vi "Interface.vi"() -> ()   [LabVIEW 2013]
uses:
  MeasureModeControl.ctl
  <vilib>/Utility/miscctls.llb/LVBoundsTypeDef.ctl
  GlobalVariables/LanguagesSettings.vi
  GlobalVariables/PreconfiguredSleeveData.vi
  GlobalVariables/CaptParameters.vi
  GlobalVariables/ValveParameters.vi
  GlobalVariables/MachineInfos.vi
  GlobalVariables/StabilizationSettings.vi
  GlobalVariables/CalibrationVolumes.vi
  GlobalVariables/HardwarePresent.vi
  GlobalVariables/ValveValues.vi
  GlobalVariables/AppState.vi
  GlobalVariables/PressureAndTimeSamples.vi
  GlobalVariables/CurrentPressure.vi
  GlobalVariables/CommunicationActivity.vi
  GlobalVariables/CalibrationState.vi
  GlobalVariables/FittedCurvePolynom.vi
  <vilib>/Utility/file.llb/Write To Spreadsheet File (string).vi
  <vilib>/Utility/file.llb/Read From Spreadsheet File (string).vi
  GlobalVariables/MeasureExportStrings.vi
  <vilib>/Utility/config.llb/Read Key (String).vi
  GlobalVariables/UserInfos.vi
  <vilib>/Utility/config.llb/NI_LVConfig.lvlib
panel:
  in  "DeleteMeasureLine":bool
  in  "ExportData":bool
  in  "LoadData":bool
  in  "SaveData":bool
  in  "ReloadResultTableTexts":bool
  in  "MeasureMode":T1
  in  "ReloadDiskVolumes":bool
  in  "StabilityAchieved":bool
  in  "UpdateServiceGraph":bool
  in  "ComputeCalibrationResult":bool
  in  "SingleCalibrationMeasureButtonsVisible":bool
  out "FirstGraphSampleIndex":i32
  in  "ServiceButtonsVisible":bool
  in  "ExportMeasuresButtonsVisible":bool
  in  "ChangeMenuState":bool
  in  "MeasureIndicatorsVisible":bool
  in  "MeasureSetupButtonsVisible":bool
  in  "CalibrationButtonsVisible":bool
  in  "CalibrationResultsVisible":bool
  in  "UserFilledDataChanged":bool
  out "NotificationTexts":string[](array[string])
  out "rPressionM":dbl caption="Pression courante" format="%#.1f bars"
  out "error out":errorcluster caption="sortie d'erreur"
  out "indicateurPerteSignal":bool caption="Perte du signal de pression"
  out "indicateurDefautPuissance":bool caption="Défaut de puissance"
  out "indicateurSurpression":bool caption="Surpression"
  in  "btnExit":bool
  out "vTimeDate":timestamp format="%<%.1X\n%x>T"
  out "strInstallName":string="INSTALL NAME"
  in  "AppTab":T2(tab) caption="Onglets1"
  out "presentationPicture":picture caption="Prêt"
  in  "MeasuresTabs":enum32{"Grain measures", "Pore measures"}(tab) caption="Measures"
  in  "LoadGrainMeasuresBtn":bool
  in  "SaveGrainMeasuresBtn":bool caption="SaveDataFileButton"
  in  "ExportGrainMeasuresBtn":bool caption="Exporter"
  in  "ClearGrainMeasuresBtn":bool caption="Clear measures table"
  out "grainMeasuresTable":string[][](table)=[["Date", "Numéro", "ID de l'échantillon", "Profondeur (coudées)", "Poids à sec (g)", "Volume de grain (cm3)", "Densité de grain (g/cm3)", "Volume de pore (cm3)", "Porosité (%)", "Volume de l'enveloppe (cm3)", "Longueur (cm)", "Diamètre (cm)", "Epaisseur (cm)", "Température (°C)", "Commentaires"]] caption="Résultats Mesures de grains"
  in  "ClearGrainMeasureBtn":bool
  in  "LoadPoreMeasuresBtn":bool
  in  "SavePoreMeasuresBtn":bool caption="SaveDataFileButton"
  in  "ExportPoreMeasuresBtn":bool caption="Exporter"
  out "poreMeasuresTable":string[][](table)=[["Date", "Numéro", "ID de l'échantillon", "Profondeur (coudées)", "Poids à sec (g)", "Volume de grain (cm3)", "Densité de grain (g/cm3)", "Volume de pore (cm3)", "Porosité (%)", "Volume de l'enveloppe (cm3)", "Longueur (cm)", "Diamètre (cm)", "Epaisseur (cm)", "Température (°C)", "Commentaires"]] caption="Résultats"
  in  "ClearPoreMeasuresBtn":bool caption="Clear measures table"
  in  "ClearPoreMeasureBtn":bool
  in  "btnMesureGrain":bool
  out "MeasureTotalAddedVolume":dbl caption="Volume total"
  in  "MeasureDiskSet":i32(listbox) caption="Jeu de disques"
  in  "MeasureDiskVolumes":i32[](listbox) caption="Volumes disponibles"
  in  "Comments":string caption="Commentaires"
  in  "Temperature":dbl caption="Température (°C)"
  in  "BulkVolume":dbl caption="Volume de grain (cm3)"
  in  "DryWeight":dbl caption="Poids à sec (g)"
  in  "SampleDepth":dbl caption="Profondeur (cm)"
  in  "SampleID":string caption="ID de l'échantillon"
  in  "SampleNumber":string caption="Numéro"
  in  "DoMeasureMeasure":bool caption="LaunchMeasureMeasure"
  in  "ReferenceCellMeasure":u16=1 caption="Cellule de référence" min=1 max=2
  in  "DiskSet":i32(listbox) caption="Jeu de disques"
  in  "RestartCalibration":bool
  out "CalibrationStep":u32 caption="Nombre de mesures effectuées"
  in  "CalibrationFilePath":path caption="Fichier de calibration"
  in  "LoadCalibrationFileBtn":bool
  in  "AvalaibleVolumesList":i32[](listbox) caption="Volumes disponibles"
  in  "ChosenVolume":dbl caption="Volume total"
  in  "DoMeasureCalibration":bool caption="DoCalibrationMeasure"
  in  "EndCalibration":bool caption="Finir la calibration"
  out "measureStabilization":string
  in  "P1P2RatioMeasure":dbl caption="P1/P2 ratio"
  out "MeasureReportedString":string
  out "VolumeMeasureInd":dbl caption="Volume de grain mesuré"
  out "calibrationStabilization":string
  in  "KeepCalibrationPoint":bool caption="Garder le point"
  out "VolumeOfCalibrationMeasure":dbl caption="Volume total"
  out "P1P2RatioCalibration":dbl caption="Rapport P1/P2"
  in  "ContinueCalibration":bool
  out "Correlation":dbl
  out "AverageAbsoluteDeviation":dbl caption="Deviation moyenne"
  in  "SaveCalibrationFile":bool caption="Save calibration file"
  out "ResidueInd":dbl caption="Résidu"
  out "FittedPolynomCoeffs":dbl[](array[numeric]) caption="Coefficient du polynome d'interpolation"
  in  "ExportToPDF":bool caption="Export to PDF"
  in  "ExportToHTMLBtn":bool
  in  "Client":string
  in  "Country":string caption="Pays"
  in  "Formation":string
  in  "LatitudeLongitude":string caption="Latitude/Longitude"
  in  "Operator":string caption="Opérateur"
  in  "Well":string caption="Puits"
  in  "Lab":string caption="Laboratoire"
  in  "Company":string caption="Entreprise"
  in  "Field":string caption="Champs"
  in  "Location":string caption="Lieu"
  out "PurgeState":string
  out "ValvesBoutonVisible":bool=TRUE caption="Sample valve"
  in  "FlushPressureGraph":bool
  in  "Sample ValveBtn":bool=TRUE caption="Sample valve"
  in  "V2Btn":bool=TRUE caption="V2"
  in  "V1Btn":bool=TRUE caption="V1"
  in  "Inlet ValveBtn":bool=TRUE caption="Inlet valve"
  in  "Outlet ValveBtn":bool=TRUE caption="Outlet valve"
  out "PressureGraph":T3(graph)
  out "Helium Tank":string caption="Bonbonne d'Hélium"
  out "NotificationArea":string
  out "Ref2":string caption="Référence 2"
  out "Matrix Cup":string caption="Echantillon"
  out "Ref1":string caption="Référence 1"
  in  "manualModeBtn":bool
  out "Outlet ValveInd":bool=TRUE caption="Valve de sortie"
  out "Sample ValveInd":bool=TRUE caption="Valve de l'échantillon"
  out "V2Ind":bool=TRUE caption="V2"
  out "V1Ind":bool=TRUE caption="V1"
  out "Inlet ValveInd":bool=TRUE caption="Valve d'entrée"
  out "vPressionM":dbl format="%#.1f bars"
  in  "btnVidanger":bool
  in  "btnEtal":bool
  in  "btnMesurePore":bool
  in  "MaximalWaitTime":u32 caption="Temps maximal d'attente (ms)"
  in  "VarianceTrigger":dbl caption="Variance minimale"
  in  "MinimalWaitTime":u32 caption="Temps minimal d'attente (ms)"
  in  "PressureCaptorConfig":T4 caption="Configuration du capteur"
  in  "mdpControl":string caption="Mot de passe"
  in  "SamplesMasks":bool[](array[boolean]) caption="Prise en compte point n°"
  in  "CalibrationVolumesTable":string[][](table) caption="Tableau des volumes de calibrations"
  out "AverageAbsoluteDeviationServices":dbl caption="Deviation moyenne"
  out "CorrelationServices":dbl caption="Correlation"
  out "ResiduServices":dbl caption="Résidu"
  out "FittedPolynomCoeffsServices":dbl[](array[numeric]) caption="Coefficient du polynome d'interpolation"
  out "XYGraphService":cluster{dbl[], dbl[]}[](graph)=[{[1.0, 2.0, 4.0], [2.0, 1.0, 0.0]}, {[0.5, 1.5, 3.5], [3.0, 4.0, 2.0]}] caption="Mesure et courbe d'étalonnage"
  out "pumeActive":bool caption="PUM-E actif"
  out "pressureCaptorActive":bool caption="Capteur de pression actif"
  in  "MachineName":string caption="Nom de la machine"
  in  "Pressure Gain":dbl=1.0 caption="Gain de pression"
  in  "Pressure Offset":dbl caption="Offset de pression"
  in  "Valve mapping":T5 caption="Mappage des valves"
  in  "LanguagesList":i32(listbox) caption="Langues disponibles"
  in  "SaveConfigChanges":bool caption="Save changes"
  in  "SleeveConfiguration":T6 caption="Configuration de la chemise"
  in  "ValvesConfig":T7 caption="Configuration des valves" {"Mode" items=["RTU", "ASCII"]}
  # "Stabilisation"
  # "Services"
  # "Transmission"
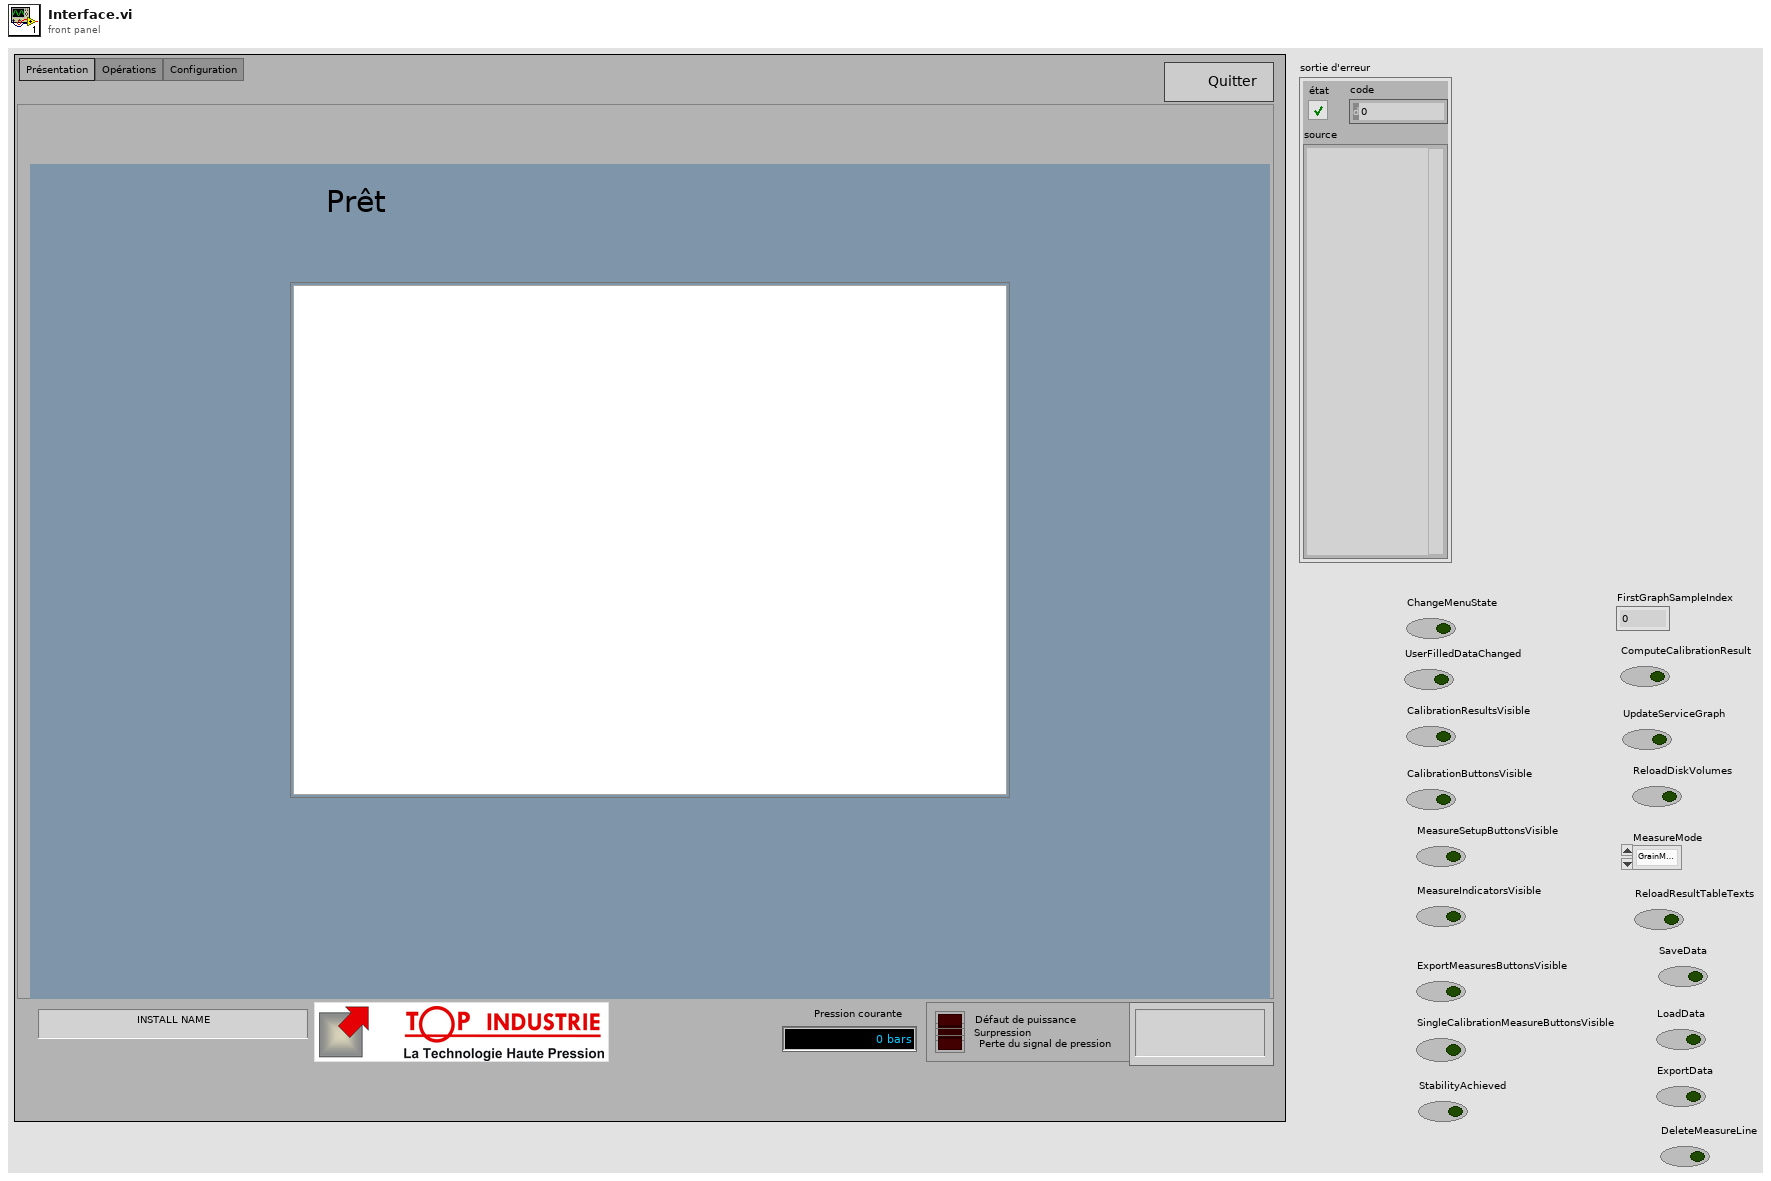
[diagram p1: front panel]
types:
  T1 = typedef "MeasureModeControl.ctl" = enum16{"GrainMeasure", "PoreMeasure"}
  T2 = enum32{"Présentation", "Opérations", "Configuration"}
  T3 = cluster{"TimeSamples":dbl[], "PressureSamples":dbl[]}
  T4 = cluster{"Baudrate":u32, "Port":string, "Databits":u16, "Parity":u16, "Stopbits":u16, "Flow Control":u16, "Slave Address":u16, "Register Address":u16, "Timeout (ms)":u16, "MaxCaptorPressure":dbl}
  T5 = cluster{"Inlet Valve":u8, "V1":u8, "V2":u8, "Sample Valve":u8, "Outlet Valve":u8}
  T6 = cluster{"Length (cm)":dbl, "Diameter (cm)":dbl, "Thickness (cm)":dbl}
  T7 = cluster{"Baudrate":u32, "Port":string, "Databits":u16, "Parity":u16, "Stopbits":u16, "Flow Control":u16, "Slave Address":u16, "Mode":u16, "Timeout (ms)":u16}
  T8 = enum8{"Enabled", "Disabled", "Disabled and Grayed Out"}
  T9 = cluster{bool, "CalibrationStep":u32, "Volumes":dbl[], "PressureRatios":dbl[], "Weights":bool[]}
  T10 = typedef "LVBoundsTypeDef.ctl" = cluster{"Width":u32, "Height":u32}
  T11 = cluster{"baudrate":u32, "databits":u16, "paritybit":u16, "stopbits":u16, "flux control":u16, "Port":string, "Serial Parameters":cluster{"Mode":enum16{"RTU", "ASCII"}, "Slave Address":u8}, "Timeout":u32, "Valve mapping":cluster{"Inlet Valve":u8, "V1":u8, "V2":u8, "Sample Valve":u8, "Outlet Valve":u8}}
  T12 = cluster{"baudrate":u32, "databits":u16, "paritybit":u16, "stopbits":u16, "flux control":u16, "Port":string, "Register Address":u16, "Serial Parameters":cluster{"Mode":enum16{"RTU", "ASCII"}, "Slave Address":u8}, "Timeout":u32, "PressureLimit":dbl}
  T13 = cluster{"SupportedLanguagesList":string[], "ActiveLanguage":string, "ActiveLanguageIndex":u16, "LocalisationFileContent[out]":cluster{"Indices":u32[], "LocalizedWords":string[][]}}
  T14 = cluster{"SerialNumber":string, "MachineName":string}
  T15 = cluster{"sleeveLength":dbl, "sleeveDiameter":dbl, "sleeveThickness":dbl}
  T16 = cluster{"baudrate":u32, "Port":string, "databits":u16, "paritybit":u16, "stopbits":u16, "flux control":u16, "Slave Address":u8, "Register Address":u16, "Timeout":u32, "PressureLimit":dbl}
  T17 = cluster{"baudrate":u32, "Port":string, "databits":u16, "paritybit":u16, "stopbits":u16, "flux control":u16, "Slave Address":u8, "Mode":enum16{"RTU", "ASCII"}, "Timeout":u32}
  T18 = cluster{"CalibrationVolumes":dbl[], "SetName":string, "DisplayedStrings":string[]}[]
  T19 = cluster{"MinimalWaitTime":u32, "VarianceTrigger":dbl, "MaxWaitTime":u32}
  T20 = typedef "imagedata.ctl" = cluster{"image type":i32, "image depth":i32, "image":u8[], "mask":u8[], "colors":u32[], "Rectangle":cluster{"left":i16, "top":i16, "right":i16, "bottom":i16}}
  T21 = cluster{"Indices":u32[], "LocalizedWords":string[][]}
  T22 = cluster{"SignalLoss":bool, "PumeActive":bool, "CaptorActive":bool}
  T23 = cluster{"CalibrationVolumes":dbl[], "SetName":string, "DisplayedStrings":string[]}
  T24 = cluster{"SampleNumber":string, "SampleID":string, "SampleDepth":dbl, "DryWeight":dbl, "BulkVolume":dbl, "Temperature":dbl, "Comments":string}
  T25 = cluster{"date":string, "sampleNumber":string, "sampleID":string, "sampleDepth":dbl, "dryWeight":dbl, "grainDensity":dbl, "bulk volume":dbl, "poreVolume":dbl, "porosity":dbl, "sleeveVolume":dbl, "sleeveLength":dbl, "sleeveDiameter":dbl, "sleeveThickness":dbl, "temperature":dbl, "comments":string}
  T26 = cluster{"NewVal":u32, "VarianceTrigger":dbl, "MaxWaitTime":u32}
  T27 = cluster{"MinimalWaitTime":u32, "NewVal":dbl, "MaxWaitTime":u32}
  T28 = cluster{"MinimalWaitTime":u32, "VarianceTrigger":dbl, "NewVal":u32}
  T29 = cluster{"Baudrate":u32, "Databits":u16, "Parity":u16, "Stopbits":u16, "Flow Control":u16, "Port":string, cluster{"Mode":u16, "Slave Address":u16}, "Timeout (ms)":u16, "Valve mapping":cluster{"Inlet Valve":u8, "V1":u8, "V2":u8, "Sample Valve":u8, "Outlet Valve":u8}}
  T30 = cluster{"Baudrate":u32, "Databits":u16, "Parity":u16, "Stopbits":u16, "Flow Control":u16, "Port":string, "Register Address":u16, cluster{u16, "Slave Address":u16}, "Timeout (ms)":u16, "MaxCaptorPressure":dbl}
  T31 = cluster{"SupportedLanguagesList":string[], "String":string, "LanguagesList":i32, "LocalisationFileContent[out]":cluster{"Indices":u32[], "LocalizedWords":string[][]}}
  T32 = typedef "NI_LVConfig.lvlib/Config Data RefNum.ctl" = refnum<k1>
  T33 = cluster{bool, u32, "Volumes":dbl[], "PressureRatios":dbl[], "Weights":bool[]}
  T34 = typedef "LVRowAndColumnTypeDef.ctl" = cluster{"Row":i32, "Column":i32}
  T35 = cluster{"location":string, "Field":string, "Company":string, "Lab":string, "Operator":string, "Well":string, "Lat/Long":string, "Formation":string, "Country":string, "Client":string}
  T36 = cluster{"NewVal":string, "Field":string, "Company":string, "Lab":string, "Operator":string, "Well":string, "Lat/Long":string, "Formation":string, "Country":string, "Client":string}
  T37 = cluster{"location":string, "NewVal":string, "Company":string, "Lab":string, "Operator":string, "Well":string, "Lat/Long":string, "Formation":string, "Country":string, "Client":string}
  T38 = cluster{"location":string, "Field":string, "NewVal":string, "Lab":string, "Operator":string, "Well":string, "Lat/Long":string, "Formation":string, "Country":string, "Client":string}
  T39 = cluster{"location":string, "Field":string, "Company":string, "NewVal":string, "Operator":string, "Well":string, "Lat/Long":string, "Formation":string, "Country":string, "Client":string}
  T40 = cluster{"location":string, "Field":string, "Company":string, "Lab":string, "NewVal":string, "Well":string, "Lat/Long":string, "Formation":string, "Country":string, "Client":string}
  T41 = cluster{"location":string, "Field":string, "Company":string, "Lab":string, "Operator":string, "NewVal":string, "Lat/Long":string, "Formation":string, "Country":string, "Client":string}
  T42 = cluster{"location":string, "Field":string, "Company":string, "Lab":string, "Operator":string, "Well":string, "NewVal":string, "Formation":string, "Country":string, "Client":string}
  T43 = cluster{"location":string, "Field":string, "Company":string, "Lab":string, "Operator":string, "Well":string, "Lat/Long":string, "NewVal":string, "Country":string, "Client":string}
  T44 = cluster{"location":string, "Field":string, "Company":string, "Lab":string, "Operator":string, "Well":string, "Lat/Long":string, "Formation":string, "NewVal":string, "Client":string}
  T45 = cluster{"location":string, "Field":string, "Company":string, "Lab":string, "Operator":string, "Well":string, "Lat/Long":string, "Formation":string, "Country":string, "NewVal":string}
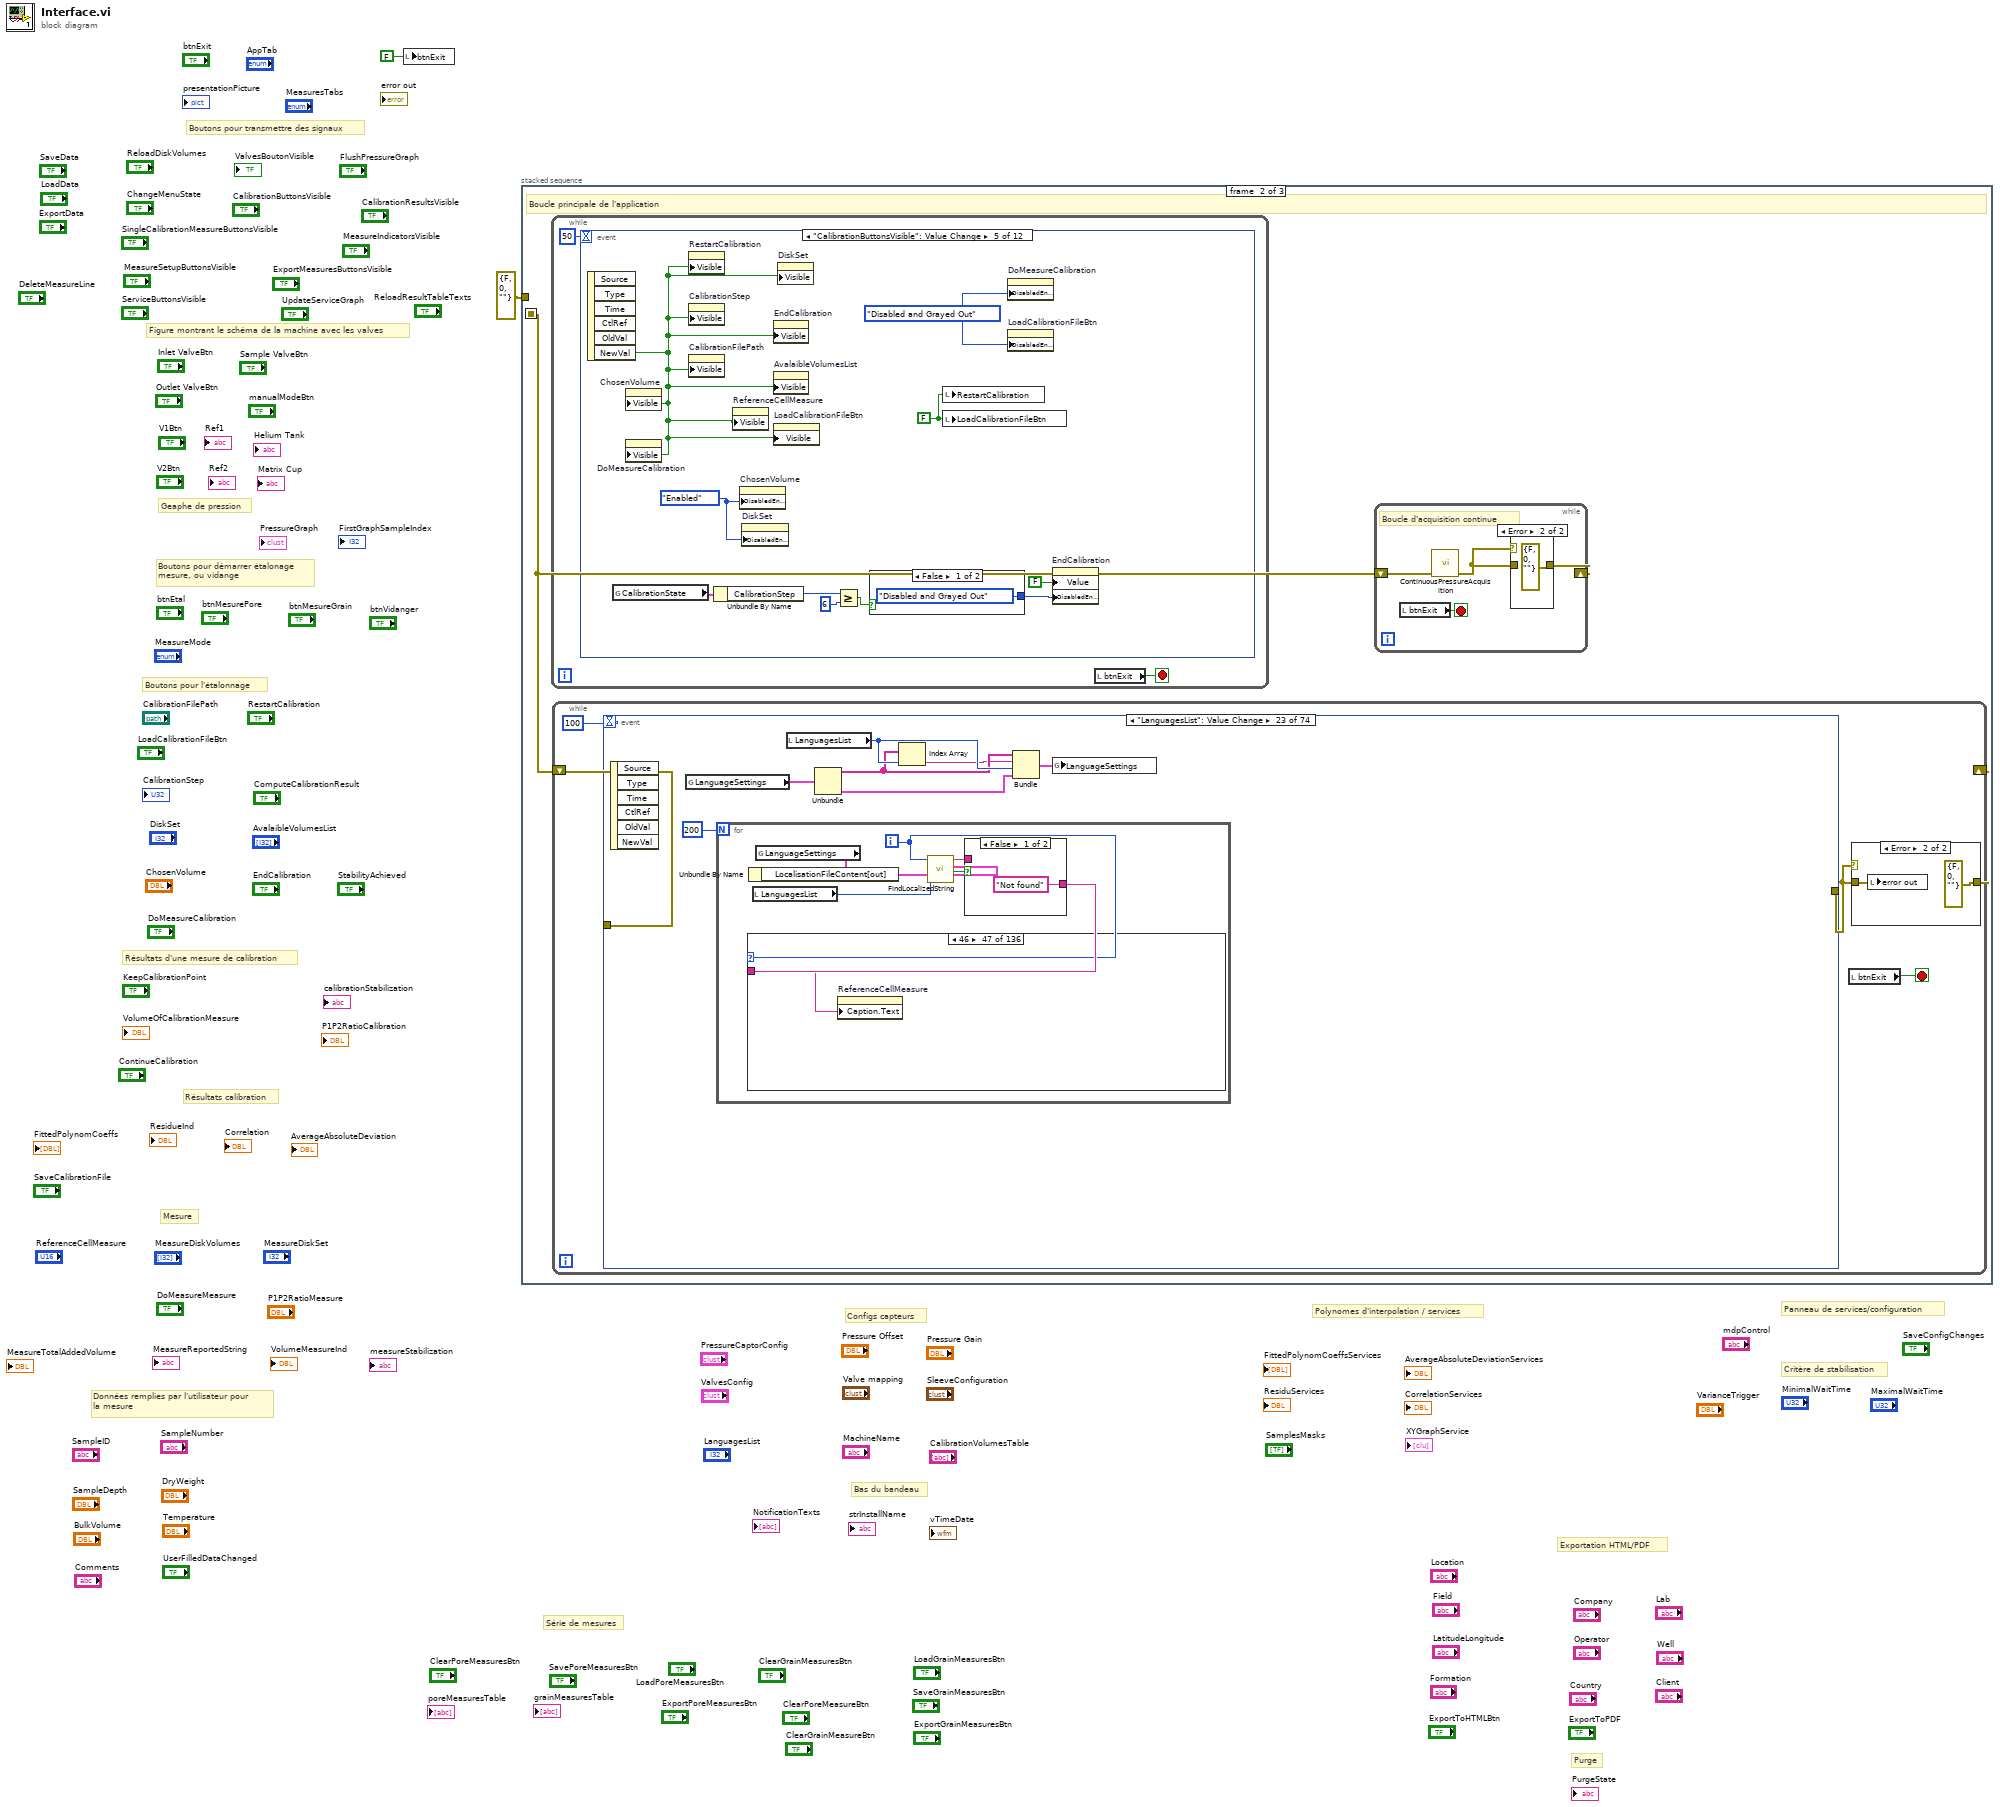
[diagram p0: block diagram]
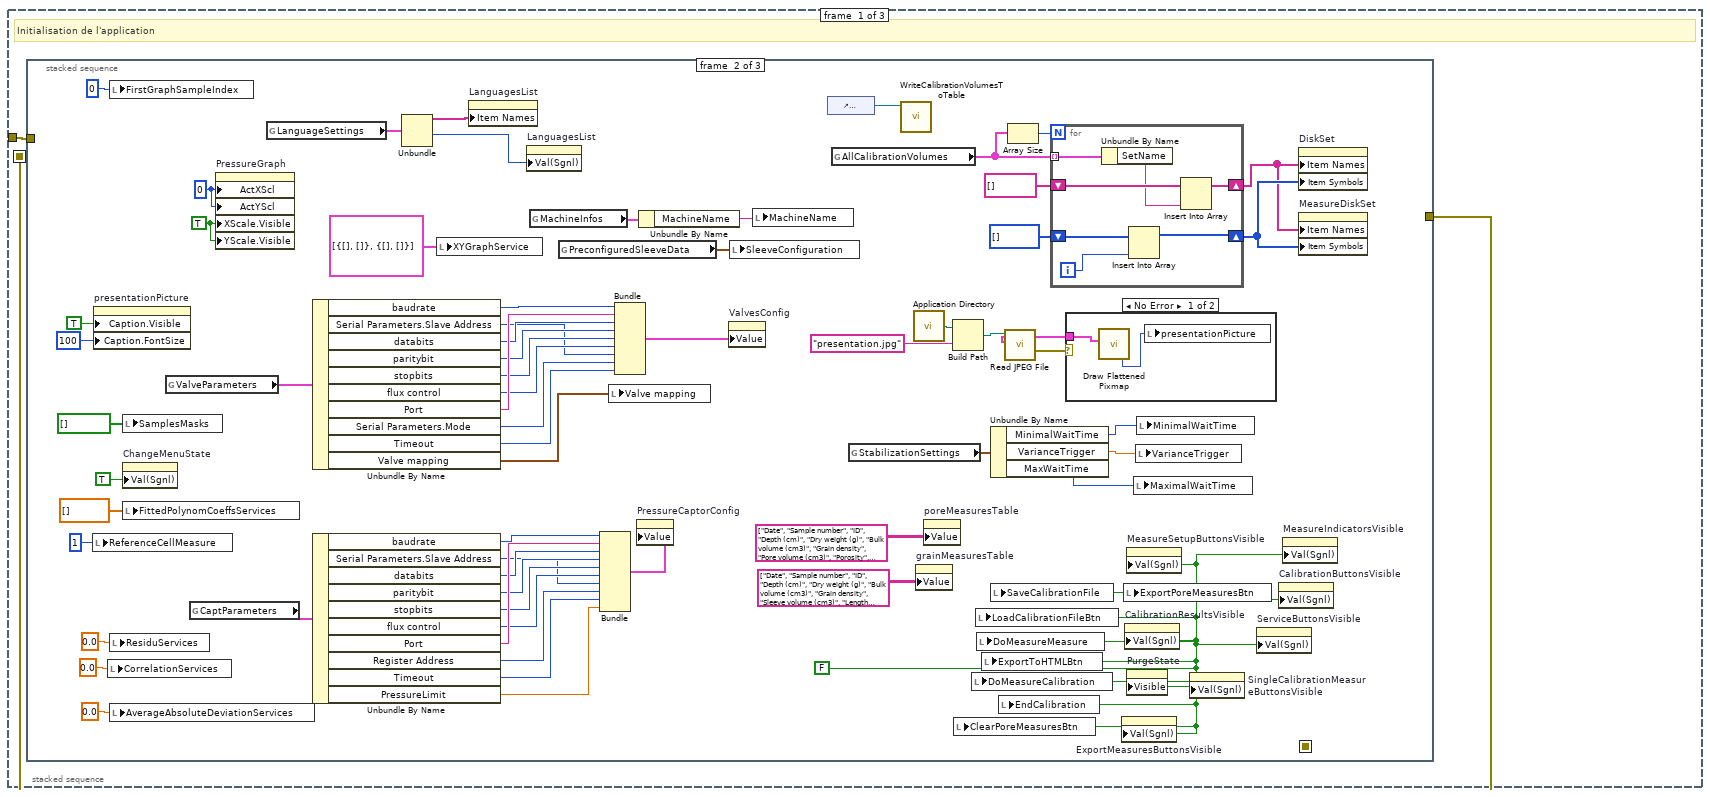
[diagram p2: hidden frame]
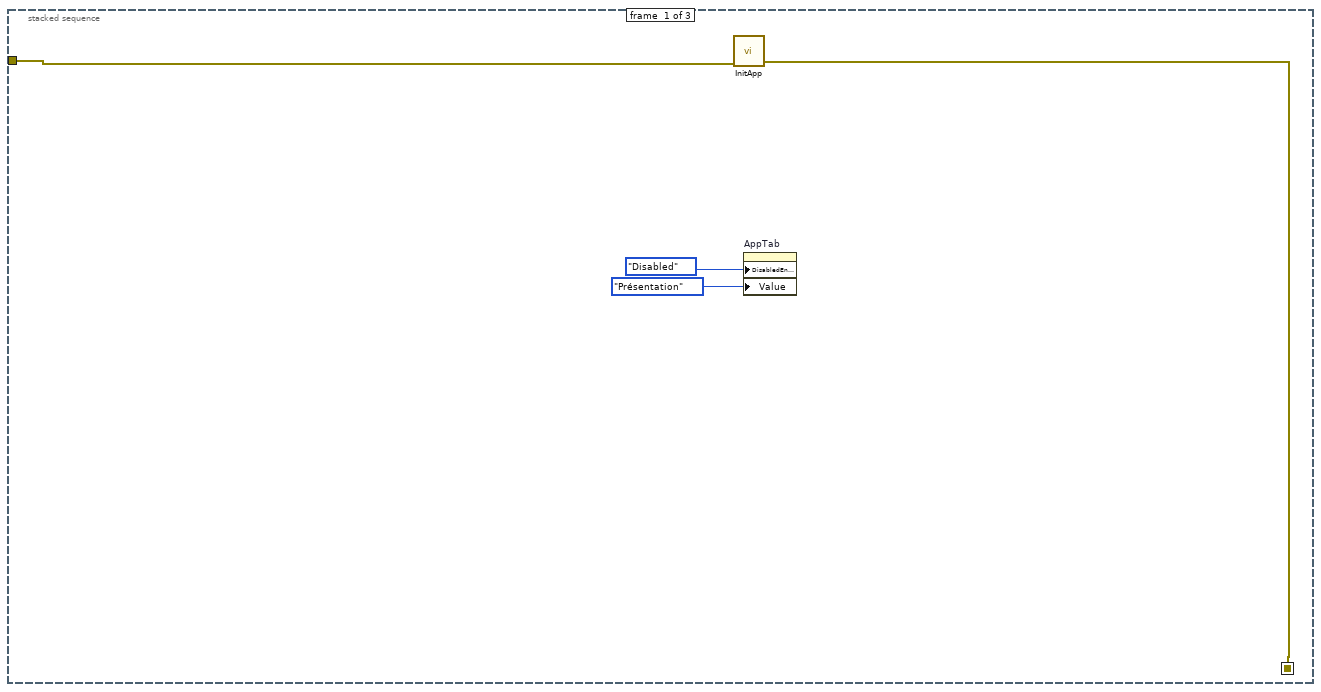
[diagram p3: hidden frame]
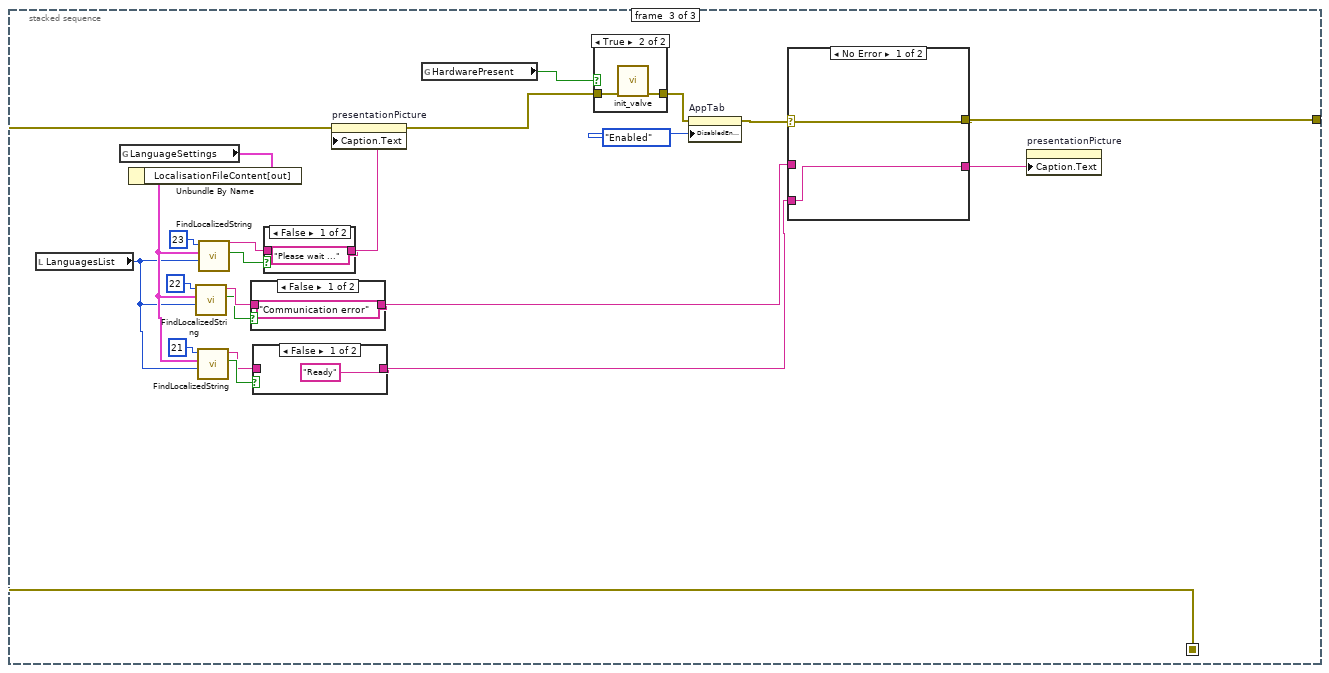
[diagram p5: hidden frame]
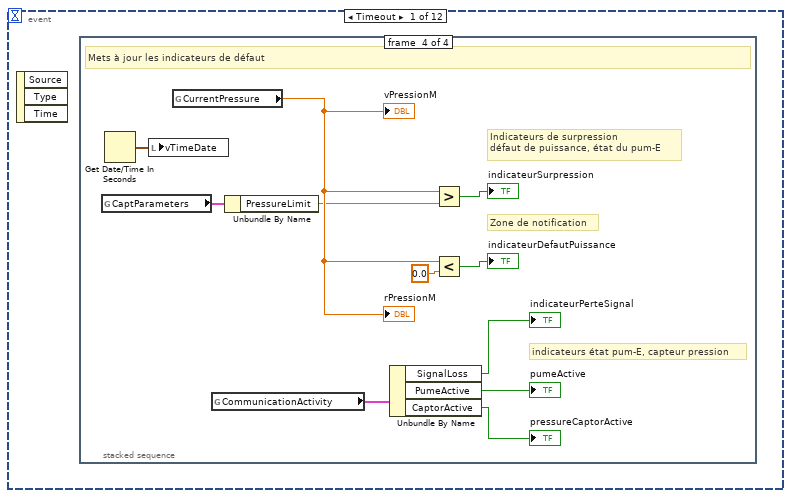
[diagram p12: hidden frame]
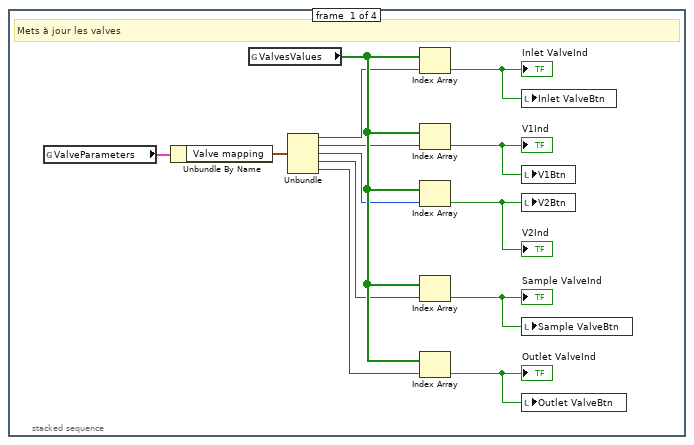
[diagram p13: hidden frame]
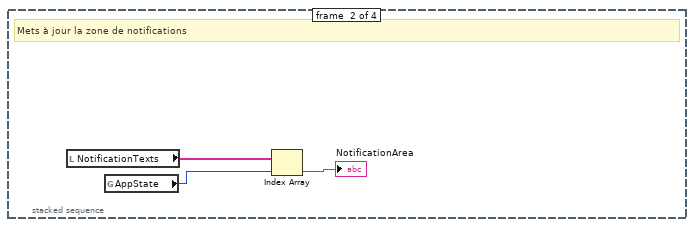
[diagram p14: hidden frame]
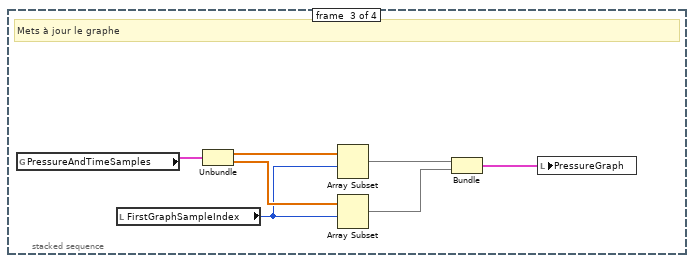
[diagram p15: hidden frame]
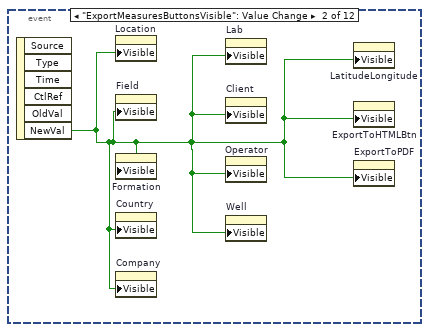
[diagram p16: hidden frame]
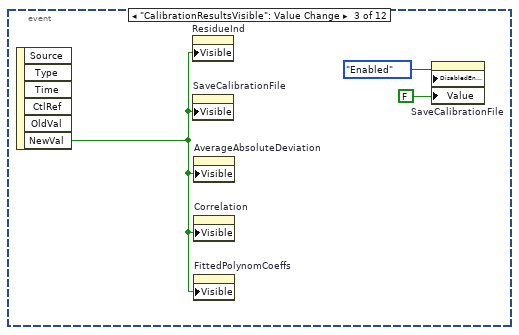
[diagram p17: hidden frame]
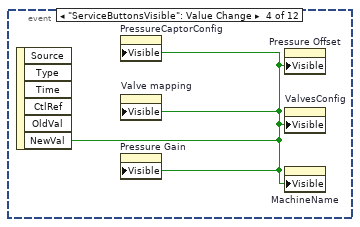
[diagram p18: hidden frame]
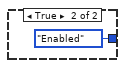
[diagram p19: hidden frame]
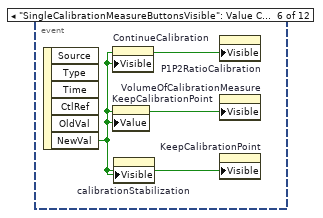
[diagram p20: hidden frame]
diagram:
  # "Boutons pour transmettre des signaux"
  # "Configs capteurs"
  # "Polynomes d'interpolation / services"
  # "Critère de stabilisation"
  # "Résultats d'une mesure de calibration"
  # "Geaphe de pression"
  # "Figure montrant le schéma de la machine avec les valves"
  # "Exportation HTML/PDF"
  # "Série de mesures"
  # "Données remplies par l'utilisateur pour \nla mesure"
  # "Panneau de services/configuration"
  # "Mesure"
  # "Résultats calibration"
  # "Purge"
  # "Boutons pour démarrer étalonage\nmesure, ou vidange"
  # "Bas du bandeau"
  # "Boutons pour l'étalonnage"
  n1 = local write "btnExit"(FALSE ("btnExit")) -> ()
  n2 = stacked-sequence {
    seq-local: [w3 _ _] -> [_ w116 _]
    tunnel: errorcluster {"status"=FALSE, "code"=0, "source"=""} ("error in") -> [w4 _ _]
    frame #0 {
      # "Initialisation de l'application"
      n3 = stacked-sequence {
        seq-local: [w5 _ _] -> [_ _ w80]
        tunnel: w4 -> [w8 _ _]
        tunnel: [_ _ w81] -> w3
        frame #0 {
          n4 = call "InitApp.vi"("error in"=w8) -> ("error out"=w5:errorcluster)  [unwired: 10 in]
          n5 = property on="AppTab" class="TabCtl (strict)"("DisabledEnum"=T8."Disabled" ("Disabled"), "Value"=T2."Présentation" ("Onglets1")) -> ()  [unwired: 2 in, 2 out]
        }
        frame #1 {
          w9 = TRUE ("X Scale.Visible")
          w10 = 0 ("Active X Scale")
          w32 = FALSE ("Visible")
          n6 = local write "ReferenceCellMeasure"(u16 1 ("ReferenceCellMeasure")) -> ()
          n7 = property on="presentationPicture" class="Pict"("Caption.Visible"=TRUE, "Caption.FontSize"=100) -> ()  [unwired: 2 in, 2 out]
          n8 = local write "CorrelationServices"(0.0 ("CorrelationServices")) -> ()
          n9 = local write "FirstGraphSampleIndex"(u32 0 ("FirstGraphSampleIndex")) -> ()
          n10 = local write "ResiduServices"(0.0 ("ResiduServices")) -> ()
          n11 = local write "AverageAbsoluteDeviationServices"(0.0 ("AverageAbsoluteDeviationServices")) -> ()
          n12 = local write "SamplesMasks"(bool[] [] ("SamplesMasks")) -> ()
          n13 = property on="ChangeMenuState" class="Bool (strict)"("Val(Sgnl)"=TRUE ("Value (Signaling)")) -> ()  [unwired: 2 in, 2 out]
          n14 = local write "FittedPolynomCoeffsServices"(dbl[] [] ("FittedPolynomCoeffsServices")) -> ()
          n15 = global read "ValveParameters.vi" "ValveParameters"() -> (w46:T11)
          n16 = global read "CaptParameters.vi" "CaptParameters"() -> (w65:T12)
          n17 = property on="PressureGraph" class="XYGraph (strict)"("ActXScl"=w10, "ActYScl"=w10, "XScale.Visible"=w9, "YScale.Visible"=w9) -> ()  [unwired: 2 in, 2 out]
          n18 = global read "LanguagesSettings.vi" "LanguageSettings"() -> (w69:T13)
          n19 = Unbundle By Name(w46) -> ("baudrate"=w55:u32, "Serial Parameters.Slave Address"=w49:u8, "databits"=w53:u16, "paritybit"=w52:u16, "stopbits"=w51:u16, "flux control"=w50:u16, "Port"=w54:string, "Serial Parameters.Mode"=w48:enum16{"RTU", "ASCII"}, "Timeout"=w47:u32, "Valve mapping"=w43:T5)
          n20 = Unbundle By Name(w65) -> ("baudrate"=w64:u32, "Serial Parameters.Slave Address"=w58:u8, "databits"=w62:u16, "paritybit"=w61:u16, "stopbits"=w60:u16, "flux control"=w59:u16, "Port"=w63:string, "Register Address"=w57:u16, "Timeout"=w56:u32, "PressureLimit"=w25:dbl)
          n21 = Unbundle(w69) -> ("SupportedLanguagesList"=w67:string[], "ActiveLanguageIndex"=w66:u16)  [unwired: 2 out]
          n22 = local write "XYGraphService"(cluster{dbl[], dbl[]}[] [{[], []}, {[], []}] ("XYGraphService")) -> ()
          n23 = property on="LanguagesList" class="LstBox (strict)"("Item Names"=w67) -> ()  [unwired: 2 in, 2 out]
          n24 = property on="LanguagesList" class="LstBox (strict)"("Val(Sgnl)"=w66) -> ()  [unwired: 2 in, 2 out]
          n25 = global read "MachineInfos.vi" "MachineInfos"() -> (w24:T14)
          n26 = global read "PreconfiguredSleeveData.vi" "PreconfiguredSleeveData"() -> (w68:T15)
          n27 = Bundle("baudrate"=w64, "Port"=w63, "databits"=w62, "paritybit"=w61, "stopbits"=w60, "flux control"=w59, "Slave Address"=w58, "Register Address"=w57, "Timeout"=w56, "PressureLimit"=w25) -> (w45:T16)  [unwired: 1 in]
          n28 = local write "Valve mapping"(w43) -> ()
          n29 = Bundle("baudrate"=w55, "Port"=w54, "databits"=w53, "paritybit"=w52, "stopbits"=w51, "flux control"=w50, "Slave Address"=w49, "Mode"=w48, "Timeout"=w47) -> (w44:T17)  [unwired: 1 in]
          n30 = property on="PressureCaptorConfig" class="Clust (strict)"("Value"=w45) -> ()  [unwired: 2 in, 2 out]
          n31 = Unbundle By Name(w24) -> ("MachineName"=w23:string)
          n32 = property on="ValvesConfig" class="Clust (strict)"("Value"=w44) -> ()  [unwired: 2 in, 2 out]
          n33 = local write "SleeveConfiguration"(w68) -> ()
          n34 = local write "MachineName"(w23) -> ()
          n35 = control-ref of="CalibrationVolumesTable"() -> (w38:refnum<vi>)
          n36 = global read "CalibrationVolumes.vi" "AllCalibrationVolumes"() -> (w16:T18)
          n37 = global read "StabilizationSettings.vi" "StabilizationSettings"() -> (w22:T19)
          n38 = call "WriteCalibrationVolumesToTable.vi"("Table in"=w38) -> ()  [unwired: 11 in]
          n39 = call <vilib>:"Application Directory.vi"() -> ("Application Directory"=w42:path)
          n40 = property on="grainMeasuresTable" class="Tbl (strict)"("Value"=string[][] [["Date", "Sample number", "ID", "Depth (cm)", "Dry weight (g)", "Bulk volume (cm3)", "Grain density", "Sleeve volume (cm3)", "Length (cm)", "Diameter (cm)", "Thickness (cm)", "Temperature (°C)", "Comments"]] ("measuresTable")) -> ()  [unwired: 2 in, 2 out]
          n41 = property on="poreMeasuresTable" class="Tbl (strict)"("Value"=string[][] [["Date", "Sample number", "ID", "Depth (cm)", "Dry weight (g)", "Bulk volume (cm3)", "Grain density", "Pore volume (cm3)", "Porosity", "Sleeve volume (cm3)", "Length (cm)", "Diameter (cm)", "Thickness (cm)", "Temperature (°C)", "Comments"]] ("measuresTable")) -> ()  [unwired: 2 in, 2 out]
          n42 = Build Path(base path=w42, name or relative path="presentation.jpg") -> (appended path=w41:path)
          n43 = local write "ClearPoreMeasuresBtn"(w32) -> ()
          n44 = local write "DoMeasureCalibration"(w32) -> ()
          n45 = local write "LoadCalibrationFileBtn"(w32) -> ()
          n46 = local write "DoMeasureMeasure"(w32) -> ()
          n47 = local write "ExportToHTMLBtn"(w32) -> ()
          n48 = Unbundle By Name(w22) -> ("MinimalWaitTime"=w21:u32, "VarianceTrigger"=w20:dbl, "MaxWaitTime"=w19:u32)
          n49 = local write "SaveCalibrationFile"(w32) -> ()
          n50 = local write "EndCalibration"(w32) -> ()
          n51 = call <vilib>:"Read JPEG File.vi"("path to JPEG file"=w41) -> ("error out"=w39:errorcluster, "image data"=w40:T20)  [unwired: 8 in, 1 out]
          n52 = Array Size(array=w16) -> (size(s)=w17:i32)
          n53 = for {
            N: w17 -> [_]
            shift-right: [w76] -> w13
            shift-left: string[] [] -> [w77]
            tunnel: w16 -> [w75] mode=indexing
            shift-right: [w71] -> w14
            shift-left: i32[] [] -> [w73]
            i -> [w72]
            n54 = Unbundle By Name(w75) -> ("SetName"=w74:string)
            n55 = Insert Into Array(array=w73, new element=w72) -> (w71:i32[])  [unwired: 1 in]
            n56 = Insert Into Array(array=w77, new element=w74) -> (w76:string[])  [unwired: 1 in]
          }
          n57 = case shown="No Error" w39 {
            tunnel: w40 -> [w79 _]
            frame No Error {
              n58 = call <vilib>:"Draw Flattened Pixmap.vi"("image data"=w79) -> ("new picture"=w78:picture)  [unwired: 8 in]
              n59 = local write "presentationPicture"(w78) -> ()
            }
            frame Error {
            }
          }
          n60 = property on="ExportMeasuresButtonsVisible" class="Bool (strict)"("Val(Sgnl)"=w32) -> ()  [unwired: 2 in, 2 out]
          n61 = local write "ExportPoreMeasuresBtn"(w32) -> ()
          n62 = property on="CalibrationResultsVisible" class="Bool (strict)"("Val(Sgnl)"=w32) -> ()  [unwired: 2 in, 2 out]
          n63 = property on="MeasureSetupButtonsVisible" class="Bool (strict)"("Val(Sgnl)"=w32) -> ()  [unwired: 2 in, 2 out]
          n64 = property on="PurgeState" class="Str"("Visible"=w32) -> ()  [unwired: 2 in, 2 out]
          n65 = local write "MaximalWaitTime"(w19) -> ()
          n66 = local write "VarianceTrigger"(w20) -> ()
          n67 = local write "MinimalWaitTime"(w21) -> ()
          n68 = property on="SingleCalibrationMeasureButtonsVisible" class="Bool (strict)"("Val(Sgnl)"=w32) -> ()  [unwired: 2 in, 2 out]
          n69 = property on="ServiceButtonsVisible" class="Bool (strict)"("Val(Sgnl)"=w32) -> ()  [unwired: 2 in, 2 out]
          n70 = property on="CalibrationButtonsVisible" class="Bool (strict)"("Val(Sgnl)"=w32) -> ()  [unwired: 2 in, 2 out]
          n71 = property on="MeasureIndicatorsVisible" class="Bool (strict)"("Val(Sgnl)"=w32) -> ()  [unwired: 2 in, 2 out]
          n72 = property on="DiskSet" class="LstBox (strict)"("Item Names"=w13, "Item Symbols"=w14) -> ()  [unwired: 2 in, 2 out]
          n73 = property on="MeasureDiskSet" class="LstBox (strict)"("Item Names"=w13, "Item Symbols"=w14) -> ()  [unwired: 2 in, 2 out]
        }
        frame #2 {
          n74 = local read "LanguagesList"() -> (w99:i32)
          n75 = global read "LanguagesSettings.vi" "LanguageSettings"() -> (w85:T13)
          n76 = Unbundle By Name(w85) -> ("LocalisationFileContent[out]"=w100:T21)
          n77 = call "FindLocalizedString.vi"("LangIndex"=w99, "LocalizationFileContent"=w100, "WordIndex"=22) -> ("Found"=w89:bool, "LocalizedString"=w90:string)  [unwired: 7 in]
          n78 = call "FindLocalizedString.vi"("LangIndex"=w99, "LocalizationFileContent"=w100, "WordIndex"=21) -> ("Found"=w97:bool, "LocalizedString"=w96:string)  [unwired: 7 in]
          n79 = call "FindLocalizedString.vi"("LangIndex"=w99, "LocalizationFileContent"=w100, "WordIndex"=23) -> ("Found"=w92:bool, "LocalizedString"=w93:string)  [unwired: 7 in]
          n80 = case shown="False" w89 {
            tunnel: w90 -> [_ w111]
            tunnel: ["Communication error" w111] -> w91
            frame False {
            }
            frame True {
            }
          }
          n81 = case shown="False" w97 {
            tunnel: w96 -> [_ w104]
            tunnel: ["Ready" w104] -> w101
            frame False {
            }
            frame True {
            }
          }
          n82 = case shown="False" w92 {
            tunnel: w93 -> [_ w109]
            tunnel: ["Please wait ..." w109] -> w94
            frame False {
            }
            frame True {
            }
          }
          n83 = property on="presentationPicture" class="Pict"(error in=w80, "Caption.Text"=w94) -> (error out=w88:errorcluster)  [unwired: 1 in, 1 out]
          n84 = global read "HardwarePresent.vi" "HardwarePresent"() -> (w102:bool)
          n85 = case shown="True" w102 {
            tunnel: [w105 w107] -> w84
            tunnel: w88 -> [w105 w106]
            frame False {
            }
            frame True {
              n86 = call "init_valve.vi"("error in"=w106) -> ("error out"=w107:errorcluster)  [unwired: 10 in]
            }
          }
          n87 = property on="AppTab" class="TabCtl (strict)"(error in=w84, "DisabledEnum"=T8."Enabled" ("Disabled")) -> (error out=w83:errorcluster)  [unwired: 1 in, 1 out]
          n88 = case shown="No Error" w83 {
            selector: w83 -> [w113 w115]
            tunnel: [w113 w115] -> w81
            tunnel: w91 -> [_ w114]
            tunnel: [w112 w114] -> w95
            tunnel: w101 -> [w112 _]
            frame No Error {
            }
            frame Error {
            }
          }
          n89 = property on="presentationPicture" class="Pict"("Caption.Text"=w95) -> ()  [unwired: 2 in, 2 out]
        }
      }
    }
    frame #1 {
      # "Boucle principale de l'application"
      n90 = while {
        stop <- w123 stop-if-true
        n91 = event shown="[4] \"CalibrationButtonsVisible\": Value Change" {
          selector: _ -> [_ _ _ _ _ _ _ _ _ _ _ _]
          dyn-events: _ -> [_ _ _ _ _ _ _ _ _ _ _ _]
          timeout: 50 -> [_ _ _ _ _ _ _ _ _ _ _ _]
          event Timeout {
            n92 = event-data() -> ()  [unwired: 1 in, 3 out]
            n93 = stacked-sequence {
              frame #0 {
                # "Mets à jour les valves"
                n94 = global read "ValveParameters.vi" "ValveParameters"() -> (w131:T11)
                n95 = Unbundle By Name(w131) -> ("Valve mapping"=w130:T5)
                n96 = global read "ValveValues.vi" "ValvesValues"() -> (w137:bool[])
                n97 = Unbundle(w130) -> ("Inlet Valve"=w125:u8, "V1"=w129:u8, "V2"=w128:u8, "Sample Valve"=w127:u8, "Outlet Valve"=w126:u8)
                n98 = Index Array(array=w137, index=w125) -> (element=w135:bool)
                "Inlet ValveInd" <- w135
                n99 = Index Array(array=w137, index=w129) -> (element=w133:bool)
                "V1Ind" <- w133
                n100 = Index Array(array=w137, index=w128) -> (element=w136:bool)
                "V2Ind" <- w136
                n101 = Index Array(array=w137, index=w127) -> (element=w134:bool)
                "Sample ValveInd" <- w134
                n102 = Index Array(array=w137, index=w126) -> (element=w132:bool)
                "Outlet ValveInd" <- w132
                n103 = local write "Inlet ValveBtn"(w135) -> ()
                n104 = local write "V1Btn"(w133) -> ()
                n105 = local write "V2Btn"(w136) -> ()
                n106 = local write "Sample ValveBtn"(w134) -> ()
                n107 = local write "Outlet ValveBtn"(w132) -> ()
              }
              frame #1 {
                # "Mets à jour la zone de notifications"
                n108 = local read "NotificationTexts"() -> (w138:string[])
                n109 = global read "AppState.vi" "AppState"() -> (w140:u16)
                n110 = Index Array(array=w138, index=w140) -> (element=→"NotificationArea":string)
              }
              frame #2 {
                # "Mets à jour le graphe"
                n111 = global read "PressureAndTimeSamples.vi" "PressureAndTimeSamples"() -> (w147:T3)
                n112 = local read "FirstGraphSampleIndex"() -> (w143:i32)
                n113 = Unbundle(w147) -> ("TimeSamples"=w145:dbl[], "PressureSamples"=w144:dbl[])
                n114 = Array Subset(array=w145, index=w143) -> (w142:dbl[])  [unwired: 1 in]
                n115 = Array Subset(array=w144, index=w143) -> (w141:dbl[])  [unwired: 1 in]
                n116 = Bundle(w142, w141) -> (w146:cluster{dbl[], dbl[]})  [unwired: 1 in]
                n117 = local write "PressureGraph"(w146) -> ()
              }
              frame #3 {
                # "indicateurs état pum-E, capteur pression"
                # "Indicateurs de surpression\ndéfaut de puissance, état du pum-E"
                # "Zone de notification"
                # "Mets à jour les indicateurs de défaut"
                n118 = global read "CaptParameters.vi" "CaptParameters"() -> (w150:T12)
                n119 = Get Date/Time In Seconds() -> (seconds since 1Jan1904=w148:timestamp)
                n120 = local write "vTimeDate"(w148) -> ()
                n121 = global read "CurrentPressure.vi" "CurrentPressure"() -> (w151:dbl)
                "vPressionM" <- w151
                "rPressionM" <- w151
                n122 = global read "CommunicationActivity.vi" "CommunicationActivity"() -> (w158:T22)
                n123 = Unbundle By Name(w150) -> ("PressureLimit"=w149:dbl)
                n124 = Unbundle By Name(w158) -> ("SignalLoss"=→"indicateurPerteSignal":bool, "PumeActive"=→"pumeActive":bool, "CaptorActive"=→"pressureCaptorActive":bool)
                n125 = Greater?(x=w151, y=w149) -> (0:→"indicateurSurpression":bool)
                n126 = Less?(x=w151, y=0.0) -> (x < y?=→"indicateurDefautPuissance":bool)
              }
            }
          }
          event "ExportMeasuresButtonsVisible": Value Change {
            n127 = event-data() -> ("NewVal"=w159:bool)  [unwired: 1 in, 5 out]
            n128 = property on="Location" class="Str"("Visible"=w159) -> ()  [unwired: 2 in, 2 out]
            n129 = property on="Field" class="Str"("Visible"=w159) -> ()  [unwired: 2 in, 2 out]
            n130 = property on="Formation" class="Str"("Visible"=w159) -> ()  [unwired: 2 in, 2 out]
            n131 = property on="Country" class="Str"("Visible"=w159) -> ()  [unwired: 2 in, 2 out]
            n132 = property on="Company" class="Str"("Visible"=w159) -> ()  [unwired: 2 in, 2 out]
            n133 = property on="Lab" class="Str"("Visible"=w159) -> ()  [unwired: 2 in, 2 out]
            n134 = property on="Client" class="Str"("Visible"=w159) -> ()  [unwired: 2 in, 2 out]
            n135 = property on="Operator" class="Str"("Visible"=w159) -> ()  [unwired: 2 in, 2 out]
            n136 = property on="Well" class="Str"("Visible"=w159) -> ()  [unwired: 2 in, 2 out]
            n137 = property on="LatitudeLongitude" class="Str"("Visible"=w159) -> ()  [unwired: 2 in, 2 out]
            n138 = property on="ExportToHTMLBtn" class="Bool (strict)"("Visible"=w159) -> ()  [unwired: 2 in, 2 out]
            n139 = property on="ExportToPDF" class="Bool (strict)"("Visible"=w159) -> ()  [unwired: 2 in, 2 out]
          }
          event "CalibrationResultsVisible": Value Change {
            n140 = event-data() -> ("NewVal"=w161:bool)  [unwired: 1 in, 5 out]
            n141 = property on="ResidueInd" class="DigNum (strict)"("Visible"=w161) -> ()  [unwired: 2 in, 2 out]
            n142 = property on="SaveCalibrationFile" class="Bool (strict)"("Visible"=w161) -> ()  [unwired: 2 in, 2 out]
            n143 = property on="AverageAbsoluteDeviation" class="DigNum (strict)"("Visible"=w161) -> ()  [unwired: 2 in, 2 out]
            n144 = property on="Correlation" class="DigNum (strict)"("Visible"=w161) -> ()  [unwired: 2 in, 2 out]
            n145 = property on="FittedPolynomCoeffs" class="Arr (strict)"("Visible"=w161) -> ()  [unwired: 2 in, 2 out]
            n146 = property on="SaveCalibrationFile" class="Bool (strict)"("DisabledEnum"=T8."Enabled" ("Disabled"), "Value"=FALSE ("SaveCalibrationFile")) -> ()  [unwired: 2 in, 2 out]
          }
          event "ServiceButtonsVisible": Value Change {
            n147 = event-data() -> ("NewVal"=w163:bool)  [unwired: 1 in, 5 out]
            n148 = property on="PressureCaptorConfig" class="Clust (strict)"("Visible"=w163) -> ()  [unwired: 2 in, 2 out]
            n149 = property on="Valve mapping" class="Clust (strict)"("Visible"=w163) -> ()  [unwired: 2 in, 2 out]
            n150 = property on="Pressure Gain" class="DigNum (strict)"("Visible"=w163) -> ()  [unwired: 2 in, 2 out]
            n151 = property on="Pressure Offset" class="DigNum (strict)"("Visible"=w163) -> ()  [unwired: 2 in, 2 out]
            n152 = property on="ValvesConfig" class="Clust (strict)"("Visible"=w163) -> ()  [unwired: 2 in, 2 out]
            n153 = property on="MachineName" class="Str"("Visible"=w163) -> ()  [unwired: 2 in, 2 out]
          }
          event "CalibrationButtonsVisible": Value Change {
            w166 = FALSE ("RestartCalibration")
            w165 = T8."Enabled" ("Disabled")
            w173 = T8."Disabled and Grayed Out" ("Disabled")
            n154 = event-data() -> ("NewVal"=w164:bool)  [unwired: 1 in, 5 out]
            n155 = global read "CalibrationState.vi" "CalibrationState"() -> (w167:T9)
            n156 = property on="ChosenVolume" class="DigNum (strict)"("Visible"=w164) -> ()  [unwired: 2 in, 2 out]
            n157 = property on="DoMeasureCalibration" class="Bool (strict)"("Visible"=w164) -> ()  [unwired: 2 in, 2 out]
            n158 = property on="RestartCalibration" class="Bool (strict)"("Visible"=w164) -> ()  [unwired: 2 in, 2 out]
            n159 = property on="CalibrationStep" class="DigNum (strict)"("Visible"=w164) -> ()  [unwired: 2 in, 2 out]
            n160 = property on="CalibrationFilePath" class="Path"("Visible"=w164) -> ()  [unwired: 2 in, 2 out]
            n161 = Unbundle By Name(w167) -> ("CalibrationStep"=w168:u32)
            n162 = property on="ReferenceCellMeasure" class="DigNum (strict)"("Visible"=w164) -> ()  [unwired: 2 in, 2 out]
            n163 = property on="ChosenVolume" class="DigNum (strict)"("DisabledEnum"=w165) -> ()  [unwired: 2 in, 2 out]
            n164 = property on="DiskSet" class="LstBox (strict)"("DisabledEnum"=w165) -> ()  [unwired: 2 in, 2 out]
            n165 = property on="EndCalibration" class="Bool (strict)"("Visible"=w164) -> ()  [unwired: 2 in, 2 out]
            n166 = property on="AvalaibleVolumesList" class="LstBox (strict)"("Visible"=w164) -> ()  [unwired: 2 in, 2 out]
            n167 = property on="LoadCalibrationFileBtn" class="Bool (strict)"("Visible"=w164) -> ()  [unwired: 2 in, 2 out]
            n168 = property on="DiskSet" class="LstBox (strict)"("Visible"=w164) -> ()  [unwired: 2 in, 2 out]
            n169 = Greater Or Equal?(x=w168, y=u32 6) -> (x >= y?=w170:bool)
            n170 = case shown="False" w170 {
              tunnel: [T8."Disabled and Grayed Out" ("Disabled") T8."Enabled" ("Disabled")] -> w171
              frame False {
              }
              frame True {
              }
            }
            n171 = local write "RestartCalibration"(w166) -> ()
            n172 = local write "LoadCalibrationFileBtn"(w166) -> ()
            n173 = property on="DoMeasureCalibration" class="Bool (strict)"("DisabledEnum"=w173) -> ()  [unwired: 2 in, 2 out]
            n174 = property on="LoadCalibrationFileBtn" class="Bool (strict)"("DisabledEnum"=w173) -> ()  [unwired: 2 in, 2 out]
            n175 = property on="EndCalibration" class="Bool (strict)"("Value"=FALSE ("EndCalibration"), "DisabledEnum"=w171) -> ()  [unwired: 2 in, 2 out]
          }
          event "SingleCalibrationMeasureButtonsVisible": Value Change {
            n176 = event-data() -> ("NewVal"=w176:bool)  [unwired: 1 in, 5 out]
            n177 = property on="ContinueCalibration" class="Bool (strict)"("Visible"=w176) -> ()  [unwired: 2 in, 2 out]
            n178 = property on="KeepCalibrationPoint" class="Bool (strict)"("Value"=w176) -> ()  [unwired: 2 in, 2 out]
            n179 = property on="calibrationStabilization" class="Str"("Visible"=w176) -> ()  [unwired: 2 in, 2 out]
            n180 = property on="P1P2RatioCalibration" class="DigNum (strict)"("Visible"=w176) -> ()  [unwired: 2 in, 2 out]
            n181 = property on="VolumeOfCalibrationMeasure" class="DigNum (strict)"("Visible"=w176) -> ()  [unwired: 2 in, 2 out]
            n182 = property on="KeepCalibrationPoint" class="Bool (strict)"("Visible"=w176) -> ()  [unwired: 2 in, 2 out]
          }
          event "ChangeMenuState": Value Change {
            n183 = event-data() -> ()  [unwired: 1 in, 6 out]
            n184 = global read "AppState.vi" "AppState"() -> (w183:u16)
            n185 = global read "CalibrationState.vi" "CalibrationState"() -> (w179:T9)
            n186 = global read "AppState.vi" "AppState"() -> (w201:u16)
            n187 = global read "CalibrationState.vi" "CalibrationState"() -> (w207:T9)
            n188 = global read "AppState.vi" "AppState"() -> (w196:u16)
            n189 = global read "AppState.vi" "AppState"() -> (w191:u16)
            n190 = Not Equal?(x=w183, y=u16 1) -> (x != y?=w185:bool)
            n191 = Not Equal?(x=w183, y=u16 3) -> (x != y?=w186:bool)
            n192 = Unbundle(w179) -> (w181:bool)  [unwired: 4 out]
            n193 = And(x=w185, y=w186) -> (x .and. y?=w177:bool)
            n194 = Not Equal?(x=w201, y=u16 3) -> (x != y?=w202:bool)
            n195 = And(x=w181, y=w177) -> (x .and. y?=w180:bool)
            n196 = Unbundle(w207) -> (w198:bool)  [unwired: 4 out]
            n197 = Not Equal?(x=w191, y=u16 1) -> (x != y?=w189:bool)
            n198 = Not Equal?(x=w191, y=u16 3) -> (x != y?=w188:bool)
            n199 = Not Equal?(x=w196, y=u16 1) -> (x != y?=w193:bool)
            n200 = Not Equal?(x=w196, y=u16 3) -> (x != y?=w194:bool)
            n201 = case shown="False" w180 {
              tunnel: [T8."Disabled and Grayed Out" ("Disabled") T8."Enabled" ("Disabled")] -> w178
              frame False {
              }
              frame True {
              }
            }
            n202 = case shown="False" w202 {
              tunnel: [T8."Disabled and Grayed Out" ("Disabled") T8."Enabled" ("Disabled")] -> w205
              frame False {
              }
              frame True {
              }
            }
            n203 = And(x=w189, y=w188) -> (x .and. y?=w187:bool)
            n204 = And(x=w193, y=w194) -> (x .and. y?=w192:bool)
            n205 = And(x=w198, y=w187) -> (x .and. y?=w199:bool)
            n206 = case shown="False" w192 {
              tunnel: [T8."Disabled and Grayed Out" ("Disabled") T8."Enabled" ("Disabled")] -> w204
              frame False {
              }
              frame True {
              }
            }
            n207 = case shown="False" w199 {
              tunnel: [T8."Disabled and Grayed Out" ("Disabled") T8."Enabled" ("Disabled")] -> w206
              frame False {
              }
              frame True {
              }
            }
            n208 = property on="btnMesureGrain" class="Bool (strict)"("DisabledEnum"=w178) -> ()  [unwired: 2 in, 2 out]
            n209 = property on="btnVidanger" class="Bool (strict)"("DisabledEnum"=w205) -> ()  [unwired: 2 in, 2 out]
            n210 = property on="btnEtal" class="Bool (strict)"("DisabledEnum"=w204) -> ()  [unwired: 2 in, 2 out]
            n211 = property on="btnMesurePore" class="Bool (strict)"("DisabledEnum"=w206) -> ()  [unwired: 2 in, 2 out]
          }
          event "MeasureSetupButtonsVisible": Value Change {
            n212 = event-data() -> ("NewVal"=w217:bool)  [unwired: 1 in, 5 out]
            n213 = local read "MeasureMode"() -> (w219:T1)
            n214 = property on="ReferenceCellMeasure" class="DigNum (strict)"("Visible"=w217) -> ()  [unwired: 2 in, 2 out]
            n215 = property on="SampleNumber" class="Str"("Visible"=w217) -> ()  [unwired: 2 in, 2 out]
            n216 = property on="Temperature" class="DigNum (strict)"("Visible"=w217) -> ()  [unwired: 2 in, 2 out]
            n217 = property on="Comments" class="Str"("Visible"=w217) -> ()  [unwired: 2 in, 2 out]
            n218 = property on="SampleDepth" class="DigNum (strict)"("Visible"=w217) -> ()  [unwired: 2 in, 2 out]
            n219 = property on="DryWeight" class="DigNum (strict)"("Visible"=w217) -> ()  [unwired: 2 in, 2 out]
            n220 = property on="SampleID" class="Str"("Visible"=w217) -> ()  [unwired: 2 in, 2 out]
            n221 = Equal?(x=w219, y=MeasureModeControl."PoreMeasure") -> (x = y?=w220:bool)
            n222 = And(x=w217, y=w220) -> (x .and. y?=w216:bool)
            n223 = property on="BulkVolume" class="DigNum (strict)"("Visible"=w216) -> ()  [unwired: 2 in, 2 out]
            n224 = property on="MeasureTotalAddedVolume" class="DigNum (strict)"("Visible"=w217) -> ()  [unwired: 2 in, 2 out]
            n225 = property on="MeasureDiskSet" class="LstBox (strict)"("Visible"=w217) -> ()  [unwired: 2 in, 2 out]
            n226 = property on="MeasureDiskVolumes" class="LstBox (strict)"("Visible"=w217) -> ()  [unwired: 2 in, 2 out]
            n227 = property on="DoMeasureMeasure" class="Bool (strict)"("Visible"=w217, "DisabledEnum"=T8."Disabled and Grayed Out" ("Disabled")) -> ()  [unwired: 2 in, 2 out]
          }
          event "ReloadDiskVolumes": Value Change {
            # "On re-remplit la liste des volumes des disques"
            # "On re-remplit la liste des volumes des disques"
            n228 = event-data() -> ()  [unwired: 1 in, 6 out]
            n229 = global read "CalibrationVolumes.vi" "AllCalibrationVolumes"() -> (w226:T18)
            n230 = global read "CalibrationVolumes.vi" "AllCalibrationVolumes"() -> (w230:T18)
            n231 = local read "MeasureDiskSet"() -> (w227:i32)
            n232 = global read "CalibrationVolumes.vi" "AllCalibrationVolumes"() -> (w239:T18)
            n233 = local read "DiskSet"() -> (w235:i32)
            n234 = To Long Integer(number=w227) -> (32bit integer=w225:i32)
            n235 = To Long Integer(number=w235) -> (32bit integer=w231:i32)
            n236 = Index Array(array=w226, index=w225) -> (element=w224:T23)
            n237 = Array Size(array=w239) -> (size(s)=w240:i32)
            n238 = Index Array(array=w230, index=w231) -> (element=w232:T23)
            n239 = Unbundle(w224) -> ("DisplayedStrings"=w222:string[])  [unwired: 2 out]
            n240 = for {
              N: w240 -> [_]
              shift-right: [w247] -> w236
              shift-left: string[] [] -> [w248]
              tunnel: w239 -> [w246] mode=indexing
              shift-right: [w242] -> w237
              shift-left: i32[] [] -> [w244]
              i -> [w243]
              n241 = Insert Into Array(array=w244, new element=w243) -> (w242:i32[])  [unwired: 1 in]
              n242 = Unbundle By Name(w246) -> ("SetName"=w245:string)
              n243 = Insert Into Array(array=w248, new element=w245) -> (w247:string[])  [unwired: 1 in]
            }
            n244 = Unbundle(w232) -> ("DisplayedStrings"=w223:string[])  [unwired: 2 out]
            n245 = property on="MeasureDiskVolumes" class="LstBox (strict)"("Item Names"=w222, "DisabledEnum"=T8."Enabled" ("Disabled"), "Val(Sgnl)"=i32[] [] ("Value (Signaling)")) -> ()  [unwired: 2 in, 2 out]
            n246 = property on="AvalaibleVolumesList" class="LstBox (strict)"("Item Names"=w223, "DisabledEnum"=T8."Enabled" ("Disabled"), "Val(Sgnl)"=i32[] [] ("Value (Signaling)")) -> ()  [unwired: 2 in, 2 out]
            n247 = property on="DiskSet" class="LstBox (strict)"("Item Names"=w236, "Item Symbols"=w237) -> ()  [unwired: 2 in, 2 out]
            n248 = property on="MeasureDiskSet" class="LstBox (strict)"("Item Names"=w236, "Item Symbols"=w237) -> ()  [unwired: 2 in, 2 out]
          }
          event "ValvesBoutonVisible": Value Change {
            n249 = event-data() -> ("NewVal"=w249:bool)  [unwired: 1 in, 5 out]
            n250 = property on="V2Btn" class="Bool (strict)"("Visible"=w249) -> ()  [unwired: 2 in, 2 out]
            n251 = property on="V1Btn" class="Bool (strict)"("Visible"=w249) -> ()  [unwired: 2 in, 2 out]
            n252 = property on="Inlet ValveBtn" class="Bool (strict)"("Visible"=w249) -> ()  [unwired: 2 in, 2 out]
            n253 = property on="Sample ValveBtn" class="Bool (strict)"("Visible"=w249) -> ()  [unwired: 2 in, 2 out]
            n254 = property on="Outlet ValveBtn" class="Bool (strict)"("Visible"=w249) -> ()  [unwired: 2 in, 2 out]
          }
          event "MeasureIndicatorsVisible": Value Change {
            n255 = event-data() -> ("NewVal"=w250:bool)  [unwired: 1 in, 5 out]
            n256 = property on="MeasureReportedString" class="Str"("Visible"=w250) -> ()  [unwired: 2 in, 2 out]
            n257 = property on="VolumeMeasureInd" class="DigNum (strict)"("Visible"=w250) -> ()  [unwired: 2 in, 2 out]
            n258 = property on="P1P2RatioMeasure" class="DigNum (strict)"("Visible"=w250) -> ()  [unwired: 2 in, 2 out]
            n259 = property on="measureStabilization" class="Str"("Visible"=w250) -> ()  [unwired: 2 in, 2 out]
          }
          event "ReloadResultTableTexts": Value Change {
            n260 = event-data() -> ()  [unwired: 1 in, 6 out]
            n261 = for {
              N: 15 -> [_]
              i -> [w256]
              n262 = local read "LanguagesList"() -> (w255:i32)
              n263 = global read "LanguagesSettings.vi" "LanguageSettings"() -> (w254:T13)
              n264 = Unbundle By Name(w254) -> ("LocalisationFileContent[out]"=w253:T21)
              n265 = call "FindLocalizedString.vi"("LangIndex"=w255, "LocalizationFileContent"=w253, "WordIndex"=w256) -> ("Found"=w257:bool, "LocalizedString"=w258:string)  [unwired: 7 in]
              n266 = case shown="False" w257 {
                tunnel: w258 -> [_ w378]
                tunnel: ["Not found" w378] -> w252
                frame False {
                }
                frame True {
                }
              }
              n267 = case shown="Default" w256 {
                tunnel: w252 -> [_ w259 w268 w277 w286 w295 w304 w313 w318 w323 w332 w341 w350 w359 w368]
                frame Default {
                }
                frame 1 {
                  n268 = local read "poreMeasuresTable"() -> (w267:string[][])
                  n269 = property on="SampleNumber" class="Str"("Caption.Text"=w259) -> ()  [unwired: 2 in, 2 out]
                  n270 = local read "grainMeasuresTable"() -> (w260:string[][])
                  n271 = Replace Array Subset(array=w267, new element=w259, index (row)=0, index (col)=1) -> (w266:string[][])
                  n272 = local write "poreMeasuresTable"(w266) -> ()
                  n273 = Replace Array Subset(array=w260, new element=w259, index (row)=0, index (col)=1) -> (w261:string[][])
                  n274 = local write "grainMeasuresTable"(w261) -> ()
                }
                frame 2 {
                  n275 = local read "poreMeasuresTable"() -> (w276:string[][])
                  n276 = local read "grainMeasuresTable"() -> (w269:string[][])
                  n277 = property on="SampleID" class="Str"("Caption.Text"=w268) -> ()  [unwired: 2 in, 2 out]
                  n278 = Replace Array Subset(array=w276, new element=w268, index (row)=0, index (col)=2) -> (w275:string[][])
                  n279 = local write "poreMeasuresTable"(w275) -> ()
                  n280 = Replace Array Subset(array=w269, new element=w268, index (row)=0, index (col)=2) -> (w270:string[][])
                  n281 = local write "grainMeasuresTable"(w270) -> ()
                }
                frame 3 {
                  n282 = local read "poreMeasuresTable"() -> (w285:string[][])
                  n283 = local read "grainMeasuresTable"() -> (w278:string[][])
                  n284 = property on="SampleDepth" class="DigNum (strict)"("Caption.Text"=w277) -> ()  [unwired: 2 in, 2 out]
                  n285 = Replace Array Subset(array=w285, new element=w277, index (row)=0, index (col)=3) -> (w284:string[][])
                  n286 = local write "poreMeasuresTable"(w284) -> ()
                  n287 = Replace Array Subset(array=w278, new element=w277, index (row)=0, index (col)=3) -> (w279:string[][])
                  n288 = local write "grainMeasuresTable"(w279) -> ()
                }
                frame 4 {
                  n289 = local read "poreMeasuresTable"() -> (w294:string[][])
                  n290 = local read "grainMeasuresTable"() -> (w287:string[][])
                  n291 = property on="DryWeight" class="DigNum (strict)"("Caption.Text"=w286) -> ()  [unwired: 2 in, 2 out]
                  n292 = Replace Array Subset(array=w294, new element=w286, index (row)=0, index (col)=4) -> (w293:string[][])
                  n293 = local write "poreMeasuresTable"(w293) -> ()
                  n294 = Replace Array Subset(array=w287, new element=w286, index (row)=0, index (col)=4) -> (w288:string[][])
                  n295 = local write "grainMeasuresTable"(w288) -> ()
                }
                frame 5 {
                  n296 = local read "poreMeasuresTable"() -> (w303:string[][])
                  n297 = local read "grainMeasuresTable"() -> (w296:string[][])
                  n298 = property on="BulkVolume" class="DigNum (strict)"("Caption.Text"=w295) -> ()  [unwired: 2 in, 2 out]
                  n299 = Replace Array Subset(array=w303, new element=w295, index (row)=0, index (col)=5) -> (w302:string[][])
                  n300 = local write "poreMeasuresTable"(w302) -> ()
                  n301 = Replace Array Subset(array=w296, new element=w295, index (row)=0, index (col)=5) -> (w297:string[][])
                  n302 = local write "grainMeasuresTable"(w297) -> ()
                }
                frame 6 {
                  n303 = local read "poreMeasuresTable"() -> (w312:string[][])
                  n304 = local read "grainMeasuresTable"() -> (w305:string[][])
                  n305 = Replace Array Subset(array=w312, new element=w304, index (row)=0, index (col)=6) -> (w311:string[][])
                  n306 = local write "poreMeasuresTable"(w311) -> ()
                  n307 = Replace Array Subset(array=w305, new element=w304, index (row)=0, index (col)=6) -> (w306:string[][])
                  n308 = local write "grainMeasuresTable"(w306) -> ()
                }
                frame 7 {
                  n309 = local read "poreMeasuresTable"() -> (w317:string[][])
                  n310 = Replace Array Subset(array=w317, new element=w313, index (row)=0, index (col)=7) -> (w316:string[][])
                  n311 = local write "poreMeasuresTable"(w316) -> ()
                }
                frame 8 {
                  n312 = local read "poreMeasuresTable"() -> (w322:string[][])
                  n313 = Replace Array Subset(array=w322, new element=w318, index (row)=0, index (col)=8) -> (w321:string[][])
                  n314 = local write "poreMeasuresTable"(w321) -> ()
                }
                frame 9 {
                  n315 = local read "poreMeasuresTable"() -> (w331:string[][])
                  n316 = local read "grainMeasuresTable"() -> (w324:string[][])
                  n317 = Replace Array Subset(array=w331, new element=w323, index (row)=0, index (col)=9) -> (w330:string[][])
                  n318 = local write "poreMeasuresTable"(w330) -> ()
                  n319 = Replace Array Subset(array=w324, new element=w323, index (row)=0, index (col)=7) -> (w325:string[][])
                  n320 = local write "grainMeasuresTable"(w325) -> ()
                }
                frame 10 {
                  n321 = local read "poreMeasuresTable"() -> (w340:string[][])
                  n322 = local read "grainMeasuresTable"() -> (w333:string[][])
                  n323 = Replace Array Subset(array=w340, new element=w332, index (row)=0, index (col)=10) -> (w339:string[][])
                  n324 = local write "poreMeasuresTable"(w339) -> ()
                  n325 = Replace Array Subset(array=w333, new element=w332, index (row)=0, index (col)=8) -> (w334:string[][])
                  n326 = local write "grainMeasuresTable"(w334) -> ()
                }
                frame 11 {
                  n327 = local read "poreMeasuresTable"() -> (w349:string[][])
                  n328 = local read "grainMeasuresTable"() -> (w342:string[][])
                  n329 = Replace Array Subset(array=w349, new element=w341, index (row)=0, index (col)=11) -> (w348:string[][])
                  n330 = local write "poreMeasuresTable"(w348) -> ()
                  n331 = Replace Array Subset(array=w342, new element=w341, index (row)=0, index (col)=9) -> (w343:string[][])
                  n332 = local write "grainMeasuresTable"(w343) -> ()
                }
                frame 12 {
                  n333 = local read "poreMeasuresTable"() -> (w358:string[][])
                  n334 = local read "grainMeasuresTable"() -> (w351:string[][])
                  n335 = Replace Array Subset(array=w358, new element=w350, index (row)=0, index (col)=12) -> (w357:string[][])
                  n336 = local write "poreMeasuresTable"(w357) -> ()
                  n337 = Replace Array Subset(array=w351, new element=w350, index (row)=0, index (col)=10) -> (w352:string[][])
                  n338 = local write "grainMeasuresTable"(w352) -> ()
                }
                frame 13 {
                  n339 = local read "poreMeasuresTable"() -> (w367:string[][])
                  n340 = property on="Temperature" class="DigNum (strict)"("Caption.Text"=w359) -> ()  [unwired: 2 in, 2 out]
                  n341 = local read "grainMeasuresTable"() -> (w360:string[][])
                  n342 = Replace Array Subset(array=w367, new element=w359, index (row)=0, index (col)=13) -> (w366:string[][])
                  n343 = local write "poreMeasuresTable"(w366) -> ()
                  n344 = Replace Array Subset(array=w360, new element=w359, index (row)=0, index (col)=11) -> (w361:string[][])
                  n345 = local write "grainMeasuresTable"(w361) -> ()
                }
                frame 14 {
                  n346 = local read "poreMeasuresTable"() -> (w376:string[][])
                  n347 = property on="Comments" class="Str"("Caption.Text"=w368) -> ()  [unwired: 2 in, 2 out]
                  n348 = local read "grainMeasuresTable"() -> (w369:string[][])
                  n349 = Replace Array Subset(array=w376, new element=w368, index (row)=0, index (col)=14) -> (w375:string[][])
                  n350 = local write "poreMeasuresTable"(w375) -> ()
                  n351 = Replace Array Subset(array=w369, new element=w368, index (row)=0, index (col)=12) -> (w370:string[][])
                  n352 = local write "grainMeasuresTable"(w370) -> ()
                }
              }
            }
          }
        }
        n353 = local read "btnExit"() -> (w123:bool)
      }
      n354 = while {
        shift-right: [w380] -> _
        shift-left: w116 -> [w382]
        stop <- w383 stop-if-true
        n355 = event shown="[22] \"LanguagesList\": Value Change" {
          selector: _ -> [_ _ _ _ _ _ _ _ _ _ _ _ _ _ _ _ _ _ _ _ _ _ _ _ _ _ _ _ _ _ _ _ _ _ _ _ _ _ _ _ _ _ _ _ _ _ _ _ _ _ _ _ _ _ _ _ _ _ _ _ _ _ _ _ _ _ _ _ _ _ _ _ _ _]
          dyn-events: _ -> [_ _ _ _ _ _ _ _ _ _ _ _ _ _ _ _ _ _ _ _ _ _ _ _ _ _ _ _ _ _ _ _ _ _ _ _ _ _ _ _ _ _ _ _ _ _ _ _ _ _ _ _ _ _ _ _ _ _ _ _ _ _ _ _ _ _ _ _ _ _ _ _ _ _]
          timeout: 100 -> [_ _ _ _ _ _ _ _ _ _ _ _ _ _ _ _ _ _ _ _ _ _ _ _ _ _ _ _ _ _ _ _ _ _ _ _ _ _ _ _ _ _ _ _ _ _ _ _ _ _ _ _ _ _ _ _ _ _ _ _ _ _ _ _ _ _ _ _ _ _ _ _ _ _]
          tunnel: w382 -> [_ _ w407 w481 w501 _ _ _ _ _ _ _ _ _ _ _ _ w542 _ _ _ _ _ w899 w903 _ w930 _ _ w947 w960 w972 w983 w994 _ _ _ _ _ _ _ w1069 _ _ w1121 _ _ _ w1173 _ _ _ _ _ _ _ _ _ _ _ _ _ _ _ _ _ _ _ _ w1405 _ w1417 w1439 w1475]
          tunnel: [_ _ w409 w480 w500 _ _ _ _ _ _ _ _ _ _ _ _ w543 _ _ _ _ _ w899 w903 _ w925 _ _ w949 w959 w971 w981 w992 _ _ _ _ _ _ _ w1068 _ _ w1120 _ _ _ w1172 _ _ _ _ _ _ _ _ _ _ _ _ _ _ _ _ _ _ _ _ w1404 _ w1416 w1438 w1474] -> w379
          event "btnMesurePore": Value Change {
            # "Si la calibration est faîte, que l'on est\nen mode idle: on lance la mesure"
            n356 = event-data() -> ("NewVal"=w390:bool)  [unwired: 1 in, 5 out]
            n357 = global read "CalibrationState.vi" "CalibrationState"() -> (w389:T9)
            n358 = Unbundle(w389) -> (w388:bool)  [unwired: 4 out]
            n359 = And(x=w388, y=w390) -> (x .and. y?=w387:bool)
            n360 = case shown="True" w387 {
              frame False {
              }
              frame True {
                n361 = stacked-sequence {
                  frame #0 {
                    # "On désactive le mode automatique"
                    n362 = property on="manualModeBtn" class="Bool (strict)"("Val(Sgnl)"=FALSE ("Value (Signaling)")) -> ()  [unwired: 2 in, 2 out]
                  }
                  frame #1 {
                    # "On passe en mode mesure: et on indique que c'est une mesure de pores"
                    n363 = global write "AppState.vi" "AppState"(u16 2 ("AppState")) -> ()
                    n364 = local write "MeasureMode"(MeasureModeControl."PoreMeasure" ("MeasureMode")) -> ()
                  }
                  frame #2 {
                    w394 = TRUE ("Value (Signaling)")
                    w395 = FALSE ("Value (Signaling)")
                    # "On efface/affiche les contrôles qu'il faut. On change l'état de l'app"
                    n365 = property on="MeasureSetupButtonsVisible" class="Bool (strict)"("Val(Sgnl)"=w394) -> ()  [unwired: 2 in, 2 out]
                    n366 = property on="ChangeMenuState" class="Bool (strict)"("Val(Sgnl)"=w394) -> ()  [unwired: 2 in, 2 out]
                    n367 = property on="ReloadDiskVolumes" class="Bool (strict)"("Val(Sgnl)"=w394) -> ()  [unwired: 2 in, 2 out]
                    n368 = property on="CalibrationResultsVisible" class="Bool (strict)"("Val(Sgnl)"=w395) -> ()  [unwired: 2 in, 2 out]
                    n369 = property on="CalibrationButtonsVisible" class="Bool (strict)"("Val(Sgnl)"=w395) -> ()  [unwired: 2 in, 2 out]
                    n370 = property on="MeasureIndicatorsVisible" class="Bool (strict)"("Val(Sgnl)"=w395) -> ()  [unwired: 2 in, 2 out]
                    n371 = property on="PurgeState" class="Str"("Visible"=w395) -> ()  [unwired: 2 in, 2 out]
                    n372 = property on="ExportMeasuresButtonsVisible" class="Bool (strict)"("Val(Sgnl)"=w395) -> ()  [unwired: 2 in, 2 out]
                  }
                  frame #3 {
                    # "On change l'onglet des résultats de mesure affiché"
                    n373 = property on="MeasuresTabs" class="TabCtl (strict)"("Value"=enum32{"Grain measures", "Pore measures"}."Pore measures" ("MeasuresTabs")) -> ()  [unwired: 2 in, 2 out]
                  }
                }
              }
            }
          }
          event "btnMesureGrain": Value Change {
            # "Si la calibration est faîte, que l'on est\nen mode idle: on lance la mesure"
            n374 = event-data() -> ("NewVal"=w397:bool)  [unwired: 1 in, 5 out]
            n375 = global read "CalibrationState.vi" "CalibrationState"() -> (w400:T9)
            n376 = Unbundle(w400) -> (w399:bool)  [unwired: 4 out]
            n377 = And(x=w399, y=w397) -> (x .and. y?=w398:bool)
            n378 = case shown="True" w398 {
              frame False {
              }
              frame True {
                n379 = stacked-sequence {
                  frame #0 {
                    # "On désactive le mode automatique"
                    n380 = property on="manualModeBtn" class="Bool (strict)"("Val(Sgnl)"=FALSE ("Value (Signaling)")) -> ()  [unwired: 2 in, 2 out]
                  }
                  frame #1 {
                    # "On passe en mode mesure: et on indique que c'est une mesure de pores"
                    n381 = global write "AppState.vi" "AppState"(u16 2 ("AppState")) -> ()
                    n382 = local write "MeasureMode"(MeasureModeControl."GrainMeasure" ("MeasureMode")) -> ()
                  }
                  frame #2 {
                    w404 = TRUE ("Value (Signaling)")
                    w405 = FALSE ("Value (Signaling)")
                    # "On efface/affiche les contrôles qu'il faut. On change l'état de l'app"
                    n383 = property on="MeasureSetupButtonsVisible" class="Bool (strict)"("Val(Sgnl)"=w404) -> ()  [unwired: 2 in, 2 out]
                    n384 = property on="ChangeMenuState" class="Bool (strict)"("Val(Sgnl)"=w404) -> ()  [unwired: 2 in, 2 out]
                    n385 = property on="ReloadDiskVolumes" class="Bool (strict)"("Val(Sgnl)"=w404) -> ()  [unwired: 2 in, 2 out]
                    n386 = property on="CalibrationResultsVisible" class="Bool (strict)"("Val(Sgnl)"=w405) -> ()  [unwired: 2 in, 2 out]
                    n387 = property on="CalibrationButtonsVisible" class="Bool (strict)"("Val(Sgnl)"=w405) -> ()  [unwired: 2 in, 2 out]
                    n388 = property on="MeasureIndicatorsVisible" class="Bool (strict)"("Val(Sgnl)"=w405) -> ()  [unwired: 2 in, 2 out]
                    n389 = property on="PurgeState" class="Str"("Visible"=w405) -> ()  [unwired: 2 in, 2 out]
                    n390 = property on="ExportMeasuresButtonsVisible" class="Bool (strict)"("Val(Sgnl)"=w405) -> ()  [unwired: 2 in, 2 out]
                  }
                  frame #3 {
                    # "On change l'onglet de résultats de mesures affiché"
                    n391 = property on="MeasuresTabs" class="TabCtl (strict)"("Value"=enum32{"Grain measures", "Pore measures"}."Grain measures" ("MeasuresTabs")) -> ()  [unwired: 2 in, 2 out]
                  }
                }
              }
            }
          }
          event "DoMeasureMeasure": Value Change {
            # "Si on est bien dans l'état de mesure"
            n392 = event-data() -> ("NewVal"=w413:bool)  [unwired: 1 in, 5 out]
            n393 = global read "AppState.vi" "AppState"() -> (w411:u16)
            n394 = Equal?(x=w411, y=u16 2) -> (x = y?=w412:bool)
            n395 = And(x=w412, y=w413) -> (x .and. y?=w408:bool)
            n396 = case shown="True" w408 {
              tunnel: w407 -> [w414 w416]
              tunnel: [w414 w415] -> w409
              frame False {
              }
              frame True {
                n397 = stacked-sequence {
                  tunnel: w416 -> [_ w435 _ _]
                  tunnel: [_ w430 _ _] -> w415
                  frame #0 {
                    n398 = property on="manualModeBtn" class="Bool (strict)"("DisabledEnum"=T8."Disabled and Grayed Out" ("Disabled"), "Val(Sgnl)"=FALSE ("Value (Signaling)")) -> ()  [unwired: 2 in, 2 out]
                  }
                  frame #1 {
                    # "Effectue la mesure et reporte la valeur"
                    n399 = local read "MeasureTotalAddedVolume"() -> (w428:dbl)
                    n400 = local read "ReferenceCellMeasure"() -> (w447:u16)
                    n401 = global read "PressureAndTimeSamples.vi" "PressureAndTimeSamples"() -> (w449:T3)
                    n402 = global read "FittedCurvePolynom.vi" "FittedCurvePolynom"() -> (w448:dbl[])
                    n403 = To Long Integer(number=w447) -> (32bit integer=w450:i32)
                    n404 = call "Measure.vi"("Graph in"=w449, "error in"=w435, "Reference Cell"=w450) -> ("error out"=w430:errorcluster, "Values"=w425:cluster{dbl[], dbl[]}, "P1/P2"=w432:dbl, "StabilityAchieved"=w431:bool)  [unwired: 5 in]
                    n405 = local write "StabilityAchieved"(w431) -> ()
                    n406 = global write "PressureAndTimeSamples.vi" "PressureAndTimeSamples"(w425) -> ()
                    n407 = Build Array(w432) -> (w427:dbl[])
                    n408 = local write "P1P2RatioMeasure"(w432) -> ()
                    n409 = call "Horner.vi"("Meilleure poly"=w448, "X"=w427) -> ("Y"=w426:dbl[])  [unwired: 9 in]
                    n410 = call "ElementWiseMinus.vi"("a"=w428, "Array [in]"=w426) -> ("Array[out]"=w429:dbl[])  [unwired: 9 in]
                    n411 = local read "SampleNumber"() -> (w444:string)
                    n412 = local read "SampleDepth"() -> (w442:dbl)
                    n413 = local read "Temperature"() -> (w441:dbl)
                    n414 = local read "BulkVolume"() -> (w437:dbl)
                    n415 = local read "Comments"() -> (w440:string)
                    n416 = local read "DryWeight"() -> (w436:dbl)
                    n417 = local read "SampleID"() -> (w443:string)
                    n418 = Bundle("SampleNumber"=w444, "SampleID"=w443, "SampleDepth"=w442, "DryWeight"=w436, "BulkVolume"=w437, "Temperature"=w441, "Comments"=w440) -> (w445:T24)  [unwired: 1 in]
                    n419 = local read "MeasureMode"() -> (w419:T1)
                    n420 = Index Array(array=w429, index=0) -> (element=w433:dbl)
                    n421 = local read "MeasureMode"() -> (w424:T1)
                    n422 = local write "VolumeMeasureInd"(w433) -> ()
                    n423 = call "ComputeSampleData.vi"("MeasureMode"=w419, "MeasuredVolume"=w433, "UserFilledData"=w445) -> ("MeasureData"=w446:T25)  [unwired: 8 in]
                    n424 = local read "MeasureMode"() -> (w422:T1)
                    n425 = call "DataToStringArray.vi"("MeasureMode"=w424, "MeasureData"=w446) -> ("Array"=w438:string[])  [unwired: 9 in]
                    n426 = Equal?(x=w422, y=MeasureModeControl."PoreMeasure") -> (x = y?=w420:bool)
                    n427 = case shown="True" w420 {
                      tunnel: [w453 w454] -> w439
                      frame False {
                        n428 = property on="grainMeasuresTable" class="Tbl (strict)"() -> ("Value"=w453:string[][])  [unwired: 2 in, 2 out]
                      }
                      frame True {
                        n429 = property on="poreMeasuresTable" class="Tbl (strict)"() -> ("Value"=w454:string[][])  [unwired: 2 in, 2 out]
                      }
                    }
                    n430 = Insert Into Array(array=w439, new element=w438) -> (w423:string[][])  [unwired: 2 in]
                    n431 = case shown="True" w420 {
                      tunnel: w423 -> [w451 w452]
                      frame False {
                        n432 = property on="grainMeasuresTable" class="Tbl (strict)"("Value"=w451) -> ()  [unwired: 2 in, 2 out]
                      }
                      frame True {
                        n433 = property on="poreMeasuresTable" class="Tbl (strict)"("Value"=w452) -> ()  [unwired: 2 in, 2 out]
                      }
                    }
                  }
                  frame #2 {
                    # "Affiche/cache les boutons qu'il faut"
                    n434 = property on="MeasureIndicatorsVisible" class="Bool (strict)"("Val(Sgnl)"=TRUE) -> ()  [unwired: 2 in, 2 out]
                    n435 = global write "AppState.vi" "AppState"(u16 0 ("AppState")) -> ()
                    n436 = property on="manualModeBtn" class="Bool (strict)"("DisabledEnum"=T8."Enabled" ("Disabled")) -> ()  [unwired: 2 in, 2 out]
                    n437 = global read "LanguagesSettings.vi" "LanguageSettings"() -> (w465:T13)
                    n438 = Unbundle By Name(w465) -> ("LocalisationFileContent[out]"=w466:T21)
                    n439 = local read "StabilityAchieved"() -> (w461:bool)
                    n440 = local read "MeasureMode"() -> (w456:T1)
                    n441 = local read "LanguagesList"() -> (w462:i32)
                    n442 = case shown="False" w461 {
                      tunnel: [u32 131 ("WordIndex") u32 130 ("WordIndex")] -> w460
                      frame False {
                      }
                      frame True {
                      }
                    }
                    n443 = call "FindLocalizedString.vi"("LangIndex"=w462, "LocalizationFileContent"=w466, "WordIndex"=w460) -> ("Found"=w463:bool, "LocalizedString"=w464:string)  [unwired: 7 in]
                    n444 = Equal?(x=w456, y=MeasureModeControl."GrainMeasure") -> (x = y?=w457:bool)
                    n445 = case shown="False" w463 {
                      tunnel: w464 -> [_ w477]
                      tunnel: ["Not found" w477] -> w459
                      frame False {
                      }
                      frame True {
                      }
                    }
                    n446 = case shown="False" w457 {
                      tunnel: [enum32{"Grain measures", "Pore measures"}."Pore measures" ("MeasuresTabs") enum32{"Grain measures", "Pore measures"}."Grain measures" ("MeasuresTabs")] -> w458
                      frame False {
                      }
                      frame True {
                      }
                    }
                    n447 = local write "measureStabilization"(w459) -> ()
                    n448 = property on="MeasuresTabs" class="TabCtl (strict)"("Value"=w458) -> ()  [unwired: 2 in, 2 out]
                    n449 = property on="DoMeasureMeasure" class="Bool (strict)"("Value"=FALSE ("DoMeasureMeasure")) -> ()  [unwired: 2 in, 2 out]
                    n450 = property on="MeasureSetupButtonsVisible" class="Bool (strict)"("Val(Sgnl)"=FALSE ("Value (Signaling)")) -> ()  [unwired: 2 in, 2 out]
                  }
                  frame #3 {
                    n451 = property on="ChangeMenuState" class="Bool (strict)"("Val(Sgnl)"=TRUE ("Value (Signaling)")) -> ()  [unwired: 2 in, 2 out]
                  }
                }
              }
            }
          }
          event "SaveData": Value Change {
            n452 = event-data() -> ("NewVal"=w479:bool)  [unwired: 1 in, 5 out]
            n453 = case shown="True" w479 {
              tunnel: w481 -> [w482 w490]
              tunnel: [w482 w489] -> w480
              frame False {
              }
              frame True {
                n454 = call "File Dialog4"("default name"="data.csv", "error in"=w490, "pattern (all files)"="*.csv", "pattern label"="Data file") -> ("selected path"=w483:path, "cancelled"=w484:bool, "error out"=w489:errorcluster)  [unwired: 8 in, 1 out]
                n455 = Not(x=w484) -> (.not. x?=w485:bool)
                n456 = case shown="True" w485 {
                  tunnel: w483 -> [_ w496]
                  frame False {
                  }
                  frame True {
                    n457 = local read "MeasureMode"() -> (w492:T1)
                    n458 = Equal?(x=w492, y=MeasureModeControl."PoreMeasure" ("MeasureMode")) -> (x = y?=w493:bool)
                    n459 = case shown="True" w493 {
                      tunnel: [w497 w498] -> w494
                      frame False {
                        n460 = property on="grainMeasuresTable" class="Tbl (strict)"() -> ("Value"=w497:string[][])  [unwired: 2 in, 2 out]
                      }
                      frame True {
                        n461 = property on="poreMeasuresTable" class="Tbl (strict)"() -> ("Value"=w498:string[][])  [unwired: 2 in, 2 out]
                      }
                    }
                    n462 = call-poly <vilib>:"Write To Spreadsheet File.vi"("delimiter (\\t)"=";" ("delimiter (\\t)"), "2D data"=w494, "file path (dialog if empty)"=w496) -> ()  [unwired: 5 in, 1 out]
                  }
                }
              }
            }
          }
          event "LoadData": Value Change {
            n463 = event-data() -> ("NewVal"=w499:bool)  [unwired: 1 in, 5 out]
            n464 = case shown="True" w499 {
              tunnel: w501 -> [w502 w504]
              tunnel: [w502 w503] -> w500
              frame False {
              }
              frame True {
                n465 = call "File Dialog"("default name"="data.csv", "error in"=w504, "pattern (all files)"="*.csv", "pattern label"="Data file") -> ("selected path"=w510:path, "cancelled"=w509:bool, "error out"=w503:errorcluster)  [unwired: 8 in, 1 out]
                n466 = Not(x=w509) -> (.not. x?=w508:bool)
                n467 = case shown="True" w508 {
                  tunnel: w510 -> [_ w516]
                  frame False {
                  }
                  frame True {
                    n468 = call-poly <vilib>:"Read From Spreadsheet File.vi"("delimiter (\\t)"=";" ("delimiter (\\t)"), "file path (dialog if empty)"=w516) -> ("all rows"=w511:string[][])  [unwired: 5 in, 4 out]
                    n469 = local read "MeasureMode"() -> (w513:T1)
                    n470 = Equal?(x=w513, y=MeasureModeControl."PoreMeasure" ("MeasureMode")) -> (x = y?=w514:bool)
                    n471 = case shown="True" w514 {
                      tunnel: w511 -> [w517 w518]
                      frame False {
                        n472 = property on="grainMeasuresTable" class="Tbl (strict)"("Value"=w517) -> ()  [unwired: 2 in, 2 out]
                      }
                      frame True {
                        n473 = property on="poreMeasuresTable" class="Tbl (strict)"("Value"=w518) -> ()  [unwired: 2 in, 2 out]
                      }
                    }
                  }
                }
              }
            }
          }
          event "ExportData": Value Change {
            n474 = event-data() -> ("NewVal"=w519:bool)  [unwired: 1 in, 5 out]
            n475 = case shown="True" w519 {
              selector: w519 -> [_ w524]
              frame False {
              }
              frame True {
                w523 = FALSE ("Value (Signaling)")
                n476 = property on="ExportMeasuresButtonsVisible" class="Bool (strict)"("Val(Sgnl)"=w524) -> ()  [unwired: 2 in, 2 out]
                n477 = property on="CalibrationButtonsVisible" class="Bool (strict)"("Val(Sgnl)"=w523) -> ()  [unwired: 2 in, 2 out]
                n478 = property on="CalibrationResultsVisible" class="Bool (strict)"("Val(Sgnl)"=w523) -> ()  [unwired: 2 in, 2 out]
                n479 = property on="MeasureIndicatorsVisible" class="Bool (strict)"("Val(Sgnl)"=w523) -> ()  [unwired: 2 in, 2 out]
                n480 = property on="MeasureSetupButtonsVisible" class="Bool (strict)"("Val(Sgnl)"=w523) -> ()  [unwired: 2 in, 2 out]
                n481 = property on="PurgeState" class="Str"("Visible"=FALSE) -> ()  [unwired: 2 in, 2 out]
                n482 = property on="ChangeMenuState" class="Bool (strict)"("Val(Sgnl)"=TRUE ("Value (Signaling)")) -> ()  [unwired: 2 in, 2 out]
                n483 = global write "AppState.vi" "AppState"(u16 5 ("AppState")) -> ()
              }
            }
          }
          event "SampleNumber": Value Change {
            n484 = event-data() -> ()  [unwired: 1 in, 6 out]
            n485 = property on="UserFilledDataChanged" class="Bool (strict)"("Val(Sgnl)"=TRUE ("Value (Signaling)")) -> ()  [unwired: 2 in, 2 out]
          }
          event "SleeveConfiguration": Value Change {
            n486 = event-data() -> ()  [unwired: 1 in, 6 out]
            n487 = local read "SleeveConfiguration"() -> (w526:T6)
            n488 = global write "PreconfiguredSleeveData.vi" "PreconfiguredSleeveData"(w526) -> ()
          }
          event "btnExit": Value Change {
            w527 = TRUE ("Visible")
            w528 = T8."Enabled" ("Disabled")
            n489 = event-data() -> ()  [unwired: 1 in, 6 out]
            n490 = property on="PurgeState" class="Str"("Visible"=w527) -> ()  [unwired: 2 in, 2 out]
            n491 = property on="CalibrationButtonsVisible" class="Bool (strict)"("Val(Sgnl)"=w527) -> ()  [unwired: 2 in, 2 out]
            n492 = property on="CalibrationResultsVisible" class="Bool (strict)"("Val(Sgnl)"=w527) -> ()  [unwired: 2 in, 2 out]
            n493 = property on="MeasureIndicatorsVisible" class="Bool (strict)"("Val(Sgnl)"=w527) -> ()  [unwired: 2 in, 2 out]
            n494 = property on="MeasureSetupButtonsVisible" class="Bool (strict)"("Val(Sgnl)"=w527) -> ()  [unwired: 2 in, 2 out]
            n495 = property on="ExportMeasuresButtonsVisible" class="Bool (strict)"("Val(Sgnl)"=w527) -> ()  [unwired: 2 in, 2 out]
            n496 = property on="btnMesurePore" class="Bool (strict)"("DisabledEnum"=w528) -> ()  [unwired: 2 in, 2 out]
            n497 = property on="btnVidanger" class="Bool (strict)"("DisabledEnum"=w528) -> ()  [unwired: 2 in, 2 out]
            n498 = property on="btnEtal" class="Bool (strict)"("DisabledEnum"=w528) -> ()  [unwired: 2 in, 2 out]
          }
          event "MachineName": Value Change {
            n499 = event-data() -> ("NewVal"=w529:string)  [unwired: 1 in, 5 out]
            n500 = global read "MachineInfos.vi" "MachineInfos"() -> (w532:T14)
            n501 = Unbundle By Name(w532) -> ("SerialNumber"=w530:string)
            n502 = Bundle("SerialNumber"=w530, "NewVal"=w529) -> (w531:cluster{"SerialNumber":string, "NewVal":string})  [unwired: 1 in]
            n503 = global write "MachineInfos.vi" "MachineInfos"(w531) -> ()
          }
          event "SampleID": Value Change {
            n504 = event-data() -> ()  [unwired: 1 in, 6 out]
            n505 = property on="UserFilledDataChanged" class="Bool (strict)"("Val(Sgnl)"=TRUE ("Value (Signaling)")) -> ()  [unwired: 2 in, 2 out]
          }
          event "SampleDepth": Value Change {
            n506 = event-data() -> ()  [unwired: 1 in, 6 out]
            n507 = property on="UserFilledDataChanged" class="Bool (strict)"("Val(Sgnl)"=TRUE ("Value (Signaling)")) -> ()  [unwired: 2 in, 2 out]
          }
          event "DryWeight": Value Change {
            n508 = event-data() -> ()  [unwired: 1 in, 6 out]
            n509 = property on="UserFilledDataChanged" class="Bool (strict)"("Val(Sgnl)"=TRUE ("Value (Signaling)")) -> ()  [unwired: 2 in, 2 out]
          }
          event "BulkVolume": Value Change {
            n510 = event-data() -> ()  [unwired: 1 in, 6 out]
            n511 = property on="UserFilledDataChanged" class="Bool (strict)"("Val(Sgnl)"=TRUE ("Value (Signaling)")) -> ()  [unwired: 2 in, 2 out]
          }
          event "Temperature": Value Change {
            n512 = event-data() -> ()  [unwired: 1 in, 6 out]
            n513 = property on="UserFilledDataChanged" class="Bool (strict)"("Val(Sgnl)"=TRUE ("Value (Signaling)")) -> ()  [unwired: 2 in, 2 out]
          }
          event "Comments": Value Change {
            n514 = event-data() -> ()  [unwired: 1 in, 6 out]
            n515 = property on="UserFilledDataChanged" class="Bool (strict)"("Val(Sgnl)"=TRUE ("Value (Signaling)")) -> ()  [unwired: 2 in, 2 out]
          }
          event "UserFilledDataChanged": Value Change {
            n516 = event-data() -> ("NewVal"=w539:bool)  [unwired: 1 in, 5 out]
            n517 = case shown="True" w539 {
              frame False {
              }
              frame True {
                n518 = local write "UserFilledDataChanged"(FALSE ("UserFilledDataChanged")) -> ()
                n519 = property on="DoMeasureMeasure" class="Bool (strict)"("DisabledEnum"=T8."Enabled" ("Disabled")) -> ()  [unwired: 2 in, 2 out]
              }
            }
          }
          event "SaveConfigChanges": Value Change {
            n520 = event-data() -> ("NewVal"=w544:bool)  [unwired: 1 in, 5 out]
            n521 = case shown="True" w544 {
              tunnel: w542 -> [w545 w548]
              tunnel: [w545 w547] -> w543
              frame False {
              }
              frame True {
                n522 = flat-sequence {
                  tunnel: w548 -> [w550]
                  tunnel: [w549] -> w546
                  tunnel: [w552] -> w547
                  tunnel: w546 -> [w552]
                  frame #0 {
                    n523 = call "WriteConfiguration.vi"("error in"=w550) -> ("error out"=w549:errorcluster)  [unwired: 10 in]
                  }
                  frame #1 {
                    n524 = local write "SaveConfigChanges"(FALSE ("SaveConfigChanges")) -> ()
                  }
                }
              }
            }
          }
          event "MinimalWaitTime": Value Change {
            n525 = event-data() -> ("NewVal"=w554:u32)  [unwired: 1 in, 5 out]
            n526 = global read "StabilizationSettings.vi" "StabilizationSettings"() -> (w556:T19)
            n527 = Unbundle(w556) -> ("VarianceTrigger"=w555:dbl, "MaxWaitTime"=w553:u32)  [unwired: 1 out]
            n528 = Bundle("NewVal"=w554, "VarianceTrigger"=w555, "MaxWaitTime"=w553) -> (w557:T26)  [unwired: 1 in]
            n529 = global write "StabilizationSettings.vi" "StabilizationSettings"(w557) -> ()
          }
          event "VarianceTrigger": Value Change {
            n530 = event-data() -> ("NewVal"=w559:dbl)  [unwired: 1 in, 5 out]
            n531 = global read "StabilizationSettings.vi" "StabilizationSettings"() -> (w562:T19)
            n532 = Unbundle(w562) -> ("MinimalWaitTime"=w560:u32, "MaxWaitTime"=w558:u32)  [unwired: 1 out]
            n533 = Bundle("MinimalWaitTime"=w560, "NewVal"=w559, "MaxWaitTime"=w558) -> (w561:T27)  [unwired: 1 in]
            n534 = global write "StabilizationSettings.vi" "StabilizationSettings"(w561) -> ()
          }
          event "MaximalWaitTime": Value Change {
            n535 = event-data() -> ("NewVal"=w563:u32)  [unwired: 1 in, 5 out]
            n536 = global read "StabilizationSettings.vi" "StabilizationSettings"() -> (w567:T19)
            n537 = Unbundle(w567) -> ("MinimalWaitTime"=w565:u32, "VarianceTrigger"=w564:dbl)  [unwired: 1 out]
            n538 = Bundle("MinimalWaitTime"=w565, "VarianceTrigger"=w564, "NewVal"=w563) -> (w566:T28)  [unwired: 1 in]
            n539 = global write "StabilizationSettings.vi" "StabilizationSettings"(w566) -> ()
          }
          event "PressureCaptorConfig", "ValvesConfig", "Valve mapping": Value Change {
            n540 = event-data() -> ()  [unwired: 1 in, 6 out]
            n541 = local read "ValvesConfig"() -> (w594:T7)
            n542 = local read "PressureCaptorConfig"() -> (w573:T4)
            n543 = Unbundle By Name(w594) -> ("Baudrate"=w592:u32, "Port"=w587:string, "Databits"=w591:u16, "Parity"=w590:u16, "Stopbits"=w589:u16, "Flow Control"=w588:u16, "Slave Address"=w585:u16, "Mode"=w584:u16, "Timeout (ms)"=w586:u16)
            n544 = Unbundle By Name(w573) -> ("Baudrate"=w582:u32, "Port"=w577:string, "Databits"=w581:u16, "Parity"=w580:u16, "Stopbits"=w579:u16, "Flow Control"=w578:u16, "Slave Address"=w575:u16, "Register Address"=w571:u16, "Timeout (ms)"=w576:u16, "MaxCaptorPressure"=w568:dbl)
            n545 = local read "Valve mapping"() -> (w569:T5)
            n546 = Bundle("Mode"=w584, "Slave Address"=w585) -> (w583:cluster{"Mode":u16, "Slave Address":u16})  [unwired: 1 in]
            n547 = Bundle("Baudrate"=w592, "Databits"=w591, "Parity"=w590, "Stopbits"=w589, "Flow Control"=w588, "Port"=w587, w583, "Timeout (ms)"=w586, "Valve mapping"=w569) -> (w593:T29)  [unwired: 1 in]
            n548 = Bundle(u16 0, "Slave Address"=w575) -> (w574:cluster{u16, "Slave Address":u16})  [unwired: 1 in]
            n549 = global write "ValveParameters.vi" "ValveParameters"(w593) -> ()
            n550 = Bundle("Baudrate"=w582, "Databits"=w581, "Parity"=w580, "Stopbits"=w579, "Flow Control"=w578, "Port"=w577, "Register Address"=w571, w574, "Timeout (ms)"=w576, "MaxCaptorPressure"=w568) -> (w572:T30)  [unwired: 1 in]
            n551 = global write "CaptParameters.vi" "CaptParameters"(w572) -> ()
          }
          event "LanguagesList": Value Change {
            n552 = event-data() -> ()  [unwired: 1 in, 6 out]
            n553 = global read "LanguagesSettings.vi" "LanguageSettings"() -> (w599:T13)
            n554 = for {
              N: 200 -> [_]
              i -> [w605]
              n555 = local read "LanguagesList"() -> (w604:i32)
              n556 = global read "LanguagesSettings.vi" "LanguageSettings"() -> (w603:T13)
              n557 = Unbundle By Name(w603) -> ("LocalisationFileContent[out]"=w602:T21)
              n558 = call "FindLocalizedString.vi"("LangIndex"=w604, "LocalizationFileContent"=w602, "WordIndex"=w605) -> ("Found"=w606:bool, "LocalizedString"=w608:string)  [unwired: 7 in]
              n559 = case shown="False" w606 {
                tunnel: w608 -> [_ w897]
                tunnel: ["Not found" w897] -> w607
                frame False {
                }
                frame True {
                }
              }
              n560 = case shown="46" w605 {
                tunnel: w607 -> [_ w609 w618 w627 w636 w645 w654 w663 w668 w673 w682 w691 w700 w709 w718 _ _ _ _ _ _ _ _ _ w727 w733 w738 _ w742 w743 w744 w745 w746 w748 w752 w756 w757 w758 _ w759 w760 w761 w762 w763 w764 _ w765 w766 w767 w768 w769 w770 w771 _ w772 _ _ _ _ _ _ _ _ _ _ _ w773 w774 w775 w776 w777 w778 w779 _ w780 w781 w782 w783 w786 w790 w794 w797 w802 w804 w807 _ w809 w810 w811 w812 w813 w814 w815 w816 w817 _ w818 w819 w820 _ w821 w822 w823 w824 _ w825 w832 w833 w834 w835 w836 w837 w838 w839 w840 w841 w842 w843 w844 w845 w847 w850 w854 w858 w862 w866 w870 _ _ _ _ w874 w881 w882 w886 w891]
                frame 0, Default {
                }
                frame 1 {
                  n561 = local read "poreMeasuresTable"() -> (w617:string[][])
                  n562 = property on="SampleNumber" class="Str"("Caption.Text"=w609) -> ()  [unwired: 2 in, 2 out]
                  n563 = local read "grainMeasuresTable"() -> (w610:string[][])
                  n564 = Replace Array Subset(array=w617, new element=w609, index (row)=0, index (col)=1) -> (w616:string[][])
                  n565 = Replace Array Subset(array=w610, new element=w609, index (row)=0, index (col)=1) -> (w611:string[][])
                  n566 = local write "grainMeasuresTable"(w611) -> ()
                  n567 = local write "poreMeasuresTable"(w616) -> ()
                }
                frame 2 {
                  n568 = local read "poreMeasuresTable"() -> (w623:string[][])
                  n569 = property on="SampleID" class="Str"("Caption.Text"=w618) -> ()  [unwired: 2 in, 2 out]
                  n570 = local read "grainMeasuresTable"() -> (w619:string[][])
                  n571 = Replace Array Subset(array=w623, new element=w618, index (row)=0, index (col)=2) -> (w626:string[][])
                  n572 = local write "poreMeasuresTable"(w626) -> ()
                  n573 = Replace Array Subset(array=w619, new element=w618, index (row)=0, index (col)=2) -> (w620:string[][])
                  n574 = local write "grainMeasuresTable"(w620) -> ()
                }
                frame 3 {
                  n575 = property on="SampleDepth" class="DigNum (strict)"("Caption.Text"=w627) -> ()  [unwired: 2 in, 2 out]
                  n576 = local read "poreMeasuresTable"() -> (w632:string[][])
                  n577 = local read "grainMeasuresTable"() -> (w628:string[][])
                  n578 = Replace Array Subset(array=w628, new element=w627, index (row)=0, index (col)=3) -> (w629:string[][])
                  n579 = Replace Array Subset(array=w632, new element=w627, index (row)=0, index (col)=3) -> (w635:string[][])
                  n580 = local write "grainMeasuresTable"(w629) -> ()
                  n581 = local write "poreMeasuresTable"(w635) -> ()
                }
                frame 4 {
                  n582 = local read "poreMeasuresTable"() -> (w644:string[][])
                  n583 = local read "grainMeasuresTable"() -> (w637:string[][])
                  n584 = property on="DryWeight" class="DigNum (strict)"("Caption.Text"=w636) -> ()  [unwired: 2 in, 2 out]
                  n585 = Replace Array Subset(array=w637, new element=w636, index (row)=0, index (col)=4) -> (w638:string[][])
                  n586 = Replace Array Subset(array=w644, new element=w636, index (row)=0, index (col)=4) -> (w643:string[][])
                  n587 = local write "grainMeasuresTable"(w638) -> ()
                  n588 = local write "poreMeasuresTable"(w643) -> ()
                }
                frame 5 {
                  n589 = property on="BulkVolume" class="DigNum (strict)"("Caption.Text"=w645) -> ()  [unwired: 2 in, 2 out]
                  n590 = local read "poreMeasuresTable"() -> (w653:string[][])
                  n591 = local read "grainMeasuresTable"() -> (w646:string[][])
                  n592 = Replace Array Subset(array=w646, new element=w645, index (row)=0, index (col)=5) -> (w647:string[][])
                  n593 = Replace Array Subset(array=w653, new element=w645, index (row)=0, index (col)=5) -> (w652:string[][])
                  n594 = local write "grainMeasuresTable"(w647) -> ()
                  n595 = local write "poreMeasuresTable"(w652) -> ()
                }
                frame 6 {
                  n596 = local read "poreMeasuresTable"() -> (w662:string[][])
                  n597 = local read "grainMeasuresTable"() -> (w655:string[][])
                  n598 = Replace Array Subset(array=w655, new element=w654, index (row)=0, index (col)=6) -> (w656:string[][])
                  n599 = Replace Array Subset(array=w662, new element=w654, index (row)=0, index (col)=6) -> (w661:string[][])
                  n600 = local write "grainMeasuresTable"(w656) -> ()
                  n601 = local write "poreMeasuresTable"(w661) -> ()
                }
                frame 7 {
                  n602 = local read "poreMeasuresTable"() -> (w667:string[][])
                  n603 = Replace Array Subset(array=w667, new element=w663, index (row)=0, index (col)=7) -> (w666:string[][])
                  n604 = local write "poreMeasuresTable"(w666) -> ()
                }
                frame 8 {
                  n605 = local read "poreMeasuresTable"() -> (w672:string[][])
                  n606 = Replace Array Subset(array=w672, new element=w668, index (row)=0, index (col)=8) -> (w671:string[][])
                  n607 = local write "poreMeasuresTable"(w671) -> ()
                }
                frame 9 {
                  n608 = local read "poreMeasuresTable"() -> (w681:string[][])
                  n609 = local read "grainMeasuresTable"() -> (w674:string[][])
                  n610 = Replace Array Subset(array=w681, new element=w673, index (row)=0, index (col)=9) -> (w680:string[][])
                  n611 = Replace Array Subset(array=w674, new element=w673, index (row)=0, index (col)=7) -> (w675:string[][])
                  n612 = local write "grainMeasuresTable"(w675) -> ()
                  n613 = local write "poreMeasuresTable"(w680) -> ()
                }
                frame 10 {
                  n614 = local read "poreMeasuresTable"() -> (w690:string[][])
                  n615 = local read "grainMeasuresTable"() -> (w683:string[][])
                  n616 = Replace Array Subset(array=w683, new element=w682, index (row)=0, index (col)=8) -> (w684:string[][])
                  n617 = Replace Array Subset(array=w690, new element=w682, index (row)=0, index (col)=10) -> (w689:string[][])
                  n618 = local write "poreMeasuresTable"(w689) -> ()
                  n619 = local write "grainMeasuresTable"(w684) -> ()
                }
                frame 11 {
                  n620 = local read "poreMeasuresTable"() -> (w699:string[][])
                  n621 = local read "grainMeasuresTable"() -> (w692:string[][])
                  n622 = Replace Array Subset(array=w692, new element=w691, index (row)=0, index (col)=9) -> (w693:string[][])
                  n623 = Replace Array Subset(array=w699, new element=w691, index (row)=0, index (col)=11) -> (w698:string[][])
                  n624 = local write "grainMeasuresTable"(w693) -> ()
                  n625 = local write "poreMeasuresTable"(w698) -> ()
                }
                frame 12 {
                  n626 = local read "poreMeasuresTable"() -> (w708:string[][])
                  n627 = local read "grainMeasuresTable"() -> (w701:string[][])
                  n628 = Replace Array Subset(array=w701, new element=w700, index (row)=0, index (col)=10) -> (w702:string[][])
                  n629 = Replace Array Subset(array=w708, new element=w700, index (row)=0, index (col)=12) -> (w707:string[][])
                  n630 = local write "poreMeasuresTable"(w707) -> ()
                  n631 = local write "grainMeasuresTable"(w702) -> ()
                }
                frame 13 {
                  n632 = property on="Temperature" class="DigNum (strict)"("Caption.Text"=w709) -> ()  [unwired: 2 in, 2 out]
                  n633 = local read "poreMeasuresTable"() -> (w717:string[][])
                  n634 = local read "grainMeasuresTable"() -> (w710:string[][])
                  n635 = Replace Array Subset(array=w717, new element=w709, index (row)=0, index (col)=13) -> (w716:string[][])
                  n636 = Replace Array Subset(array=w710, new element=w709, index (row)=0, index (col)=11) -> (w711:string[][])
                  n637 = local write "grainMeasuresTable"(w711) -> ()
                  n638 = local write "poreMeasuresTable"(w716) -> ()
                }
                frame 14 {
                  n639 = property on="Comments" class="Str"("Caption.Text"=w718) -> ()  [unwired: 2 in, 2 out]
                  n640 = local read "poreMeasuresTable"() -> (w726:string[][])
                  n641 = local read "grainMeasuresTable"() -> (w719:string[][])
                  n642 = Replace Array Subset(array=w719, new element=w718, index (row)=0, index (col)=12) -> (w720:string[][])
                  n643 = Replace Array Subset(array=w726, new element=w718, index (row)=0, index (col)=14) -> (w725:string[][])
                  n644 = local write "grainMeasuresTable"(w720) -> ()
                  n645 = local write "poreMeasuresTable"(w725) -> ()
                }
                frame 15 {
                }
                frame 16 {
                }
                frame 17 {
                }
                frame 18 {
                }
                frame 19 {
                }
                frame 20 {
                }
                frame 21 {
                }
                frame 22 {
                }
                frame 23 {
                }
                frame 24 {
                  n646 = property on="AppTab" class="TabCtl (strict)"() -> ("Pages"=w731:refnum<vi>[])  [unwired: 2 in, 2 out]
                  n647 = Index Array(array=w731, index=0) -> (element=w729:refnum<vi>)
                  n648 = property class="Page"(reference=w729, "IndependentLabel"=TRUE, "TabCaption"=w727) -> ()  [unwired: 1 in, 2 out]
                }
                frame 25 {
                  n649 = property on="AppTab" class="TabCtl (strict)"() -> ("Pages"=w734:refnum<vi>[])  [unwired: 2 in, 2 out]
                  n650 = Index Array(array=w734, index=1) -> (element=w735:refnum<vi>)
                  n651 = property class="Page"(reference=w735, "IndependentLabel"=TRUE, "TabCaption"=w733) -> ()  [unwired: 1 in, 2 out]
                }
                frame 26 {
                  n652 = property on="AppTab" class="TabCtl (strict)"() -> ("Pages"=w739:refnum<vi>[])  [unwired: 2 in, 2 out]
                  n653 = Index Array(array=w739, index=2) -> (element=w740:refnum<vi>)
                  n654 = property class="Page"(reference=w740, "IndependentLabel"=TRUE, "TabCaption"=w738) -> ()  [unwired: 1 in, 2 out]
                }
                frame 27 {
                }
                frame 28 {
                  n655 = property on="strInstallName" class="Str"("Value"=w742) -> ()  [unwired: 2 in, 2 out]
                }
                frame 29 {
                  n656 = property on="btnExit" class="Bool (strict)"("BoolText.Text"=w743) -> ()  [unwired: 2 in, 2 out]
                }
                frame 30 {
                  n657 = property on="btnEtal" class="Bool (strict)"("BoolText.Text"=w744) -> ()  [unwired: 2 in, 2 out]
                }
                frame 31 {
                  n658 = property on="btnMesurePore" class="Bool (strict)"("BoolText.Text"=w745) -> ()  [unwired: 2 in, 2 out]
                }
                frame 32 {
                  n659 = property on="btnVidanger" class="Bool (strict)"("BoolText.Text"=w746) -> ()  [unwired: 2 in, 2 out]
                  n660 = property on="manualModeBtn" class="Bool (strict)"("Value"=FALSE) -> ()  [unwired: 2 in, 2 out]
                }
                frame 33 {
                  n661 = property on="manualModeBtn" class="Bool (strict)"() -> ("Strings [4]"=w751:string[])  [unwired: 2 in, 2 out]
                  n662 = Replace Array Subset(array=w751, new element=w748, index=0) -> (w750:string[])
                  n663 = property on="manualModeBtn" class="Bool (strict)"("Strings [4]"=w750) -> ()  [unwired: 2 in, 2 out]
                }
                frame 34 {
                  n664 = property on="manualModeBtn" class="Bool (strict)"() -> ("Strings [4]"=w755:string[])  [unwired: 2 in, 2 out]
                  n665 = Replace Array Subset(array=w755, new element=w752, index=1) -> (w754:string[])
                  n666 = property on="manualModeBtn" class="Bool (strict)"("Strings [4]"=w754) -> ()  [unwired: 2 in, 2 out]
                }
                frame 35 {
                  n667 = property on="Helium Tank" class="Str"("Caption.Text"=w756) -> ()  [unwired: 2 in, 2 out]
                }
                frame 36 {
                  n668 = property on="Ref1" class="Str"("Caption.Text"=w757) -> ()  [unwired: 2 in, 2 out]
                }
                frame 37 {
                  n669 = property on="Ref2" class="Str"("Caption.Text"=w758) -> ()  [unwired: 2 in, 2 out]
                }
                frame 38 {
                }
                frame 39 {
                  n670 = property on="V1Ind" class="Bool (strict)"("Caption.Text"=w759) -> ()  [unwired: 2 in, 2 out]
                }
                frame 40 {
                  n671 = property on="V2Ind" class="Bool (strict)"("Caption.Text"=w760) -> ()  [unwired: 2 in, 2 out]
                }
                frame 41 {
                  n672 = property on="Sample ValveInd" class="Bool (strict)"("Caption.Text"=w761) -> ()  [unwired: 2 in, 2 out]
                }
                frame 42 {
                  n673 = property on="Inlet ValveInd" class="Bool (strict)"("Caption.Text"=w762) -> ()  [unwired: 2 in, 2 out]
                }
                frame 43 {
                  n674 = property on="Outlet ValveInd" class="Bool (strict)"("Caption.Text"=w763) -> ()  [unwired: 2 in, 2 out]
                }
                frame 44 {
                  n675 = property on="Matrix Cup" class="Str"("Caption.Text"=w764) -> ()  [unwired: 2 in, 2 out]
                }
                frame 45 {
                }
                frame 46 {
                  n676 = property on="ReferenceCellMeasure" class="DigNum (strict)"("Caption.Text"=w765) -> ()  [unwired: 2 in, 2 out]
                }
                frame 47 {
                  n677 = property on="KeepCalibrationPoint" class="Bool (strict)"("Caption.Text"=w766) -> ()  [unwired: 2 in, 2 out]
                }
                frame 48 {
                  n678 = property on="P1P2RatioCalibration" class="DigNum (strict)"("Caption.Text"=w767) -> ()  [unwired: 2 in, 2 out]
                }
                frame 49 {
                  n679 = property on="ContinueCalibration" class="Bool (strict)"("BoolText.Text"=w768) -> ()  [unwired: 2 in, 2 out]
                }
                frame 50 {
                  n680 = property on="CalibrationVolumesTable" class="Tbl (strict)"("Caption.Text"=w769) -> ()  [unwired: 2 in, 2 out]
                }
                frame 51 {
                  n681 = property on="MachineName" class="Str"("Caption.Text"=w770) -> ()  [unwired: 2 in, 2 out]
                }
                frame 52 {
                  n682 = property on="AverageAbsoluteDeviationServices" class="DigNum (strict)"("Caption.Text"=w771) -> ()  [unwired: 2 in, 2 out]
                  n683 = property on="AverageAbsoluteDeviation" class="DigNum (strict)"("Caption.Text"=w771) -> ()  [unwired: 2 in, 2 out]
                }
                frame 53 {
                }
                frame 54 {
                  n684 = property on="mdpControl" class="Str"("Caption.Text"=w772) -> ()  [unwired: 2 in, 2 out]
                }
                frame 55 {
                }
                frame 56 {
                }
                frame 57 {
                }
                frame 58 {
                }
                frame 59 {
                }
                frame 60 {
                }
                frame 61 {
                }
                frame 62 {
                }
                frame 63 {
                }
                frame 64 {
                }
                frame 65 {
                }
                frame 66 {
                  n685 = property on="pumeActive" class="Bool (strict)"("Caption.Text"=w773) -> ()  [unwired: 2 in, 2 out]
                }
                frame 67 {
                  n686 = property on="pressureCaptorActive" class="Bool (strict)"("Caption.Text"=w774) -> ()  [unwired: 2 in, 2 out]
                }
                frame 68 {
                  n687 = property on="indicateurDefautPuissance" class="Bool (strict)"("Caption.Text"=w775) -> ()  [unwired: 2 in, 2 out]
                }
                frame 69 {
                  n688 = property on="indicateurSurpression" class="Bool (strict)"("Caption.Text"=w776) -> ()  [unwired: 2 in, 2 out]
                }
                frame 70 {
                  n689 = property on="indicateurPerteSignal" class="Bool (strict)"("Caption.Text"=w777) -> ()  [unwired: 2 in, 2 out]
                }
                frame 71 {
                  n690 = property on="rPressionM" class="DigNum (strict)"("Caption.Text"=w778) -> ()  [unwired: 2 in, 2 out]
                }
                frame 72 {
                  n691 = property on="PressureGraph" class="XYGraph (strict)"("Plot.Plot Name"=w779) -> ()  [unwired: 2 in, 2 out]
                }
                frame 73 {
                }
                frame 74 {
                  n692 = property on="MeasureDiskSet" class="LstBox (strict)"("Caption.Text"=w780) -> ()  [unwired: 2 in, 2 out]
                  n693 = property on="DiskSet" class="LstBox (strict)"("Caption.Text"=w780) -> ()  [unwired: 2 in, 2 out]
                }
                frame 77 {
                  n694 = property on="CalibrationStep" class="DigNum (strict)"("Caption.Text"=w781) -> ()  [unwired: 2 in, 2 out]
                }
                frame 78 {
                  n695 = property on="SaveCalibrationFile" class="Bool (strict)"("BoolText.Text"=w782) -> ()  [unwired: 2 in, 2 out]
                }
                frame 79 {
                  n696 = property on="RestartCalibration" class="Bool (strict)"("BoolText.Text"=w783) -> ()  [unwired: 2 in, 2 out]
                }
                frame 80 {
                  # "Idle: 0\nCalibration: 1\nMesure: 2\nVidange: 3"
                  n697 = local read "NotificationTexts"() -> (w784:string[])
                  n698 = Insert Into Array(array=w784, index=0, new element=w786) -> (w785:string[])
                  n699 = local write "NotificationTexts"(w785) -> ()
                }
                frame 81 {
                  # "Idle: 0\nCalibration: 1\nMesure: 2\nVidange: 3"
                  n700 = local read "NotificationTexts"() -> (w789:string[])
                  n701 = Insert Into Array(array=w789, index=1, new element=w790) -> (w788:string[])
                  n702 = local write "NotificationTexts"(w788) -> ()
                }
                frame 82 {
                  # "Idle: 0\nCalibration: 1\nMesure: 2\nVidange: 3"
                  n703 = local read "NotificationTexts"() -> (w792:string[])
                  n704 = Insert Into Array(array=w792, index=2, new element=w794) -> (w793:string[])
                  n705 = local write "NotificationTexts"(w793) -> ()
                }
                frame 83 {
                  # "Idle: 0\nCalibration: 1\nMesure: 2\nVidange: 3"
                  n706 = local read "NotificationTexts"() -> (w796:string[])
                  n707 = Insert Into Array(array=w796, index=3, new element=w797) -> (w798:string[])
                  n708 = local write "NotificationTexts"(w798) -> ()
                }
                frame 84 {
                  # "Idle: 0\nCalibration: 1\nMesure: 2\nVidange: 3"
                  n709 = local read "NotificationTexts"() -> (w800:string[])
                  n710 = Insert Into Array(array=w800, index=4, new element=w802) -> (w801:string[])
                  n711 = local write "NotificationTexts"(w801) -> ()
                }
                frame 85 {
                  n712 = local write "MeasureReportedString"(w804) -> ()
                }
                frame 86 {
                  # "Idle: 0\nCalibration: 1\nMesure: 2\nVidange: 3"
                  n713 = local read "NotificationTexts"() -> (w806:string[])
                  n714 = Insert Into Array(array=w806, index=6, new element=w807) -> (w805:string[])
                  n715 = local write "NotificationTexts"(w805) -> ()
                }
                frame 87 {
                }
                frame 88 {
                  n716 = property on="PurgeState" class="Str"("Text.Text"=w809) -> ()  [unwired: 2 in, 2 out]
                }
                frame 89 {
                  n717 = property on="PressureCaptorConfig" class="Clust (strict)"("Caption.Text"=w810) -> ()  [unwired: 2 in, 2 out]
                }
                frame 90 {
                  n718 = property on="ValvesConfig" class="Clust (strict)"("Caption.Text"=w811) -> ()  [unwired: 2 in, 2 out]
                }
                frame 91 {
                  n719 = property on="Valve mapping" class="Clust (strict)"("Caption.Text"=w812) -> ()  [unwired: 2 in, 2 out]
                }
                frame 92 {
                  n720 = property on="SleeveConfiguration" class="Clust (strict)"("Caption.Text"=w813) -> ()  [unwired: 2 in, 2 out]
                }
                frame 93 {
                  n721 = property on="Pressure Offset" class="DigNum (strict)"("Caption.Text"=w814) -> ()  [unwired: 2 in, 2 out]
                }
                frame 94 {
                  n722 = property on="Pressure Gain" class="DigNum (strict)"("Caption.Text"=w815) -> ()  [unwired: 2 in, 2 out]
                }
                frame 95 {
                  n723 = property on="SaveConfigChanges" class="Bool (strict)"("BoolText.Text"=w816) -> ()  [unwired: 2 in, 2 out]
                }
                frame 96 {
                  n724 = property on="LanguagesList" class="LstBox (strict)"("Caption.Text"=w817) -> ()  [unwired: 2 in, 2 out]
                }
                frame 97 {
                }
                frame 98 {
                  n725 = property on="XYGraphService" class="XYGraph (strict)"("Caption.Text"=w818) -> ()  [unwired: 2 in, 2 out]
                }
                frame 99 {
                  n726 = property on="FittedPolynomCoeffs" class="Arr (strict)"("Caption.Text"=w819) -> ()  [unwired: 2 in, 2 out]
                  n727 = property on="FittedPolynomCoeffsServices" class="Arr (strict)"("Caption.Text"=w819) -> ()  [unwired: 2 in, 2 out]
                }
                frame 100 {
                  n728 = property on="ResidueInd" class="DigNum (strict)"("Caption.Text"=w820) -> ()  [unwired: 2 in, 2 out]
                  n729 = property on="ResiduServices" class="DigNum (strict)"("Caption.Text"=w820) -> ()  [unwired: 2 in, 2 out]
                }
                frame 101 {
                }
                frame 102 {
                  n730 = property on="CalibrationFilePath" class="Path"("Caption.Text"=w821) -> ()  [unwired: 2 in, 2 out]
                }
                frame 103 {
                  n731 = property on="LoadCalibrationFileBtn" class="Bool (strict)"("BoolText.Text"=w822) -> ()  [unwired: 2 in, 2 out]
                }
                frame 104 {
                  n732 = property on="MeasureDiskVolumes" class="LstBox (strict)"("Caption.Text"=w823) -> ()  [unwired: 2 in, 2 out]
                  n733 = property on="AvalaibleVolumesList" class="LstBox (strict)"("Caption.Text"=w823) -> ()  [unwired: 2 in, 2 out]
                }
                frame 105 {
                  n734 = property on="MeasureTotalAddedVolume" class="DigNum (strict)"("Caption.Text"=w824) -> ()  [unwired: 2 in, 2 out]
                  n735 = property on="VolumeOfCalibrationMeasure" class="DigNum (strict)"("Caption.Text"=w824) -> ()  [unwired: 2 in, 2 out]
                  n736 = property on="ChosenVolume" class="DigNum (strict)"("Caption.Text"=w824) -> ()  [unwired: 2 in, 2 out]
                }
                frame 106 {
                }
                frame 107 {
                  n737 = property on="DoMeasureCalibration" class="Bool (strict)"() -> ("Strings [4]"=w830:string[])  [unwired: 2 in, 2 out]
                  n738 = property on="DoMeasureMeasure" class="Bool (strict)"() -> ("Strings [4]"=w827:string[])  [unwired: 2 in, 2 out]
                  n739 = Replace Array Subset(array=w830, new element=w825, index=0) -> (w829:string[])
                  n740 = Replace Array Subset(array=w827, new element=w825, index=0) -> (w826:string[])
                  n741 = property on="DoMeasureCalibration" class="Bool (strict)"("Strings [4]"=w829) -> ()  [unwired: 2 in, 2 out]
                  n742 = property on="DoMeasureMeasure" class="Bool (strict)"("Strings [4]"=w826) -> ()  [unwired: 2 in, 2 out]
                }
                frame 108 {
                  n743 = property on="EndCalibration" class="Bool (strict)"("BoolText.Text"=w832) -> ()  [unwired: 2 in, 2 out]
                }
                frame 109 {
                  n744 = property on="poreMeasuresTable" class="Tbl (strict)"("Caption.Text"=w833) -> ()  [unwired: 2 in, 2 out]
                }
                frame 110 {
                  n745 = property on="ClearGrainMeasuresBtn" class="Bool (strict)"("BoolText.Text"=w834) -> ()  [unwired: 2 in, 2 out]
                  n746 = property on="ClearPoreMeasuresBtn" class="Bool (strict)"("BoolText.Text"=w834) -> ()  [unwired: 2 in, 2 out]
                }
                frame 111 {
                  n747 = property on="ExportToHTMLBtn" class="Bool (strict)"("BoolText.Text"=w835) -> ()  [unwired: 2 in, 2 out]
                }
                frame 112 {
                  n748 = property on="ExportGrainMeasuresBtn" class="Bool (strict)"("BoolText.Text"=w836) -> ()  [unwired: 2 in, 2 out]
                  n749 = property on="ExportPoreMeasuresBtn" class="Bool (strict)"("BoolText.Text"=w836) -> ()  [unwired: 2 in, 2 out]
                }
                frame 113 {
                  n750 = property on="SaveGrainMeasuresBtn" class="Bool (strict)"("BoolText.Text"=w837) -> ()  [unwired: 2 in, 2 out]
                  n751 = property on="SavePoreMeasuresBtn" class="Bool (strict)"("BoolText.Text"=w837) -> ()  [unwired: 2 in, 2 out]
                }
                frame 114 {
                  n752 = property on="LoadGrainMeasuresBtn" class="Bool (strict)"("BoolText.Text"=w838) -> ()  [unwired: 2 in, 2 out]
                  n753 = property on="LoadPoreMeasuresBtn" class="Bool (strict)"("BoolText.Text"=w838) -> ()  [unwired: 2 in, 2 out]
                }
                frame 115 {
                  n754 = property on="FlushPressureGraph" class="Bool (strict)"("BoolText.Text"=w839) -> ()  [unwired: 2 in, 2 out]
                }
                frame 116 {
                  n755 = property on="ExportToPDF" class="Bool (strict)"("BoolText.Text"=w840) -> ()  [unwired: 2 in, 2 out]
                }
                frame 117 {
                  n756 = property on="MaximalWaitTime" class="DigNum (strict)"("Caption.Text"=w841) -> ()  [unwired: 2 in, 2 out]
                }
                frame 118 {
                  n757 = property on="MinimalWaitTime" class="DigNum (strict)"("Caption.Text"=w842) -> ()  [unwired: 2 in, 2 out]
                }
                frame 119 {
                  n758 = property on="VarianceTrigger" class="DigNum (strict)"("Caption.Text"=w843) -> ()  [unwired: 2 in, 2 out]
                }
                frame 120 {
                  n759 = property on="SamplesMasks" class="Arr (strict)"("Caption.Text"=w844) -> ()  [unwired: 2 in, 2 out]
                }
                frame 121 {
                  n760 = property on="ClearGrainMeasureBtn" class="Bool (strict)"("BoolText.Text"=w845) -> ()  [unwired: 2 in, 2 out]
                  n761 = property on="ClearPoreMeasureBtn" class="Bool (strict)"("BoolText.Text"=w845) -> ()  [unwired: 2 in, 2 out]
                }
                frame 122 {
                  n762 = global read "MeasureExportStrings.vi" "MeasureExportStrings"() -> (w848:string[])
                  n763 = property on="Company" class="Str"("Caption.Text"=w847) -> ()  [unwired: 2 in, 2 out]
                  n764 = Replace Array Subset(array=w848, new element=w847, index=8) -> (w849:string[])
                  n765 = global write "MeasureExportStrings.vi" "MeasureExportStrings"(w849) -> ()
                }
                frame 123 {
                  n766 = global read "MeasureExportStrings.vi" "MeasureExportStrings"() -> (w852:string[])
                  n767 = property on="Location" class="Str"("Caption.Text"=w850) -> ()  [unwired: 2 in, 2 out]
                  n768 = Replace Array Subset(array=w852, new element=w850, index=4) -> (w853:string[])
                  n769 = global write "MeasureExportStrings.vi" "MeasureExportStrings"(w853) -> ()
                }
                frame 124 {
                  n770 = global read "MeasureExportStrings.vi" "MeasureExportStrings"() -> (w856:string[])
                  n771 = property on="Country" class="Str"("Caption.Text"=w854) -> ()  [unwired: 2 in, 2 out]
                  n772 = Replace Array Subset(array=w856, new element=w854, index=9) -> (w857:string[])
                  n773 = global write "MeasureExportStrings.vi" "MeasureExportStrings"(w857) -> ()
                }
                frame 125 {
                  n774 = global read "MeasureExportStrings.vi" "MeasureExportStrings"() -> (w860:string[])
                  n775 = Replace Array Subset(array=w860, new element=w858, index=10) -> (w861:string[])
                  n776 = property on="Lab" class="Str"("Caption.Text"=w858) -> ()  [unwired: 2 in, 2 out]
                  n777 = global write "MeasureExportStrings.vi" "MeasureExportStrings"(w861) -> ()
                }
                frame 126 {
                  n778 = global read "MeasureExportStrings.vi" "MeasureExportStrings"() -> (w864:string[])
                  n779 = property on="Operator" class="Str"("Caption.Text"=w862) -> ()  [unwired: 2 in, 2 out]
                  n780 = Replace Array Subset(array=w864, new element=w862, index=12) -> (w865:string[])
                  n781 = global write "MeasureExportStrings.vi" "MeasureExportStrings"(w865) -> ()
                }
                frame 127 {
                  n782 = global read "MeasureExportStrings.vi" "MeasureExportStrings"() -> (w868:string[])
                  n783 = Replace Array Subset(array=w868, new element=w866, index=6) -> (w869:string[])
                  n784 = property on="Field" class="Str"("Caption.Text"=w866) -> ()  [unwired: 2 in, 2 out]
                  n785 = global write "MeasureExportStrings.vi" "MeasureExportStrings"(w869) -> ()
                }
                frame 128 {
                  n786 = global read "MeasureExportStrings.vi" "MeasureExportStrings"() -> (w872:string[])
                  n787 = Replace Array Subset(array=w872, new element=w870, index=3) -> (w873:string[])
                  n788 = property on="Well" class="Str"("Caption.Text"=w870) -> ()  [unwired: 2 in, 2 out]
                  n789 = global write "MeasureExportStrings.vi" "MeasureExportStrings"(w873) -> ()
                }
                frame 129 {
                }
                frame 130 {
                }
                frame 131 {
                }
                frame 132 {
                }
                frame 133 {
                  n790 = property on="DoMeasureCalibration" class="Bool (strict)"() -> ("Strings [4]"=w879:string[])  [unwired: 2 in, 2 out]
                  n791 = property on="DoMeasureMeasure" class="Bool (strict)"() -> ("Strings [4]"=w876:string[])  [unwired: 2 in, 2 out]
                  n792 = Replace Array Subset(array=w879, new element=w874, index=1) -> (w878:string[])
                  n793 = Replace Array Subset(array=w876, new element=w874, index=1) -> (w875:string[])
                  n794 = property on="DoMeasureCalibration" class="Bool (strict)"("Strings [4]"=w878) -> ()  [unwired: 2 in, 2 out]
                  n795 = property on="DoMeasureMeasure" class="Bool (strict)"("Strings [4]"=w875) -> ()  [unwired: 2 in, 2 out]
                }
                frame 134 {
                  n796 = property on="Correlation" class="DigNum (strict)"("Caption.Text"=w881) -> ()  [unwired: 2 in, 2 out]
                  n797 = property on="CorrelationServices" class="DigNum (strict)"("Caption.Text"=w881) -> ()  [unwired: 2 in, 2 out]
                }
                frame 135 {
                  n798 = property on="btnMesureGrain" class="Bool (strict)"() -> ("Strings [4]"=w885:string[])  [unwired: 2 in, 2 out]
                  n799 = Replace Array Subset(array=w885, new element=w882, index=0) -> (w884:string[])
                  n800 = property on="btnMesureGrain" class="Bool (strict)"("Strings [4]"=w884) -> ()  [unwired: 2 in, 2 out]
                }
                frame 136 {
                  n801 = property on="MeasuresTabs" class="TabCtl (strict)"() -> ("Pages"=w890:refnum<vi>[])  [unwired: 2 in, 2 out]
                  n802 = Index Array(array=w890, index=0) -> (element=w888:refnum<vi>)
                  n803 = property class="Page"(reference=w888, "IndependentLabel"=TRUE, "TabCaption"=w886) -> ()  [unwired: 1 in, 2 out]
                }
                frame 137 {
                  n804 = property on="MeasuresTabs" class="TabCtl (strict)"() -> ("Pages"=w895:refnum<vi>[])  [unwired: 2 in, 2 out]
                  n805 = Index Array(array=w895, index=1) -> (element=w893:refnum<vi>)
                  n806 = property class="Page"(reference=w893, "IndependentLabel"=TRUE, "TabCaption"=w891) -> ()  [unwired: 1 in, 2 out]
                }
              }
            }
            n807 = local read "LanguagesList"() -> (w597:i32)
            n808 = Unbundle(w599) -> ("SupportedLanguagesList"=w596:string[], "LocalisationFileContent[out]"=w598:T21)  [unwired: 2 out]
            n809 = Index Array(array=w596, index=w597) -> (element=w595:string)
            n810 = Bundle("SupportedLanguagesList"=w596, "String"=w595, "LanguagesList"=w597, "LocalisationFileContent[out]"=w598) -> (w600:T31)  [unwired: 1 in]
            n811 = global write "LanguagesSettings.vi" "LanguageSettings"(w600) -> ()
          }
          event "SavePoreMeasuresBtn": Value Change {
            n812 = event-data() -> ("NewVal"=w898:bool)  [unwired: 1 in, 5 out]
            n813 = case shown="True" w898 {
              frame False {
              }
              frame True {
                n814 = flat-sequence {
                  frame #0 {
                    n815 = local write "MeasureMode"(MeasureModeControl."PoreMeasure" ("MeasureMode")) -> ()
                  }
                  frame #1 {
                    n816 = property on="SaveData" class="Bool (strict)"("Val(Sgnl)"=TRUE ("Value (Signaling)")) -> ()  [unwired: 2 in, 2 out]
                  }
                }
              }
            }
          }
          event "LoadPoreMeasuresBtn": Value Change {
            n817 = event-data() -> ("NewVal"=w902:bool)  [unwired: 1 in, 5 out]
            n818 = case shown="True" w902 {
              frame False {
              }
              frame True {
                n819 = flat-sequence {
                  frame #0 {
                    n820 = local write "MeasureMode"(MeasureModeControl."PoreMeasure" ("MeasureMode")) -> ()
                  }
                  frame #1 {
                    n821 = property on="LoadData" class="Bool (strict)"("Val(Sgnl)"=TRUE ("Value (Signaling)")) -> ()  [unwired: 2 in, 2 out]
                  }
                }
              }
            }
          }
          event "FlushPressureGraph": Value Change {
            n822 = event-data() -> ("NewVal"=w906:bool)  [unwired: 1 in, 5 out]
            n823 = case shown="True" w906 {
              frame False {
              }
              frame True {
                n824 = local write "FlushPressureGraph"(FALSE ("FlushPressureGraph")) -> ()
                n825 = global read "PressureAndTimeSamples.vi" "PressureAndTimeSamples"() -> (w912:T3)
                n826 = Unbundle(w912) -> ("TimeSamples"=w911:dbl[])  [unwired: 1 out]
                n827 = Array Size(array=w911) -> (size(s)=w908:i32)
                n828 = Greater Than 0?(x=w908) -> (x > 0?=w910:bool)
                n829 = case shown="False" w910 {
                  tunnel: w908 -> [_ w914]
                  tunnel: [0 w914] -> w909
                  frame False {
                  }
                  frame True {
                  }
                }
                n830 = local write "FirstGraphSampleIndex"(w909) -> ()
              }
            }
          }
          event "mdpControl": Value Change {
            n831 = event-data() -> ("NewVal"=w924:string)  [unwired: 1 in, 5 out]
            n832 = call <vilib>:"Application Directory.vi"() -> ("Application Directory"=w934:path)
            n833 = Build Path(base path=w934, name or relative path=path "config.ini" ("default name")) -> (appended path=w935:path)
            n834 = call <vilib>:"Open Config Data.vi"("error in (no error)"=w930, "create file if necessary (T)"=FALSE ("create file if necessary? (T)"), "configuration file path"=w935) -> ("error out"=w933:errorcluster, "refnum"=w932:T32)  [unwired: 6 in, 1 out]
            n835 = call-poly <vilib>:"Read Key.vi"("section"="System", "error in (no error)"=w933, "key"="password", "refnum"=w932) -> ("error out"=w927:errorcluster, "value"=w917:string, "refnum out"=w926:T32)  [unwired: 4 in, 1 out]
            n836 = String Length(string=w917) -> (length=w922:i32)
            n837 = call <vilib>:"Close Config Data.vi"("error in (no error)"=w927, "write file if changed (T)"=TRUE ("write configuration file? (T)"), "refnum"=w926) -> ("error out"=w925:errorcluster)  [unwired: 8 out]
            n838 = Quotient & Remainder(x=w922, y=2) -> (floor(x/y)=w921:i32)  [unwired: 1 out]
            n839 = for {
              N: w921 -> [_]
              tunnel: w917 -> [w939]
              tunnel: [w938] -> w919 mode=indexing
              i -> [w942]
              n840 = Add(x=w942, y=w942) -> (x+y=w941:i32)
              n841 = String Subset(string=w939, offset (0)=w941, length (rest)=2 ("length (rest)")) -> (substring=w938:string)
            }
            n842 = Hexadecimal String To Number(string=w919, default (0uL)=u8 0 ("default (0 U32)")) -> (number=w918:u8[])  [unwired: 1 in, 1 out]
            n843 = Byte Array To String(unsigned byte array=w918) -> (string=w916:string)
            n844 = Equal?(x=w916, y=w924) -> (x = y?=w915:bool)
            n845 = property on="ServiceButtonsVisible" class="Bool (strict)"("Val(Sgnl)"=w915) -> ()  [unwired: 2 in, 2 out]
          }
          event "CalibrationVolumesTable": Value Change {
            n846 = event-data() -> ("NewVal"=w943:string[][])  [unwired: 1 in, 5 out]
            n847 = flat-sequence {
              tunnel: w943 -> [w944]
              frame #0 {
                n848 = call "WriteTableToCalibrationVolumes.vi"("NewVal"=w944) -> ()  [unwired: 11 in]
              }
              frame #1 {
                n849 = property on="ReloadDiskVolumes" class="Bool (strict)"("Val(Sgnl)"=TRUE ("Value (Signaling)")) -> ()  [unwired: 2 in, 2 out]
              }
            }
          }
          event "manualModeBtn": Value Change {
            n850 = event-data() -> ("NewVal"=w946:bool)  [unwired: 1 in, 5 out]
            n851 = property on="V2Btn" class="Bool (strict)"("Visible"=w946) -> ()  [unwired: 2 in, 2 out]
            n852 = property on="V1Btn" class="Bool (strict)"("Visible"=w946) -> ()  [unwired: 2 in, 2 out]
            n853 = property on="Inlet ValveBtn" class="Bool (strict)"("Visible"=w946) -> ()  [unwired: 2 in, 2 out]
            n854 = property on="Sample ValveBtn" class="Bool (strict)"("Visible"=w946) -> ()  [unwired: 2 in, 2 out]
            n855 = property on="Outlet ValveBtn" class="Bool (strict)"("Visible"=w946) -> ()  [unwired: 2 in, 2 out]
          }
          event "V1Btn": Value Change {
            n856 = event-data() -> ("OldVal"=w950:bool)  [unwired: 1 in, 5 out]
            n857 = local read "manualModeBtn"() -> (w948:bool)
            n858 = case shown="True" w948 {
              tunnel: w950 -> [w952 _]
              tunnel: w947 -> [w951 w953]
              tunnel: [w951 w954] -> w949
              frame False {
                n859 = local write "V1Btn"(w952) -> ()
              }
              frame True {
                n860 = global read "ValveParameters.vi" "ValveParameters"() -> (w956:T11)
                n861 = Unbundle By Name(w956) -> ("Valve mapping.V1"=w955:u8)
                n862 = local read "V1Btn"() -> (w957:bool)
                n863 = call "SetValve.vi"("error in"=w953, "ON"=w957, "Valve"=w955) -> ("error out"=w954:errorcluster)  [unwired: 8 in]
              }
            }
          }
          event "V2Btn": Value Change {
            n864 = event-data() -> ("OldVal"=w961:bool)  [unwired: 1 in, 5 out]
            n865 = local read "manualModeBtn"() -> (w958:bool)
            n866 = case shown="False" w958 {
              tunnel: w961 -> [w962 _]
              tunnel: w960 -> [w963 w968]
              tunnel: [w963 w967] -> w959
              frame False {
                n867 = local write "V2Btn"(w962) -> ()
              }
              frame True {
                n868 = global read "ValveParameters.vi" "ValveParameters"() -> (w966:T11)
                n869 = Unbundle By Name(w966) -> ("Valve mapping.V2"=w964:u8)
                n870 = local read "V2Btn"() -> (w965:bool)
                n871 = call "SetValve.vi"("error in"=w968, "ON"=w965, "Valve"=w964) -> ("error out"=w967:errorcluster)  [unwired: 8 in]
              }
            }
          }
          event "Inlet ValveBtn": Value Change {
            n872 = event-data() -> ("OldVal"=w970:bool)  [unwired: 1 in, 5 out]
            n873 = local read "manualModeBtn"() -> (w969:bool)
            n874 = case shown="True" w969 {
              tunnel: w970 -> [w973 _]
              tunnel: w972 -> [w974 w979]
              tunnel: [w974 w978] -> w971
              frame False {
                n875 = local write "Inlet ValveBtn"(w973) -> ()
              }
              frame True {
                n876 = global read "ValveParameters.vi" "ValveParameters"() -> (w977:T11)
                n877 = Unbundle By Name(w977) -> ("Valve mapping.Inlet Valve"=w975:u8)
                n878 = local read "Inlet ValveBtn"() -> (w976:bool)
                n879 = call "SetValve.vi"("error in"=w979, "ON"=w976, "Valve"=w975) -> ("error out"=w978:errorcluster)  [unwired: 8 in]
              }
            }
          }
          event "Outlet ValveBtn": Value Change {
            n880 = event-data() -> ("OldVal"=w982:bool)  [unwired: 1 in, 5 out]
            n881 = local read "manualModeBtn"() -> (w980:bool)
            n882 = case shown="True" w980 {
              tunnel: w982 -> [w984 _]
              tunnel: w983 -> [w985 w990]
              tunnel: [w985 w989] -> w981
              frame False {
                n883 = local write "Outlet ValveBtn"(w984) -> ()
              }
              frame True {
                n884 = global read "ValveParameters.vi" "ValveParameters"() -> (w988:T11)
                n885 = Unbundle By Name(w988) -> ("Valve mapping.Outlet Valve"=w986:u8)
                n886 = local read "Outlet ValveBtn"() -> (w987:bool)
                n887 = call "SetValve.vi"("error in"=w990, "ON"=w987, "Valve"=w986) -> ("error out"=w989:errorcluster)  [unwired: 8 in]
              }
            }
          }
          event "Sample ValveBtn": Value Change {
            n888 = event-data() -> ("OldVal"=w993:bool)  [unwired: 1 in, 5 out]
            n889 = local read "manualModeBtn"() -> (w991:bool)
            n890 = case shown="True" w991 {
              tunnel: w993 -> [w995 _]
              tunnel: w994 -> [w996 w1001]
              tunnel: [w996 w1000] -> w992
              frame False {
                n891 = local write "Sample ValveBtn"(w995) -> ()
              }
              frame True {
                n892 = global read "ValveParameters.vi" "ValveParameters"() -> (w999:T11)
                n893 = Unbundle By Name(w999) -> ("Valve mapping.Sample Valve"=w998:u8)
                n894 = local read "Sample ValveBtn"() -> (w997:bool)
                n895 = call "SetValve.vi"("error in"=w1001, "ON"=w997, "Valve"=w998) -> ("error out"=w1000:errorcluster)  [unwired: 8 in]
              }
            }
          }
          event "btnEtal": Value Change {
            n896 = event-data() -> ("NewVal"=w1002:bool)  [unwired: 1 in, 5 out]
            n897 = case shown="True" w1002 {
              frame False {
              }
              frame True {
                n898 = stacked-sequence {
                  frame #0 {
                    # "On désactive ici\nle mode manuel\npour qu'il prenne bien effet\n(si app state n'est pas idle,\npas traité)"
                    n899 = property on="manualModeBtn" class="Bool (strict)"("Val(Sgnl)"=FALSE) -> ()  [unwired: 2 in, 2 out]
                  }
                  frame #1 {
                    # "Calibration state"
                    n900 = global read "CalibrationState.vi" "CalibrationState"() -> (w1004:T9)
                    n901 = global write "AppState.vi" "AppState"(u16 1) -> ()
                    n902 = Unbundle By Name(w1004) -> ("CalibrationStep"=w1005:u32)
                    n903 = Unbundle(w1004) -> ("CalibrationStep"=w1010:u32, "Volumes"=w1009:dbl[], "PressureRatios"=w1008:dbl[], "Weights"=w1007:bool[])  [unwired: 1 out]
                    n904 = Bundle(FALSE, "CalibrationStep"=w1010, "Volumes"=w1009, "PressureRatios"=w1008, "Weights"=w1007) -> (w1011:T9)  [unwired: 1 in]
                    n905 = local write "CalibrationStep"(w1005) -> ()
                    n906 = global write "CalibrationState.vi" "CalibrationState"(w1011) -> ()
                  }
                  frame #2 {
                    w1013 = TRUE ("Value (Signaling)")
                    w1014 = FALSE ("Value (Signaling)")
                    # "Fait la transition vers l'état de calibration:\nactive et désactive les bouttons nécessaires"
                    n907 = property on="CalibrationButtonsVisible" class="Bool (strict)"("Val(Sgnl)"=w1013) -> ()  [unwired: 2 in, 2 out]
                    n908 = property on="UpdateServiceGraph" class="Bool (strict)"("Val(Sgnl)"=w1013) -> ()  [unwired: 2 in, 2 out]
                    n909 = property on="ChangeMenuState" class="Bool (strict)"("Val(Sgnl)"=w1013) -> ()  [unwired: 2 in, 2 out]
                    n910 = property on="ReloadDiskVolumes" class="Bool (strict)"("Val(Sgnl)"=w1013) -> ()  [unwired: 2 in, 2 out]
                    n911 = property on="MeasureIndicatorsVisible" class="Bool (strict)"("Val(Sgnl)"=w1014) -> ()  [unwired: 2 in, 2 out]
                    n912 = property on="CalibrationResultsVisible" class="Bool (strict)"("Val(Sgnl)"=w1014) -> ()  [unwired: 2 in, 2 out]
                    n913 = property on="ExportMeasuresButtonsVisible" class="Bool (strict)"("Val(Sgnl)"=w1014) -> ()  [unwired: 2 in, 2 out]
                    n914 = property on="PurgeState" class="Str"("Visible"=w1014) -> ()  [unwired: 2 in, 2 out]
                    n915 = property on="MeasureSetupButtonsVisible" class="Bool (strict)"("Val(Sgnl)"=w1014) -> ()  [unwired: 2 in, 2 out]
                  }
                }
              }
            }
          }
          event "ContinueCalibration": Value Change {
            n916 = event-data() -> ("NewVal"=w1015:bool)  [unwired: 1 in, 5 out]
            n917 = case shown="True" w1015 {
              frame False {
              }
              frame True {
                n918 = stacked-sequence {
                  frame #0 {
                    n919 = global read "CalibrationState.vi" "CalibrationState"() -> (w1029:T9)
                    n920 = local read "VolumeOfCalibrationMeasure"() -> (w1019:dbl)
                    n921 = local write "ContinueCalibration"(FALSE ("ContinueCalibration")) -> ()
                    n922 = local read "P1P2RatioCalibration"() -> (w1021:dbl)
                    n923 = local read "KeepCalibrationPoint"() -> (w1022:bool)
                    n924 = property on="btnEtal" class="Bool (strict)"("Val(Sgnl)"=TRUE ("Value (Signaling)")) -> ()  [unwired: 2 in, 2 out]
                    n925 = Unbundle(w1029) -> (w1027:bool, "CalibrationStep"=w1026:u32, "Volumes"=w1024:dbl[], "PressureRatios"=w1023:dbl[], "Weights"=w1020:bool[])
                    n926 = Increment(x=w1026) -> (x+1=w1025:u32)
                    n927 = Insert Into Array(array=w1024, new element=w1019) -> (w1018:dbl[])  [unwired: 1 in]
                    n928 = Insert Into Array(array=w1023, new element=w1021) -> (w1017:dbl[])  [unwired: 1 in]
                    n929 = Insert Into Array(array=w1020, new element=w1022) -> (w1016:bool[])  [unwired: 1 in]
                    n930 = property on="SingleCalibrationMeasureButtonsVisible" class="Bool (strict)"("Val(Sgnl)"=FALSE ("Value (Signaling)")) -> ()  [unwired: 2 in, 2 out]
                    n931 = Bundle(w1027, w1025, "Volumes"=w1018, "PressureRatios"=w1017, "Weights"=w1016) -> (w1028:T33)  [unwired: 1 in]
                    n932 = global write "CalibrationState.vi" "CalibrationState"(w1028) -> ()
                  }
                  frame #1 {
                    w1033 = FALSE ("Value (Signaling)")
                    # "pour simuler le \"appui puis relache\""
                    n933 = property on="UpdateServiceGraph" class="Bool (strict)"("Val(Sgnl)"=w1033) -> ()  [unwired: 2 in, 2 out]
                    n934 = property on="btnEtal" class="Bool (strict)"("Value"=w1033) -> ()  [unwired: 2 in, 2 out]
                  }
                }
              }
            }
          }
          event "RestartCalibration": Value Change {
            n935 = event-data() -> ()  [unwired: 1 in, 6 out]
            n936 = flat-sequence {
              frame #0 {
                n937 = property on="btnEtal" class="Bool (strict)"("Val(Sgnl)"=TRUE ("Value (Signaling)")) -> ()  [unwired: 2 in, 2 out]
              }
              frame #1 {
                n938 = property on="btnEtal" class="Bool (strict)"("Value"=FALSE ("btnEtal")) -> ()  [unwired: 2 in, 2 out]
              }
            }
            n939 = global write "CalibrationState.vi" "CalibrationState"(T9 {FALSE, "CalibrationStep"=0, "Volumes"=[], "PressureRatios"=[], "Weights"=[]} ("CalibrationState")) -> ()
          }
          event "DiskSet": Value Change {
            n940 = event-data() -> ()  [unwired: 1 in, 6 out]
            n941 = property on="ReloadDiskVolumes" class="Bool (strict)"("Val(Sgnl)"=TRUE ("Value (Signaling)")) -> ()  [unwired: 2 in, 2 out]
          }
          event "MeasureDiskSet": Value Change {
            n942 = event-data() -> ()  [unwired: 1 in, 6 out]
            n943 = property on="ReloadDiskVolumes" class="Bool (strict)"("Val(Sgnl)"=TRUE ("Value (Signaling)")) -> ()  [unwired: 2 in, 2 out]
          }
          event "AvalaibleVolumesList": Value Change {
            n944 = event-data() -> ()  [unwired: 1 in, 6 out]
            n945 = global read "AppState.vi" "AppState"() -> (w1039:u16)
            n946 = Equal?(x=w1039, y=u16 1) -> (x = y?=w1041:bool)
            n947 = case shown="True" w1041 {
              frame False {
              }
              frame True {
                n948 = local read "AvalaibleVolumesList"() -> (w1044:i32[])
                n949 = Array Size(array=w1044) -> (size(s)=w1045:i32)
                n950 = for {
                  N: w1045 -> [_]
                  tunnel: w1044 -> [w1050] mode=indexing
                  shift-right: [w1046] -> w1042
                  shift-left: 0.0 -> [w1048]
                  n951 = global read "CalibrationVolumes.vi" "AllCalibrationVolumes"() -> (w1054:T18)
                  n952 = local read "DiskSet"() -> (w1047:i32)
                  n953 = To Long Integer(number=w1047) -> (32bit integer=w1053:i32)
                  n954 = Index Array(array=w1054, index=w1053) -> (element=w1052:T23)
                  n955 = Unbundle(w1052) -> ("CalibrationVolumes"=w1051:dbl[])  [unwired: 2 out]
                  n956 = Index Array(array=w1051, index=w1050) -> (element=w1049:dbl)
                  n957 = Add(x=w1048, y=w1049) -> (x+y=w1046:dbl)
                }
                n958 = property on="ChosenVolume" class="DigNum (strict)"("Val(Sgnl)"=w1042) -> ()  [unwired: 2 in, 2 out]
              }
            }
          }
          event "MeasureDiskVolumes": Value Change {
            n959 = event-data() -> ()  [unwired: 1 in, 6 out]
            n960 = local read "MeasureDiskVolumes"() -> (w1058:i32[])
            n961 = Array Size(array=w1058) -> (size(s)=w1055:i32)
            n962 = for {
              N: w1055 -> [_]
              tunnel: w1058 -> [w1063] mode=indexing
              shift-right: [w1060] -> w1057
              shift-left: 0.0 -> [w1061]
              n963 = local read "MeasureDiskSet"() -> (w1059:i32)
              n964 = global read "CalibrationVolumes.vi" "AllCalibrationVolumes"() -> (w1067:T18)
              n965 = To Long Integer(number=w1059) -> (32bit integer=w1066:i32)
              n966 = Index Array(array=w1067, index=w1066) -> (element=w1065:T23)
              n967 = Unbundle(w1065) -> ("CalibrationVolumes"=w1064:dbl[])  [unwired: 2 out]
              n968 = Index Array(array=w1064, index=w1063) -> (element=w1062:dbl)
              n969 = Add(x=w1061, y=w1062) -> (x+y=w1060:dbl)
            }
            n970 = property on="MeasureTotalAddedVolume" class="DigNum (strict)"("Val(Sgnl)"=w1057) -> ()  [unwired: 2 in, 2 out]
          }
          event "DoMeasureCalibration": Value Change {
            n971 = event-data() -> ("NewVal"=w1070:bool)  [unwired: 1 in, 5 out]
            n972 = global read "AppState.vi" "AppState"() -> (w1072:u16)
            n973 = Equal?(x=w1072, y=u16 1) -> (x = y?=w1071:bool)
            n974 = And(x=w1071, y=w1070) -> (x .and. y?=w1074:bool)
            n975 = case shown="True" w1074 {
              tunnel: w1069 -> [w1075 w1077]
              tunnel: [w1075 w1076] -> w1068
              frame False {
              }
              frame True {
                n976 = stacked-sequence {
                  tunnel: w1077 -> [_ w1087 _ _]
                  tunnel: [_ w1086 _ _] -> w1076
                  frame #0 {
                    n977 = global write "AppState.vi" "AppState"(4) -> ()
                    n978 = property on="DoMeasureCalibration" class="Bool (strict)"("DisabledEnum"=T8."Disabled" ("Disabled")) -> ()  [unwired: 2 in, 2 out]
                    n979 = property on="manualModeBtn" class="Bool (strict)"("DisabledEnum"=T8."Disabled and Grayed Out" ("Disabled"), "Val(Sgnl)"=FALSE ("Value (Signaling)")) -> ()  [unwired: 2 in, 2 out]
                  }
                  frame #1 {
                    n980 = local read "ReferenceCellMeasure"() -> (w1082:u16)
                    n981 = local read "ChosenVolume"() -> (w1085:dbl)
                    n982 = global read "PressureAndTimeSamples.vi" "PressureAndTimeSamples"() -> (w1089:T3)
                    n983 = local write "VolumeOfCalibrationMeasure"(w1085) -> ()
                    n984 = To Long Integer(number=w1082) -> (32bit integer=w1090:i32)
                    n985 = call "Measure.vi"("Graph in"=w1089, "error in"=w1087, "Reference Cell"=w1090) -> ("error out"=w1086:errorcluster, "Values"=w1088:cluster{dbl[], dbl[]}, "P1/P2"=w1084:dbl, "StabilityAchieved"=w1083:bool)  [unwired: 5 in]
                    n986 = global write "PressureAndTimeSamples.vi" "PressureAndTimeSamples"(w1088) -> ()
                    n987 = local write "StabilityAchieved"(w1083) -> ()
                    n988 = local write "P1P2RatioCalibration"(w1084) -> ()
                  }
                  frame #2 {
                    n989 = global write "AppState.vi" "AppState"(1) -> ()
                    n990 = property on="DoMeasureCalibration" class="Bool (strict)"("Value"=FALSE ("DoCalibrationMeasure")) -> ()  [unwired: 2 in, 2 out]
                    n991 = property on="manualModeBtn" class="Bool (strict)"("DisabledEnum"=T8."Enabled" ("Disabled")) -> ()  [unwired: 2 in, 2 out]
                  }
                  frame #3 {
                    n992 = global read "LanguagesSettings.vi" "LanguageSettings"() -> (w1099:T13)
                    n993 = Unbundle By Name(w1099) -> ("LocalisationFileContent[out]"=w1100:T21)
                    n994 = local read "StabilityAchieved"() -> (w1094:bool)
                    n995 = local read "LanguagesList"() -> (w1096:i32)
                    n996 = property on="CalibrationButtonsVisible" class="Bool (strict)"("Val(Sgnl)"=FALSE ("Value (Signaling)")) -> ()  [unwired: 2 in, 2 out]
                    n997 = property on="SingleCalibrationMeasureButtonsVisible" class="Bool (strict)"("Val(Sgnl)"=TRUE ("Value (Signaling)")) -> ()  [unwired: 2 in, 2 out]
                    n998 = case shown="True" w1094 {
                      tunnel: [u32 131 ("WordIndex") u32 130 ("WordIndex")] -> w1101
                      frame False {
                      }
                      frame True {
                      }
                    }
                    n999 = call "FindLocalizedString.vi"("LangIndex"=w1096, "LocalizationFileContent"=w1100, "WordIndex"=w1101) -> ("Found"=w1097:bool, "LocalizedString"=w1098:string)  [unwired: 7 in]
                    n1000 = case shown="False" w1097 {
                      tunnel: w1098 -> [_ w1107]
                      tunnel: ["Not found" w1107] -> w1095
                      frame False {
                      }
                      frame True {
                      }
                    }
                    n1001 = property on="calibrationStabilization" class="Str"("Text.Text"=w1095) -> ()  [unwired: 2 in, 2 out]
                  }
                }
              }
            }
          }
          event "ClearPoreMeasuresBtn": Value Change {
            n1002 = event-data() -> ("NewVal"=w1108:bool)  [unwired: 1 in, 5 out]
            n1003 = case shown="True" w1108 {
              frame False {
              }
              frame True {
                n1004 = stacked-sequence {
                  frame #0 {
                    n1005 = property on="poreMeasuresTable" class="Tbl (strict)"("Number of Columns"=u32 15, "Number of Rows"=u32 1) -> ()  [unwired: 2 in, 2 out]
                  }
                  frame #1 {
                    n1006 = property on="poreMeasuresTable" class="Tbl (strict)"("Size"=T10 {"Width"=828, "Height"=205}) -> ()  [unwired: 2 in, 2 out]
                  }
                  frame #2 {
                    n1007 = property on="ReloadResultTableTexts" class="Bool (strict)"("Val(Sgnl)"=TRUE ("Value (Signaling)")) -> ()  [unwired: 2 in, 2 out]
                    n1008 = property on="ClearPoreMeasuresBtn" class="Bool (strict)"("Value"=FALSE ("ClearMeasuresBtn")) -> ()  [unwired: 2 in, 2 out]
                  }
                }
              }
            }
          }
          event "ClearGrainMeasuresBtn": Value Change {
            n1009 = event-data() -> ("NewVal"=w1114:bool)  [unwired: 1 in, 5 out]
            n1010 = case shown="True" w1114 {
              frame False {
              }
              frame True {
                n1011 = stacked-sequence {
                  frame #0 {
                    n1012 = property on="grainMeasuresTable" class="Tbl (strict)"("Number of Columns"=u32 12, "Number of Rows"=u32 1) -> ()  [unwired: 2 in, 2 out]
                  }
                  frame #1 {
                    n1013 = property on="grainMeasuresTable" class="Tbl (strict)"("Size"=T10 {"Width"=828, "Height"=205}) -> ()  [unwired: 2 in, 2 out]
                  }
                  frame #2 {
                    n1014 = property on="ReloadResultTableTexts" class="Bool (strict)"("Val(Sgnl)"=TRUE ("Value (Signaling)")) -> ()  [unwired: 2 in, 2 out]
                    n1015 = property on="ClearGrainMeasuresBtn" class="Bool (strict)"("Value"=FALSE ("ClearMeasuresBtn")) -> ()  [unwired: 2 in, 2 out]
                  }
                }
              }
            }
          }
          event "ExportToHTMLBtn": Value Change {
            n1016 = event-data() -> ("NewVal"=w1122:bool)  [unwired: 1 in, 5 out]
            n1017 = case shown="True" w1122 {
              tunnel: w1121 -> [w1123 w1126]
              tunnel: [w1123 w1125] -> w1120
              frame False {
              }
              frame True {
                n1018 = flat-sequence {
                  tunnel: w1126 -> [w1132]
                  tunnel: [w1131] -> w1124
                  tunnel: w1124 -> [w1137]
                  tunnel: [w1137] -> w1125
                  frame #0 {
                    n1019 = local read "MeasureMode"() -> (w1128:T1)
                    n1020 = Equal?(x=MeasureModeControl."PoreMeasure", y=w1128) -> (x = y?=w1129:bool)
                    n1021 = case shown="False" w1129 {
                      tunnel: [w1133 w1134] -> w1130
                      frame False {
                        n1022 = control-ref of="grainMeasuresTable"() -> (w1133:refnum<vi>)
                      }
                      frame True {
                        n1023 = control-ref of="poreMeasuresTable"() -> (w1134:refnum<vi>)
                      }
                    }
                    n1024 = call "ExportMeasuresToHTML.vi"("error in (no error)"=w1132, "MeasureMode"=w1128, "Table in"=w1130) -> ("error out"=w1131:errorcluster)  [unwired: 8 in]
                  }
                  frame #1 {
                    n1025 = property on="ExportMeasuresButtonsVisible" class="Bool (strict)"("Val(Sgnl)"=FALSE ("Value (Signaling)")) -> ()  [unwired: 2 in, 2 out]
                    n1026 = local write "ExportToHTMLBtn"(FALSE ("ExportToHTMLBtn")) -> ()
                  }
                }
              }
            }
          }
          event "ClearPoreMeasureBtn": Value Change {
            n1027 = event-data() -> ("NewVal"=w1138:bool)  [unwired: 1 in, 5 out]
            n1028 = case shown="True" w1138 {
              frame False {
              }
              frame True {
                n1029 = flat-sequence {
                  frame #0 {
                    n1030 = local write "MeasureMode"(MeasureModeControl."PoreMeasure" ("MeasureMode")) -> ()
                  }
                  frame #1 {
                    n1031 = property on="DeleteMeasureLine" class="Bool (strict)"("Val(Sgnl)"=TRUE ("Value (Signaling)")) -> ()  [unwired: 2 in, 2 out]
                  }
                }
              }
            }
          }
          event "ClearGrainMeasureBtn": Value Change {
            n1032 = event-data() -> ("NewVal"=w1141:bool)  [unwired: 1 in, 5 out]
            n1033 = case shown="True" w1141 {
              frame False {
              }
              frame True {
                n1034 = flat-sequence {
                  frame #0 {
                    n1035 = local write "MeasureMode"(MeasureModeControl."GrainMeasure" ("MeasureMode")) -> ()
                  }
                  frame #1 {
                    n1036 = property on="DeleteMeasureLine" class="Bool (strict)"("Val(Sgnl)"=TRUE ("Value (Signaling)")) -> ()  [unwired: 2 in, 2 out]
                  }
                }
              }
            }
          }
          event "DeleteMeasureLine": Value Change {
            n1037 = event-data() -> ("NewVal"=w1144:bool)  [unwired: 1 in, 5 out]
            n1038 = case shown="True" w1144 {
              frame False {
              }
              frame True {
                n1039 = local read "MeasureMode"() -> (w1153:T1)
                n1040 = Equal?(x=w1153, y=MeasureModeControl."GrainMeasure") -> (x = y?=w1154:bool)
                n1041 = case shown="False" w1154 {
                  tunnel: [w1170 w1171] -> w1150
                  tunnel: [w1170 w1171] -> w1149
                  frame False {
                    n1042 = control-ref of="poreMeasuresTable"() -> (w1170:refnum<vi>)
                  }
                  frame True {
                    n1043 = control-ref of="grainMeasuresTable"() -> (w1171:refnum<vi>)
                  }
                }
                n1044 = property class="Tbl (strict)"(reference=w1149) -> ("Selection Start"=w1148:T34)  [unwired: 1 in, 2 out]
                n1045 = property class="Tbl (strict)"(reference=w1150) -> ("Value"=w1151:string[][])  [unwired: 1 in, 2 out]
                n1046 = Unbundle By Name(w1148) -> ("Row"=w1146:i32)
                n1047 = Greater?(x=w1146, y=0) -> (0:w1147:bool)
                n1048 = case shown="True" w1147 {
                  tunnel: w1151 -> [_ w1166]
                  tunnel: w1150 -> [_ w1156]
                  tunnel: w1147 -> [_ _]
                  tunnel: w1146 -> [_ w1155]
                  frame False {
                  }
                  frame True {
                    w1169 = 0 ("index")
                    n1049 = Increment(x=w1155) -> (x+1=w1162:i32)
                    n1050 = Array Size(array=w1166) -> (size(s)=w1165:i32[])
                    n1051 = Index Array(array=w1165, index=0) -> (element=w1163:i32)
                    n1052 = Subtract(x=w1163, y=w1162) -> (x-y=w1161:i32)
                    n1053 = Index Array(array=w1165, index=1) -> (element=w1159:i32)
                    n1054 = Array Subset(array=w1166, index (row)=w1169, length (row)=w1155, index (col)=w1169, length (col)=w1159) -> (w1167:string[][])
                    n1055 = Array Subset(array=w1166, index (row)=w1162, length (row)=w1161, index (col)=0 ("index"), length (col)=w1159) -> (w1158:string[][])
                    n1056 = Insert Into Array(array=w1167, new element=w1158) -> (w1157:string[][])  [unwired: 2 in]
                    n1057 = property class="Tbl (strict)"(reference=w1156, "Value"=w1157) -> ()  [unwired: 1 in, 2 out]
                  }
                }
              }
            }
          }
          event "ExportToPDF": Value Change {
            n1058 = event-data() -> ("NewVal"=w1174:bool)  [unwired: 1 in, 5 out]
            n1059 = case shown="True" w1174 {
              tunnel: w1173 -> [w1175 w1177]
              tunnel: [w1175 w1176] -> w1172
              frame False {
              }
              frame True {
                n1060 = flat-sequence {
                  tunnel: w1177 -> [w1183]
                  tunnel: [w1182] -> w1176
                  frame #0 {
                    n1061 = local read "MeasureMode"() -> (w1179:T1)
                    n1062 = Equal?(x=MeasureModeControl."PoreMeasure", y=w1179) -> (x = y?=w1180:bool)
                    n1063 = case shown="False" w1180 {
                      tunnel: [w1184 w1185] -> w1181
                      frame False {
                        n1064 = control-ref of="grainMeasuresTable"() -> (w1184:refnum<vi>)
                      }
                      frame True {
                        n1065 = control-ref of="poreMeasuresTable"() -> (w1185:refnum<vi>)
                      }
                    }
                    n1066 = call "ExportMeasuresToPDF.vi"("error in (no error)"=w1183, "MeasureMode"=w1179, "Table in"=w1181) -> ("error out"=w1182:errorcluster)  [unwired: 8 in]
                  }
                  frame #1 {
                    n1067 = local write "ExportToPDF"(FALSE ("ExportToPDF")) -> ()
                    n1068 = property on="ExportMeasuresButtonsVisible" class="Bool (strict)"("Val(Sgnl)"=FALSE ("Value (Signaling)")) -> ()  [unwired: 2 in, 2 out]
                  }
                }
              }
            }
          }
          event "ExportPoreMeasuresBtn": Value Change {
            n1069 = event-data() -> ("NewVal"=w1188:bool)  [unwired: 1 in, 5 out]
            n1070 = case shown="True" w1188 {
              frame False {
              }
              frame True {
                n1071 = flat-sequence {
                  frame #0 {
                    n1072 = local write "MeasureMode"(MeasureModeControl."PoreMeasure" ("MeasureMode")) -> ()
                  }
                  frame #1 {
                    n1073 = property on="ExportData" class="Bool (strict)"("Val(Sgnl)"=TRUE ("Value (Signaling)")) -> ()  [unwired: 2 in, 2 out]
                  }
                }
              }
            }
          }
          event "LoadGrainMeasuresBtn": Value Change {
            n1074 = event-data() -> ("NewVal"=w1191:bool)  [unwired: 1 in, 5 out]
            n1075 = case shown="True" w1191 {
              frame False {
              }
              frame True {
                n1076 = flat-sequence {
                  frame #0 {
                    n1077 = local write "MeasureMode"(MeasureModeControl."GrainMeasure" ("MeasureMode")) -> ()
                  }
                  frame #1 {
                    n1078 = property on="LoadData" class="Bool (strict)"("Val(Sgnl)"=TRUE ("Value (Signaling)")) -> ()  [unwired: 2 in, 2 out]
                  }
                }
              }
            }
          }
          event "SaveGrainMeasuresBtn": Value Change {
            n1079 = event-data() -> ("NewVal"=w1194:bool)  [unwired: 1 in, 5 out]
            n1080 = case shown="True" w1194 {
              frame False {
              }
              frame True {
                n1081 = flat-sequence {
                  frame #0 {
                    n1082 = local write "MeasureMode"(MeasureModeControl."GrainMeasure" ("MeasureMode")) -> ()
                  }
                  frame #1 {
                    n1083 = property on="SaveData" class="Bool (strict)"("Val(Sgnl)"=TRUE ("Value (Signaling)")) -> ()  [unwired: 2 in, 2 out]
                  }
                }
              }
            }
          }
          event "ExportGrainMeasuresBtn": Value Change {
            n1084 = event-data() -> ("NewVal"=w1197:bool)  [unwired: 1 in, 5 out]
            n1085 = case shown="True" w1197 {
              frame False {
              }
              frame True {
                n1086 = flat-sequence {
                  frame #0 {
                    n1087 = local write "MeasureMode"(MeasureModeControl."GrainMeasure" ("MeasureMode")) -> ()
                  }
                  frame #1 {
                    n1088 = property on="ExportData" class="Bool (strict)"("Val(Sgnl)"=TRUE ("Value (Signaling)")) -> ()  [unwired: 2 in, 2 out]
                  }
                }
              }
            }
          }
          event "Location": Value Change {
            n1089 = event-data() -> ("NewVal"=w1200:string)  [unwired: 1 in, 5 out]
            n1090 = global read "UserInfos.vi" "UserInfos"() -> (w1211:T35)
            n1091 = Unbundle(w1211) -> ("Field"=w1209:string, "Company"=w1208:string, "Lab"=w1207:string, "Operator"=w1206:string, "Well"=w1205:string, "Lat/Long"=w1204:string, "Formation"=w1203:string, "Country"=w1202:string, "Client"=w1201:string)  [unwired: 1 out]
            n1092 = Bundle("NewVal"=w1200, "Field"=w1209, "Company"=w1208, "Lab"=w1207, "Operator"=w1206, "Well"=w1205, "Lat/Long"=w1204, "Formation"=w1203, "Country"=w1202, "Client"=w1201) -> (w1210:T36)  [unwired: 1 in]
            n1093 = global write "UserInfos.vi" "UserInfos"(w1210) -> ()
          }
          event "Field": Value Change {
            n1094 = event-data() -> ("NewVal"=w1220:string)  [unwired: 1 in, 5 out]
            n1095 = global read "UserInfos.vi" "UserInfos"() -> (w1223:T35)
            n1096 = Unbundle(w1223) -> ("location"=w1221:string, "Company"=w1219:string, "Lab"=w1218:string, "Operator"=w1217:string, "Well"=w1216:string, "Lat/Long"=w1215:string, "Formation"=w1214:string, "Country"=w1213:string, "Client"=w1212:string)  [unwired: 1 out]
            n1097 = Bundle("location"=w1221, "NewVal"=w1220, "Company"=w1219, "Lab"=w1218, "Operator"=w1217, "Well"=w1216, "Lat/Long"=w1215, "Formation"=w1214, "Country"=w1213, "Client"=w1212) -> (w1222:T37)  [unwired: 1 in]
            n1098 = global write "UserInfos.vi" "UserInfos"(w1222) -> ()
          }
          event "Company": Value Change {
            n1099 = event-data() -> ("NewVal"=w1231:string)  [unwired: 1 in, 5 out]
            n1100 = global read "UserInfos.vi" "UserInfos"() -> (w1234:T35)
            n1101 = Unbundle(w1234) -> ("location"=w1233:string, "Field"=w1232:string, "Lab"=w1230:string, "Operator"=w1229:string, "Well"=w1228:string, "Lat/Long"=w1227:string, "Formation"=w1226:string, "Country"=w1225:string, "Client"=w1224:string)  [unwired: 1 out]
            n1102 = Bundle("location"=w1233, "Field"=w1232, "NewVal"=w1231, "Lab"=w1230, "Operator"=w1229, "Well"=w1228, "Lat/Long"=w1227, "Formation"=w1226, "Country"=w1225, "Client"=w1224) -> (w1235:T38)  [unwired: 1 in]
            n1103 = global write "UserInfos.vi" "UserInfos"(w1235) -> ()
          }
          event "Lab": Value Change {
            n1104 = event-data() -> ("NewVal"=w1242:string)  [unwired: 1 in, 5 out]
            n1105 = global read "UserInfos.vi" "UserInfos"() -> (w1247:T35)
            n1106 = Unbundle(w1247) -> ("location"=w1245:string, "Field"=w1244:string, "Company"=w1243:string, "Operator"=w1241:string, "Well"=w1240:string, "Lat/Long"=w1239:string, "Formation"=w1238:string, "Country"=w1237:string, "Client"=w1236:string)  [unwired: 1 out]
            n1107 = Bundle("location"=w1245, "Field"=w1244, "Company"=w1243, "NewVal"=w1242, "Operator"=w1241, "Well"=w1240, "Lat/Long"=w1239, "Formation"=w1238, "Country"=w1237, "Client"=w1236) -> (w1246:T39)  [unwired: 1 in]
            n1108 = global write "UserInfos.vi" "UserInfos"(w1246) -> ()
          }
          event "ChosenVolume": Value Change {
            n1109 = event-data() -> ()  [unwired: 1 in, 6 out]
            n1110 = global read "AppState.vi" "AppState"() -> (w1249:u16)
            n1111 = Equal?(x=w1249, y=u16 1) -> (x = y?=w1250:bool)
            n1112 = case shown="True" w1250 {
              frame False {
              }
              frame True {
                n1113 = property on="DoMeasureCalibration" class="Bool (strict)"("DisabledEnum"=T8."Enabled" ("Disabled")) -> ()  [unwired: 2 in, 2 out]
              }
            }
          }
          event "Operator": Value Change {
            n1114 = event-data() -> ("NewVal"=w1257:string)  [unwired: 1 in, 5 out]
            n1115 = global read "UserInfos.vi" "UserInfos"() -> (w1263:T35)
            n1116 = Unbundle(w1263) -> ("location"=w1261:string, "Field"=w1260:string, "Company"=w1259:string, "Lab"=w1258:string, "Well"=w1256:string, "Lat/Long"=w1255:string, "Formation"=w1254:string, "Country"=w1253:string, "Client"=w1252:string)  [unwired: 1 out]
            n1117 = Bundle("location"=w1261, "Field"=w1260, "Company"=w1259, "Lab"=w1258, "NewVal"=w1257, "Well"=w1256, "Lat/Long"=w1255, "Formation"=w1254, "Country"=w1253, "Client"=w1252) -> (w1262:T40)  [unwired: 1 in]
            n1118 = global write "UserInfos.vi" "UserInfos"(w1262) -> ()
          }
          event "Well": Value Change {
            n1119 = event-data() -> ("NewVal"=w1268:string)  [unwired: 1 in, 5 out]
            n1120 = global read "UserInfos.vi" "UserInfos"() -> (w1275:T35)
            n1121 = Unbundle(w1275) -> ("location"=w1273:string, "Field"=w1272:string, "Company"=w1271:string, "Lab"=w1270:string, "Operator"=w1269:string, "Lat/Long"=w1267:string, "Formation"=w1266:string, "Country"=w1264:string, "Client"=w1265:string)  [unwired: 1 out]
            n1122 = Bundle("location"=w1273, "Field"=w1272, "Company"=w1271, "Lab"=w1270, "Operator"=w1269, "NewVal"=w1268, "Lat/Long"=w1267, "Formation"=w1266, "Country"=w1264, "Client"=w1265) -> (w1274:T41)  [unwired: 1 in]
            n1123 = global write "UserInfos.vi" "UserInfos"(w1274) -> ()
          }
          event "LatitudeLongitude": Value Change {
            n1124 = event-data() -> ("NewVal"=w1279:string)  [unwired: 1 in, 5 out]
            n1125 = global read "UserInfos.vi" "UserInfos"() -> (w1286:T35)
            n1126 = Unbundle(w1286) -> ("location"=w1285:string, "Field"=w1284:string, "Company"=w1283:string, "Lab"=w1282:string, "Operator"=w1281:string, "Well"=w1280:string, "Formation"=w1278:string, "Country"=w1277:string, "Client"=w1276:string)  [unwired: 1 out]
            n1127 = Bundle("location"=w1285, "Field"=w1284, "Company"=w1283, "Lab"=w1282, "Operator"=w1281, "Well"=w1280, "NewVal"=w1279, "Formation"=w1278, "Country"=w1277, "Client"=w1276) -> (w1287:T42)  [unwired: 1 in]
            n1128 = global write "UserInfos.vi" "UserInfos"(w1287) -> ()
          }
          event "Formation": Value Change {
            n1129 = event-data() -> ("NewVal"=w1290:string)  [unwired: 1 in, 5 out]
            n1130 = global read "UserInfos.vi" "UserInfos"() -> (w1299:T35)
            n1131 = Unbundle(w1299) -> ("location"=w1297:string, "Field"=w1296:string, "Company"=w1295:string, "Lab"=w1294:string, "Operator"=w1293:string, "Well"=w1292:string, "Lat/Long"=w1291:string, "Country"=w1289:string, "Client"=w1288:string)  [unwired: 1 out]
            n1132 = Bundle("location"=w1297, "Field"=w1296, "Company"=w1295, "Lab"=w1294, "Operator"=w1293, "Well"=w1292, "Lat/Long"=w1291, "NewVal"=w1290, "Country"=w1289, "Client"=w1288) -> (w1298:T43)  [unwired: 1 in]
            n1133 = global write "UserInfos.vi" "UserInfos"(w1298) -> ()
          }
          event "Country": Value Change {
            n1134 = event-data() -> ("NewVal"=w1301:string)  [unwired: 1 in, 5 out]
            n1135 = global read "UserInfos.vi" "UserInfos"() -> (w1310:T35)
            n1136 = Unbundle(w1310) -> ("location"=w1309:string, "Field"=w1308:string, "Company"=w1307:string, "Lab"=w1306:string, "Operator"=w1305:string, "Well"=w1304:string, "Lat/Long"=w1303:string, "Formation"=w1302:string, "Client"=w1300:string)  [unwired: 1 out]
            n1137 = Bundle("location"=w1309, "Field"=w1308, "Company"=w1307, "Lab"=w1306, "Operator"=w1305, "Well"=w1304, "Lat/Long"=w1303, "Formation"=w1302, "NewVal"=w1301, "Client"=w1300) -> (w1311:T44)  [unwired: 1 in]
            n1138 = global write "UserInfos.vi" "UserInfos"(w1311) -> ()
          }
          event "Client": Value Change {
            n1139 = event-data() -> ("NewVal"=w1312:string)  [unwired: 1 in, 5 out]
            n1140 = global read "UserInfos.vi" "UserInfos"() -> (w1321:T35)
            n1141 = Unbundle(w1321) -> ("location"=w1323:string, "Field"=w1320:string, "Company"=w1319:string, "Lab"=w1318:string, "Operator"=w1316:string, "Well"=w1317:string, "Lat/Long"=w1315:string, "Formation"=w1314:string, "Country"=w1313:string)  [unwired: 1 out]
            n1142 = Bundle("location"=w1323, "Field"=w1320, "Company"=w1319, "Lab"=w1318, "Operator"=w1316, "Well"=w1317, "Lat/Long"=w1315, "Formation"=w1314, "Country"=w1313, "NewVal"=w1312) -> (w1322:T45)  [unwired: 1 in]
            n1143 = global write "UserInfos.vi" "UserInfos"(w1322) -> ()
          }
          event "EndCalibration": Value Change {
            n1144 = event-data() -> ()  [unwired: 1 in, 6 out]
            n1145 = global read "CalibrationState.vi" "CalibrationState"() -> (w1327:T9)
            n1146 = Unbundle(w1327) -> ("CalibrationStep"=w1326:u32)  [unwired: 4 out]
            n1147 = Greater Or Equal?(x=w1326, y=u32 6) -> (x >= y?=w1324:bool)
            n1148 = case shown="True" w1324 {
              frame False {
              }
              frame True {
                n1149 = stacked-sequence {
                  frame #0 {
                    n1150 = property on="ComputeCalibrationResult" class="Bool (strict)"("Val(Sgnl)"=TRUE ("Value (Signaling)")) -> ()  [unwired: 2 in, 2 out]
                  }
                  frame #1 {
                    # "On marque l'état de calibration"
                    n1151 = global read "CalibrationState.vi" "CalibrationState"() -> (w1335:T9)
                    n1152 = Unbundle(w1335) -> ("CalibrationStep"=w1331:u32, "Volumes"=w1333:dbl[], "PressureRatios"=w1332:dbl[], "Weights"=w1329:bool[])  [unwired: 1 out]
                    n1153 = Bundle(TRUE, "CalibrationStep"=w1331, "Volumes"=w1333, "PressureRatios"=w1332, "Weights"=w1329) -> (w1334:T9)  [unwired: 1 in]
                    n1154 = global write "CalibrationState.vi" "CalibrationState"(w1334) -> ()
                  }
                  frame #2 {
                    # "On repasse en mode idle"
                    n1155 = global write "AppState.vi" "AppState"(u16 0) -> ()
                  }
                  frame #3 {
                    w1338 = TRUE ("Value (Signaling)")
                    # "On affiche cache ce qu'il faut"
                    n1156 = property on="ChangeMenuState" class="Bool (strict)"("Val(Sgnl)"=w1338) -> ()  [unwired: 2 in, 2 out]
                    n1157 = property on="CalibrationResultsVisible" class="Bool (strict)"("Val(Sgnl)"=w1338) -> ()  [unwired: 2 in, 2 out]
                    n1158 = property on="CalibrationButtonsVisible" class="Bool (strict)"("Val(Sgnl)"=FALSE ("Value (Signaling)")) -> ()  [unwired: 2 in, 2 out]
                    n1159 = property on="FittedPolynomCoeffs" class="Arr (strict)"("DisabledEnum"=T8."Enabled" ("Disabled")) -> ()  [unwired: 2 in, 2 out]
                  }
                }
              }
            }
          }
          event "ComputeCalibrationResult": Value Change {
            n1160 = event-data() -> ("NewVal"=w1340:bool)  [unwired: 1 in, 5 out]
            n1161 = case shown="True" w1340 {
              frame False {
              }
              frame True {
                n1162 = stacked-sequence {
                  frame #0 {
                    # "On calcule le polynôme interpolateur"
                    n1163 = global read "CalibrationState.vi" "CalibrationState"() -> (w1351:T9)
                    n1164 = Unbundle(w1351) -> ("Volumes"=w1345:dbl[], "PressureRatios"=w1343:dbl[], "Weights"=w1344:bool[])  [unwired: 2 out]
                    n1165 = global read "FittedCurvePolynom.vi" "FittedCurvePolynom"() -> (w1352:dbl[])
                    n1166 = local read "ResiduServices"() -> (w1349:dbl)
                    n1167 = call "GetSelectedElements.vi"("Masks"=w1344, "Array[in]"=w1343) -> ("Array[out]"=w1341:dbl[])  [unwired: 9 in]
                    n1168 = call "GetSelectedElements.vi"("Masks"=w1344, "Array[in]"=w1345) -> ("Array[out]"=w1342:dbl[])  [unwired: 9 in]
                    n1169 = call "CalculerPolynome.vi"("Résidu [in]"=w1349, "e3 [in]"=1e-06, "Meilleure poly [in]"=w1352, "Y"=w1342, "X"=w1341) -> ("Résidu [out]"=w1347:dbl, "Meilleur poly [out]"=w1350:dbl[])  [unwired: 5 in]
                    n1170 = global write "FittedCurvePolynom.vi" "FittedCurvePolynom"(w1350) -> ()
                    n1171 = local write "FittedPolynomCoeffsServices"(w1350) -> ()
                    n1172 = local write "FittedPolynomCoeffs"(w1350) -> ()
                    n1173 = Square Root(x=w1347) -> (sqrt(x)=w1346:dbl)
                    n1174 = local write "ResiduServices"(w1346) -> ()
                    n1175 = local write "ResidueInd"(w1346) -> ()
                  }
                  frame #1 {
                    # "On ajoute les indicateurs de bonnes calibration (corrélation, average abs deviation)"
                    n1176 = global read "CalibrationState.vi" "CalibrationState"() -> (w1364:T9)
                    n1177 = Unbundle(w1364) -> ("Volumes"=w1355:dbl[], "PressureRatios"=w1357:dbl[], "Weights"=w1353:bool[])  [unwired: 2 out]
                    n1178 = global read "FittedCurvePolynom.vi" "FittedCurvePolynom"() -> (w1363:dbl[])
                    n1179 = call "GetSelectedElements.vi"("Masks"=w1353, "Array[in]"=w1357) -> ("Array[out]"=w1356:dbl[])  [unwired: 9 in]
                    n1180 = call "GetSelectedElements.vi"("Masks"=w1353, "Array[in]"=w1355) -> ("Array[out]"=w1354:dbl[])  [unwired: 9 in]
                    n1181 = call "Horner.vi"("Meilleure poly"=w1363, "X"=w1356) -> ("Y"=w1361:dbl[])  [unwired: 9 in]
                    n1182 = call "ArraySubstraction.vi"("Y [in]"=w1361, "X [in]"=w1354) -> ("Array[out]"=w1360:dbl[])  [unwired: 9 in]
                    n1183 = call "Correlation.vi"("Y"=w1361, "X"=w1354) -> ("c"=w1362:dbl)  [unwired: 9 in]
                    n1184 = local write "CorrelationServices"(w1362) -> ()
                    n1185 = local write "Correlation"(w1362) -> ()
                    n1186 = call "ElementWiseAbs.vi"("Array [in]"=w1360) -> ("Array[out]"=w1359:dbl[])  [unwired: 10 in]
                    n1187 = call "Mean.vi"("Array"=w1359) -> ("Mean"=w1358:dbl)  [unwired: 10 in]
                    n1188 = local write "AverageAbsoluteDeviation"(w1358) -> ()
                    n1189 = local write "AverageAbsoluteDeviationServices"(w1358) -> ()
                  }
                  frame #2 {
                    # "On actualise le graphe de service"
                    n1190 = property on="UpdateServiceGraph" class="Bool (strict)"("Val(Sgnl)"=TRUE ("Value (Signaling)")) -> ()  [unwired: 2 in, 2 out]
                  }
                }
              }
            }
          }
          event "UpdateServiceGraph": Value Change {
            n1191 = event-data() -> ()  [unwired: 1 in, 6 out]
            n1192 = global read "CalibrationState.vi" "CalibrationState"() -> (w1372:T9)
            n1193 = Unbundle(w1372) -> (w1367:bool, "Volumes"=w1369:dbl[], "PressureRatios"=w1374:dbl[], "Weights"=w1366:bool[])  [unwired: 1 out]
            n1194 = local write "SamplesMasks"(w1366) -> ()
            n1195 = call "GetSelectedElements.vi"("Masks"=w1366, "Array[in]"=w1369) -> ("Array[out]"=w1368:dbl[])  [unwired: 9 in]
            n1196 = call "GetSelectedElements.vi"("Masks"=w1366, "Array[in]"=w1374) -> ("Array[out]"=w1375:dbl[])  [unwired: 9 in]
            n1197 = case shown="True" w1367 {
              tunnel: w1375 -> [_ w1382]
              tunnel: [cluster{"Array":dbl[], "Y":dbl[]} {"Array"=[], "Y"=[]} w1380] -> w1370
              frame False {
              }
              frame True {
                n1198 = global read "FittedCurvePolynom.vi" "FittedCurvePolynom"() -> (w1378:dbl[])
                n1199 = call "Interpolate.vi"("X"=w1382, "Points interpolation"=u32 1000) -> ("Array"=w1381:dbl[])  [unwired: 9 in]
                n1200 = call "Horner.vi"("Meilleure poly"=w1378, "X"=w1381) -> ("Y"=w1379:dbl[])  [unwired: 9 in]
                n1201 = Bundle("Array"=w1381, "Y"=w1379) -> (w1380:cluster{"Array":dbl[], "Y":dbl[]})  [unwired: 1 in]
              }
            }
            n1202 = Bundle("Array[out]"=w1375, "Array[out]"=w1368) -> (w1373:cluster{"Array[out]":dbl[], "Array[out]":dbl[]})  [unwired: 1 in]
            n1203 = Build Array(w1373, w1370) -> (w1371:cluster{"Array":dbl[], "Y":dbl[]}[])
            n1204 = local write "XYGraphService"(w1371) -> ()
          }
          event "SamplesMasks": Value Change {
            n1205 = event-data() -> ("NewVal"=w1383:bool[])  [unwired: 1 in, 5 out]
            n1206 = stacked-sequence {
              tunnel: w1383 -> [w1386 _ _]
              frame #0 {
                # "Change l'état de calibration pour mettre les nouveaux masques"
                n1207 = global read "CalibrationState.vi" "CalibrationState"() -> (w1393:T9)
                n1208 = Unbundle(w1393) -> (w1391:bool, "CalibrationStep"=w1390:u32, "Volumes"=w1389:dbl[], "PressureRatios"=w1388:dbl[], "Weights"=w1387:bool[])
                n1209 = Replace Array Subset(array=w1387, new element=w1386, index=0) -> (w1384:bool[])
                n1210 = Bundle(w1391, "CalibrationStep"=w1390, "Volumes"=w1389, "PressureRatios"=w1388, "Weights"=w1384) -> (w1392:T9)  [unwired: 1 in]
                n1211 = global write "CalibrationState.vi" "CalibrationState"(w1392) -> ()
              }
              frame #1 {
                # "Recalcul le polynome si nécessaire"
                n1212 = global read "CalibrationState.vi" "CalibrationState"() -> (w1395:T9)
                n1213 = Unbundle(w1395) -> (w1394:bool)  [unwired: 4 out]
                n1214 = case shown="True" w1394 {
                  frame False {
                  }
                  frame True {
                    n1215 = property on="ComputeCalibrationResult" class="Bool (strict)"("Val(Sgnl)"=TRUE ("Value (Signaling)")) -> ()  [unwired: 2 in, 2 out]
                  }
                }
              }
              frame #2 {
                # "Dans tous les cas, met à jour le graphe de service"
                n1216 = property on="UpdateServiceGraph" class="Bool (strict)"("Val(Sgnl)"=TRUE ("Value (Signaling)")) -> ()  [unwired: 2 in, 2 out]
              }
            }
          }
          event "CalibrationFilePath": Value Change {
            n1217 = event-data() -> ("NewVal"=w1400:path)  [unwired: 1 in, 5 out]
            n1218 = Not Equal?(x=path "", y=w1400) -> (x != y?=w1401:bool)
            n1219 = case shown="False" w1401 {
              tunnel: [T8."Disabled and Grayed Out" ("Disabled") T8."Enabled" ("Disabled")] -> w1398
              frame False {
              }
              frame True {
              }
            }
            n1220 = property on="LoadCalibrationFileBtn" class="Bool (strict)"("DisabledEnum"=w1398) -> ()  [unwired: 2 in, 2 out]
          }
          event "LoadCalibrationFileBtn": Value Change {
            n1221 = event-data() -> ("NewVal"=w1406:bool)  [unwired: 1 in, 5 out]
            n1222 = case shown="False" w1406 {
              tunnel: w1405 -> [w1407 w1409]
              tunnel: [w1407 w1408] -> w1404
              frame False {
              }
              frame True {
                n1223 = stacked-sequence {
                  tunnel: w1409 -> [w1411 _ _]
                  tunnel: [w1410 _ _] -> w1408
                  frame #0 {
                    n1224 = local read "CalibrationFilePath"() -> (w1413:path)
                    n1225 = call "LoadCalibrationFile.vi"("error in (no error)"=w1411, "Path"=w1413) -> ("error out"=w1410:errorcluster, "CalibrationState"=w1412:T9)  [unwired: 8 in]
                    n1226 = global write "CalibrationState.vi" "CalibrationState"(w1412) -> ()
                  }
                  frame #1 {
                    n1227 = property on="btnEtal" class="Bool (strict)"("Val(Sgnl)"=TRUE ("Value (Signaling)")) -> ()  [unwired: 2 in, 2 out]
                  }
                  frame #2 {
                    n1228 = property on="btnEtal" class="Bool (strict)"("Value"=FALSE ("btnEtal")) -> ()  [unwired: 2 in, 2 out]
                  }
                }
              }
            }
          }
          event Timeout {
            n1229 = event-data() -> ()  [unwired: 1 in, 3 out]
          }
          event "SaveCalibrationFile": Value Change {
            n1230 = event-data() -> ("NewVal"=w1418:bool)  [unwired: 1 in, 5 out]
            n1231 = case shown="True" w1418 {
              tunnel: w1417 -> [w1419 w1425]
              tunnel: [w1419 w1422] -> w1416
              frame False {
              }
              frame True {
                n1232 = Default Directory() -> (w1426:path)
                n1233 = call "File Dialog3"("start path"=w1426, "default name"="calibration.txt", "error in"=w1425, "pattern (all files)"="*.txt") -> ("selected path"=w1423:path, "cancelled"=w1420:bool, "error out"=w1424:errorcluster)  [unwired: 8 in, 1 out]
                n1234 = Not(x=w1420) -> (.not. x?=w1421:bool)
                n1235 = case shown="True" w1421 {
                  tunnel: w1424 -> [w1429 w1432]
                  tunnel: w1423 -> [_ w1431]
                  tunnel: [w1429 w1430] -> w1422
                  frame False {
                  }
                  frame True {
                    n1236 = flat-sequence {
                      tunnel: [w1435] -> w1430
                      tunnel: w1432 -> [w1434]
                      tunnel: w1431 -> [w1433]
                      frame #0 {
                        n1237 = global read "CalibrationState.vi" "CalibrationState"() -> (w1436:T9)
                        n1238 = call "WriteCalibrationFile.vi"("error in (no error)"=w1434, "CalibrationState"=w1436, "Path"=w1433) -> ("error out"=w1435:errorcluster)  [unwired: 8 in]
                      }
                      frame #1 {
                        n1239 = local write "SaveCalibrationFile"(FALSE ("SaveCalibrationFile")) -> ()
                      }
                    }
                  }
                }
              }
            }
          }
          event "btnVidanger": Value Change {
            # "Possibilité de vidanger à tout moment"
            n1240 = event-data() -> ("NewVal"=w1440:bool)  [unwired: 1 in, 5 out]
            n1241 = case shown="True" w1440 {
              tunnel: w1439 -> [w1441 w1443]
              tunnel: [w1441 w1442] -> w1438
              frame False {
              }
              frame True {
                n1242 = stacked-sequence {
                  tunnel: w1443 -> [_ _ _ w1461 _ _]
                  tunnel: [_ _ _ w1460 _ _] -> w1442
                  frame #0 {
                    n1243 = property on="manualModeBtn" class="Bool (strict)"("Val(Sgnl)"=FALSE, "DisabledEnum"=T8."Disabled and Grayed Out" ("Disabled")) -> ()  [unwired: 2 in, 2 out]
                  }
                  frame #1 {
                    n1244 = global write "AppState.vi" "AppState"(u16 3 ("AppState")) -> ()
                  }
                  frame #2 {
                    w1454 = FALSE ("Value (Signaling)")
                    # "Efface/Affiche les contrôles nécessaires"
                    n1245 = global read "LanguagesSettings.vi" "LanguageSettings"() -> (w1450:T13)
                    n1246 = property on="CalibrationResultsVisible" class="Bool (strict)"("Val(Sgnl)"=w1454) -> ()  [unwired: 2 in, 2 out]
                    n1247 = property on="CalibrationButtonsVisible" class="Bool (strict)"("Val(Sgnl)"=w1454) -> ()  [unwired: 2 in, 2 out]
                    n1248 = property on="MeasureIndicatorsVisible" class="Bool (strict)"("Val(Sgnl)"=w1454) -> ()  [unwired: 2 in, 2 out]
                    n1249 = property on="MeasureSetupButtonsVisible" class="Bool (strict)"("Val(Sgnl)"=w1454) -> ()  [unwired: 2 in, 2 out]
                    n1250 = property on="ChangeMenuState" class="Bool (strict)"("Val(Sgnl)"=w1454) -> ()  [unwired: 2 in, 2 out]
                    n1251 = property on="ExportMeasuresButtonsVisible" class="Bool (strict)"("Val(Sgnl)"=w1454) -> ()  [unwired: 2 in, 2 out]
                    n1252 = Unbundle By Name(w1450) -> ("LocalisationFileContent[out]"=w1449:T21)
                    n1253 = local read "LanguagesList"() -> (w1453:i32)
                    n1254 = property on="PurgeState" class="Str"("Visible"=TRUE) -> ()  [unwired: 2 in, 2 out]
                    n1255 = call "FindLocalizedString.vi"("LangIndex"=w1453, "LocalizationFileContent"=w1449, "WordIndex"=u32 88) -> ("Found"=w1452:bool, "LocalizedString"=w1451:string)  [unwired: 7 in]
                    n1256 = case shown="True" w1452 {
                      tunnel: w1451 -> [_ w1457]
                      tunnel: ["Not found" w1457] -> w1447
                      frame False {
                      }
                      frame True {
                      }
                    }
                    n1257 = property on="PurgeState" class="Str"("Text.Text"=w1447) -> ()  [unwired: 2 in, 2 out]
                  }
                  frame #3 {
                    # "Effectue la vidange"
                    n1258 = local read "ReferenceCellMeasure"() -> (w1458:u16)
                    n1259 = call "DoPurge.vi"("error in (no error)"=w1461, "VrefUsed"=w1458) -> ("error out"=w1460:errorcluster, "StabilityAchieved"=w1459:bool)  [unwired: 7 in, 1 out]
                    n1260 = local write "StabilityAchieved"(w1459) -> ()
                  }
                  frame #4 {
                    # "Affiche le message de réussite, retransitionne vers l'état idle"
                    n1261 = global read "LanguagesSettings.vi" "LanguageSettings"() -> (w1462:T13)
                    n1262 = global write "AppState.vi" "AppState"(u16 0 ("AppState")) -> ()
                    n1263 = property on="manualModeBtn" class="Bool (strict)"("DisabledEnum"=T8."Enabled" ("Disabled")) -> ()  [unwired: 2 in, 2 out]
                    n1264 = Unbundle By Name(w1462) -> ("LocalisationFileContent[out]"=w1465:T21)
                    n1265 = local read "LanguagesList"() -> (w1468:i32)
                    n1266 = call "FindLocalizedString.vi"("LangIndex"=w1468, "LocalizationFileContent"=w1465, "WordIndex"=u32 87) -> ("Found"=w1467:bool, "LocalizedString"=w1466:string)  [unwired: 7 in]
                    n1267 = case shown="True" w1467 {
                      tunnel: w1466 -> [_ w1472]
                      tunnel: ["Not found" w1472] -> w1463
                      frame False {
                      }
                      frame True {
                      }
                    }
                    n1268 = property on="PurgeState" class="Str"("Text.Text"=w1463) -> ()  [unwired: 2 in, 2 out]
                  }
                  frame #5 {
                    n1269 = property on="ChangeMenuState" class="Bool (strict)"("Val(Sgnl)"=TRUE ("Value (Signaling)")) -> ()  [unwired: 2 in, 2 out]
                  }
                }
              }
            }
          }
          event "Pressure Offset", "Pressure Gain": Value Change {
            n1270 = event-data() -> ()  [unwired: 1 in, 6 out]
            n1271 = local read "Pressure Offset"() -> (w1477:dbl)
            n1272 = local read "Pressure Gain"() -> (w1476:dbl)
            n1273 = call "capt_scaling.vi"("error in"=w1475, "Gain"=w1476, "Offset"=w1477) -> ("error out"=w1474:errorcluster)  [unwired: 8 in]
          }
        }
        n1274 = local read "btnExit"() -> (w383:bool)
        n1275 = case shown="Error" w379 {
          tunnel: w379 -> [w384 w386]
          tunnel: [w384 errorcluster {"status"=FALSE, "code"=0, "source"=""} ("error in")] -> w380
          frame No Error {
          }
          frame Error {
            n1276 = local write "error out"(w386) -> ()
          }
        }
      }
      n1277 = while {
        shift-right: [w117] -> _
        shift-left: w116 -> [w119]
        stop <- w120 stop-if-true
        # "Boucle d'acquisition continue"
        n1278 = local read "btnExit"() -> (w120:bool)
        n1279 = call "ContinuousPressureAcquisition.vi"("error in"=w119) -> ("error out"=w118:errorcluster)  [unwired: 10 in]
        n1280 = case shown="Error" w118 {
          tunnel: [w121 errorcluster {"status"=FALSE, "code"=0, "source"=""} ("error in")] -> w117
          tunnel: w118 -> [w121 _]
          frame No Error {
          }
          frame Error {
          }
        }
      }
    }
    frame #2 {
      # "Nettoyage avant quittage"
      n1281 = global read "HardwarePresent.vi" "HardwarePresent"() -> (w1478:bool)
      n1282 = case shown="True" w1478 {
        frame False {
          n1283 = Stop() -> ()  [unwired: 1 in]
        }
        frame True {
          n1284 = Quit LabVIEW(quit? (T)=TRUE) -> ()
        }
      }
    }
  }
